vi "test_CRC-32 - Check Protection.vi"(8 "error in (no error)":errorcluster) -> (0 "error out":errorcluster)   [LabVIEW 2023, in "Instrument Addon Protections Unit Tests.lvclass"]
uses:
  Instrument Addon Protections Unit Tests.lvclass
  <vilib>/addons/_JKI Toolkits/VI Tester/TestCase.llb/TestCase.lvclass
  CRC-32/CRC-32.lvclass
panel:
  out "CRC-32 out":refnum<class "CRC-32.lvclass">
  in  "CRC-32 in":refnum<class "CRC-32.lvclass">
  out "TestCase out":refnum<class "Instrument Addon Protections Unit Tests.lvclass">
  in  "TestCase in":refnum<class "Instrument Addon Protections Unit Tests.lvclass">
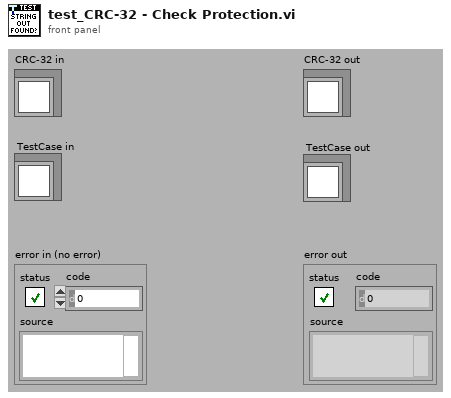
[diagram p1: front panel]
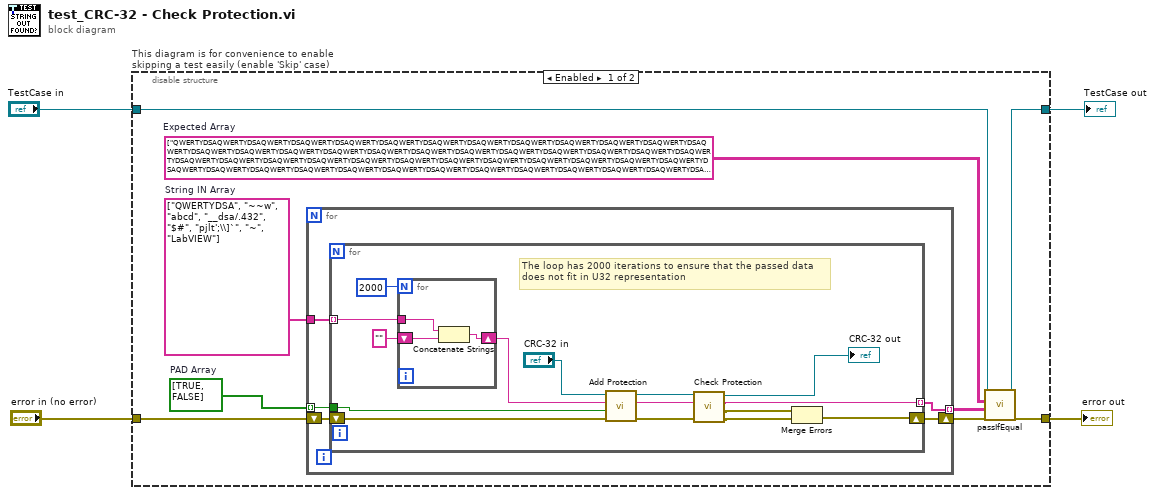
[diagram p0: block diagram]
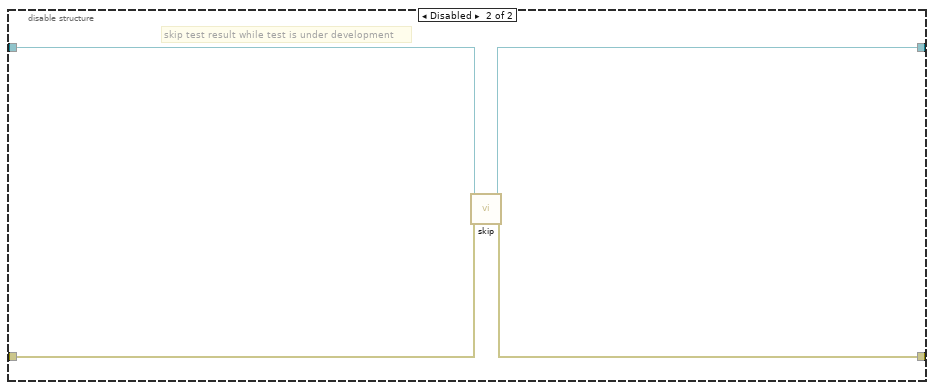
[diagram p2: hidden frame]
diagram:
  n1 = disable-structure "This diagram is for convenience to enable skipping a test easily (enable 'Skip' case)" shown="Enabled" {
    disable-tunnel: "TestCase in" -> [w11 w40]
    disable-tunnel: [w12 w38] -> w1
    disable-tunnel: [w13 w39] -> w3
    disable-tunnel: "error in (no error)" -> [w10 w37]
    frame Enabled {
      w5 = string[][] [["QWERTYDSAQWERTYDSAQWERTYDSAQWERTYDSAQWERTYDSAQWERTYDSAQWERTYDSAQWERTYDSAQWERTYDSAQWERTYDSAQWERTYDSAQWERTYDSAQWERTYDSAQWERTYDSAQWERTYDSAQWERTYDSAQWERTYDSAQWERTYDSAQWERTYDSAQWERTYDSAQWERTYDSAQWERTYDSAQWERTYDSAQWERTYDSAQWERTYDSAQWERTYDSAQWERTYDSAQWERTYDSAQWERTYDSAQWERTYDSAQWERTYDSAQWERTYDSAQWERTYDSAQWERTYDSAQWERTYDSAQWERTYDSAQWERTYDSAQWERTYDSAQWERTYDSAQWERTYDSAQWERTYDSAQWERTYDSAQWERTYDSAQWERTYDSAQWERTYDSAQWERTYDSAQWERTYDSAQWERTYDSAQWERTYDSAQWERTYDSAQWERTYDSAQWERTYDSAQWERTYDSAQWERTYDSAQWERTYDSAQWERTYDSAQWERTYDSAQWERTYDSAQWERTYDSAQWERTYDSAQWERTYDSAQWERTYDSAQWERTYDSAQWERTYDSAQWERTYDSAQWERTYDSAQWERTY...", "~~w~~w~~w~~w~~w~~w~~w~~w~~w~~w~~w~~w~~w~~w~~w~~w~~w~~w~~w~~w~~w~~w~~w~~w~~w~~w~~w~~w~~w~~w~~w~~w~~w~~w~~w~~w~~w~~w~~w~~w~~w~~w~~w~~w~~w~~w~~w~~w~~w~~w~~w~~w~~w~~w~~w~~w~~w~~w~~w~~w~~w~~w~~w~~w~~w~~w~~w~~w~~w~~w~~w~~w~~w~~w~~w~~w~~w~~w~~w~~w~~w~~w~~w~~w~~w~~w~~w~~w~~w~~w~~w~~w~~w~~w~~w~~w~~w~~w~~w~~w~~w~~w~~w~~w~~w~~w~~w~~w~~w~~w~~w~~w~~w~~w~~w~~w~~w~~w~~w~~w~~w~~w~~w~~w~~w~~w~~w~~w~~w~~w~~w~~w~~w~~w~~w~~w~~w~~w~~w~~w~~w~~w~~w~~w~~w~~w~~w~~w~~w~~w~~w~~w~~w~~w~~w~~w~~w~~w~~w~~w~~w~~w~~w~~w~~w~~w~~w~~w~~w~~w~~w~~w~~w~~w~~w~~w~~w~~w~~w~~w~~w~~w~~w~~w~~w~~w~~w~~w~~w~~w~~w~~w~~w~~w~~w~~w~~w~~w~~w~~w~~w~~w~~w~~w~~w~~w~~w~~w~~w~~w~~w~~w~~w~~w~~w~~w~~w~~w~~w~~w~~w~~w~~w~~w~~w~~w~~w~~w~~w~~w~~w~~w~~w~~w~~w~~w~~w~~w~~w~~w~~w~~w~~w~~w~~w~~w~~w~~w~~w~~w~~w~~w~~w~~w~~w~~w~~w~~w~~w~~w~~w~~w~~w~~w~~w~~w~~w~~w~~w~~w~~w~~w~~w~~w~~w~~w~~w~~w~~w~~w~~w~~w~~w~~w~~w~~w~~w~~w~~w~~w~~w~~w~~w~~w~~w~~w~~w~~w~~w~~w~~w~~w~~w~~w~~w~~w~~w~~w~~w~~w~~w~~w~~w~~w~~w~~w~~w~~w~~w~~w~~w~~w~~w~~w~~w~~w~~w~~w~~w~~w~~w~~w~~w~~w~~w~~w~~w~~w~~w~~w~~w~~w~~w~~w~~w~~w~~w~~w~~w~~w~~w~~w~~w~~w~~w~~w~~w~~w~~w~~w~~w~~w~~w~~w~~w~~w~~w~~w~~w~~w~~w~~w~~w~~w~~w~~w~~w~~w~~w~~w~~w~~w~~w~~w~~w~~w~~w~~w~~w~~w~~w~~w~~w~~w~~w~~w~~w~~w~~w~~w~~w~~w~~w~~w~~w~~w~~w~~w~~w~~w~~w~~w~~w~~w~~w~~w~~w~~w~~w~~w~~w~~w~~w~~w~~w~~w~~w~~w~~w~~w~~w~~w~~w~~w~~w~~w~~w~~w~~w~~w~~w~~w~~w~~w~~w~~w~~w~~w~~w~~w~~w~~w~~w~~w~~w~~w~~w~~w~~w~~w~~w~~w~~w~~w~~w~~w~~w~~w~~w~~w~~w~~w~~w~~w~~w~~w~~w~~w~~w~~w~~w~~w~~w~~w~~w~~w~~w~~w~~w~~w~~w~~w~~w~~w~~w~~w~~w~~w~~w~~w~~w~~w~~w~~w~~w~~w~~w~~w~~w~~w~~w~~w~~w~~w~~w~~w~~w~~w~~w~~w~~w~~w~~w~~w~~w~~w~~w~~w~~w~~w~~w~~w~~w~~w~~w~~w~~w~~w~~w~~w~~w~~w~~w~~w~~w~~w~~w~~w~~w~~w~~w~~w~~w~~w~~w~~w~~w~~w~~w~~w~~w~~w~~w~~w~~w~~w~~w~~w~~w~~w~~w~~w~~w~~w~~w~~w~~w~~w~~w~~w~~w~~w~~w~~w~~w~~w~~w~~w~~w~~w~~w~~w~~w~~w~~w~~w~~w~~w~~w~~w~~w~~w~~w~~w~~w~~w~~w~~w~~w~~w~~w~~w~~w~~w~~w~~w~~w~~w~~w~~w~~w~~w~~w~~w~~w~~w~~w~~w~~w~~w~~w~~w~~w~~w~~w~~w~~w~~w~~w~~w~~w~~w~~w~~w~~w~~w~~w~~w~~w~~w~~w~~w~~w~~w~~w~~w~~w~~w~~w~~w~~w~~w~~w~~w~~w~~w~~w~~w~~w~~w~~w~~w~~w~~w~~w~~w~~w~~w~~w~~w~~w~~w~~w~~w~~w~~w~~w~~w~~w~~w~~w~~w~~w~~w~~w~~w~~w~~w~~w~~w~~w~~w~~w~~w~~w~~w~~w~~w~~w~~w~~w~~w~~w~~w~~w~~w~~w~~w~~w~~w~~w~~w~~w~~w~~w~~w~~w~~w~~w~~w~~w~~w~~w~~w~~w~~w~~w~~w~~w~~w~~w~~w~~w~~w~~w~~w~~w~~w~~w~~w~~w~~w~~w~~w~~w~~w~~w~~w~~w~~w~~w~~w~~w~~w~~w~~w~~w~~w~~w~~w~~w~~w~~w~~w~~w~~w~~w~~w~~w~~w~~w~~w~~w~~w~~w~~w~~w~~w~~w~~w~~w~~w~~w~~w~~w~~w~~w~~w~~w~~w~~w~~w~~w~~w~~w~~w~~w~~w~~w~~w~~w~~w~~w~~w~~w~~w~~w~~w~~w~~w~~w~~w~~w~~w~~w~~w~~w~~w~~w~~w~~w~~w~~w~~w~~w~~w~~w~~w~~w~~w~~w~~w~~w~~w~~w~~w~~w~~w~~w~~w~~w~~w~~w~~w~~w~~w~~w~~w~~w~~w~~w~~w~~w~~w~~w~~w~~w~~w~~w~~w~~w~~w~~w~~w~~w~~w~~w~~w~~w~~w~~w~~w~~w~~w~~w~~w~~w~~w~~w~~w~~w~~w~~w~~w~~w~~w~~w~~w~~w~~w~~w~~w~~w~~w~~w~~w~~w~~w~~w~~w~~w~~w~~w~~w~~w~~w~~w~~w~~w~~w~~w~~w~~w~~w~~w~~w~~w~~w~~w~~w~~w~~w~~w~~w~~w~~w~~w~~w~~w~~w~~w~~w~~w~~w~~w~~w~~w~~w~~w~~w~~w~~w~~w~~w~~w~~w~~w~~w~~w~~w~~w~~w~~w~~w~~w~~w~~w~~w~~w~~w~~w~~w~~w~~w~~w~~w~~w~~w~~w~~w~~w~~w~~w~~w~~w~~w~~w~~w~~w~~w~~w~~w~~w~~w~~w~~w~~w~~w~~w~~w~~w~~w~~w~~w~~w~~w~~w~~w~~w~~w~~w~~w~~w~~w~~w~~w~~w~~w~~w~~w~~w~~w~~w~~w~~w~~w~~w~~w~~w~~w~~w~~w~~w~~w~~w~~w~~w~~w~~w~~w~~w~~w~~w~~w~~w~~w~~w~~w~~w~~w~~w~~w~~w~~w~~w~~w~~w~~w~~w~~w~~w~~w~~w~~w~~w~~w~~w~~w~~w~~w~~w~~w~~w~~w~~w~~w~~w~~w~~w~~w~~w~~w~~w~~w~~w~~w~~w~~w~~w~~w~~w~~w~~w~~w~~w~~w~~w~~w~~w~~w~~w~~w~~w~~w~~w~~w~~w~~w~~w~~w~~w~~w~~w~~w~~w~~w~~w~~w~~w~~w~~w~~w~~w~~w~~w~~w~~w~~w~~w~~w~~w~~w~~w~~w~~w~~w~~w~~w~~w~~w~~w~~w~~w~~w~~w~~w~~w~~w~~w~~w~~w~~w~~w~~w~~w~~w~~w~~w~~w~~w~~w~~w~~w~~w~~w~~w~~w~~w~~w~~w~~w~~w~~w~~w~~w~~w~~w~~w~~w~~w~~w~~w~~w~~w~~w~~w~~w~~w~~w~~w~~w~~w~~w~~w~~w~~w~~w~~w~~w~~w~~w~~w~~w~~w~~w~~w~~w~~w~~w~~w~~w~~w~~w~~w~~w~~w~~w~~w~~w~~w~~w~~w~~w~~w~~w~~w~~w~~w~~w~~w~~w~~w~~w~~w~~w~~w~~w~~w~~w~~w~~w~~w~~w~~w~~w~~w~~w~~w~~w~~w~~w~~w~~w~~w~~w~~w~~w~~w~~w~~w~~w~~w~~w~~w~~w~~w~~w~~w~~w~~w~~w~~w~~w~~w~~w~~w~~w~~w~~w~~w~~w~~w~~w~~w~~w~~w~~w~~w~~w~~w~~w~~w~~w~~w~~w~~w~~w~~w~~w~~w~~w~~w~~w~~w~~w~~w~~w~~w~~w~~w~~w~~w~~w~~w~~w~~w~~w~~w~~w~~w~~w~~w~~w~~w~~w~~w~~w~~w~~w~~w~~w~~w~~w~~w~~w~~w~~w~~w~~w~~w~~w~~w~~w~~w~~w~~w~~w~~w~~w~~w~~w~~w~~w~~w~~w~~w~~w~~w~~w~~w~~w~~w~~w~~w~~w~~w~~w~~w~~w~~w~~w~~w~~w~~w~~w~~w~~w~~w~~w~~w~~w~~w~~w~~w~~w~~w~~w~~w~~w~~w~~w~~w~~w~~w~~w~~w~~w~~w~~w~~w~~w~~w~~w~~w~~w~~w~~w~~w~~w~~w~~w~~w~~w~~w~~w~~w~~w~~w~~w~~w~~w~~w~~w~~w~~w~~w~~w~~w~~w~~w~~w~~w~~w~~w~~w~~w~~w~~w~~w~~w~~w~~w~~w~~w~~w~~w~~w~~w~~w~~w~~w~~w~~w~~w~~w~~w~~w~~w~~w~~w~~w~~w~~w~~w~~w~~w~~w~~w~~w~~w~~w~~w~~w~~w~~w~~w~~w~~w~~w~~w~~w~~w~~w~~w~~w~~w~~w~~w~~w~~w~~w~~w~~w~~w~~w~~w~~w~~w~~w~~w~~w~~w~~w~~w~~w~~w~~w~~w~~w~~w~~w~~w~~w~~w~~w~~w~~w~~w~~w~~w~~w~~w~~w~~w~~w~~w~~w~~w~~w~~w~~w~~w~~w~~w~~w~~w~~w~~w~~w~~w~~w~~w~~w~~w~~w~~w~~w~~w~~w~~w~~w~~w~~w~~w~~w~~w~~w~~w~~w~~w~~w~~w~~w~~w~~w~~w~~w~~w~~w~~w~~w~~w~~w~~w~~w~~w~~w~~w~~w~~w~~w~~w~~w~~w~~w~~w~~w~~w~~w~~w~~w~~w~~w~~w~~w~~w~~w~~w~~w~~w~~w~~w~~w~~w~~w~~w~~w~~w~~w~~w~~w~~w~~w~~w~~w~~w~~w~~w~~w~~w~~w~~w~~w~~w~~w~~w~~w~~w~~w~~w~~w~~w~~w~~w~~w~~w~~w~~w~~w~~w~~w~~w~~w~~w~~w~~w~~w~~w~~w~~w~~w~~w~~w~~w~~w~~w~~w~~w~~w~~w~~w~~w~~w~~w~~w~~w~~w~~w~~w~~w~~w~~w~~w~~w~~w~~w~~w~~w~~w~~w~~w~~w~~w~~w~~w~~w~~w~~w~~w~~w~~w~~w~~w~~w~~w~~w~~w~~w~~w~~w~~w~~w~~w~~w~~w~~w~~w~~w~~w~~w~~w~~w~~w~~w~~w~~w~~w~~w~~w~~w~~w~~w~~w~~w~~w~~w~~w~~w~~w~~w~~w~~w~~w~~w~~w~~w~~w~~w~~w~~w~~w~~w~~w~~w~~w~~w~~w~~w~~w~~w~~w~~w~~w~~w~~w~~w~~w~~w~~w~~w~~w~~w~~w~~w~~w~~w~~w~~w~~w~~w~~w~~w~~w~~w~~w~~w~~w~~w~~w~~w~~w~~w~~w~~w~~w~~w~~w~~w~~w~~w~~w~~w~~w~~w~~w~~w~~w~~w~~w~~w~~w~~w~~w~~w~~w~~w~~w~~w~~w~~w~~w~~w~~w~~w~~w~~w~~w~~w~~w~~w~~w~~w~~w~~w~~w~~w~~w~~w~~w~~w~~w~~w~~w~~w~~w~~w~~w~~w~~w~~w~~w~~w~~w~~w~~w~~w~~w~~w~~w~~w~~w~~w~~w~~w~~w~~w~~w~~w~~w~~w~~w~~w~~w~~w~~w~~w~~w~~w~~w~~w~~w~~w~~w~~w~~w~~w~~w~~w~~w~~w~~w~~w~~w~~w~~w~~w~~w~~w~~w~~w~~w~~w~~w~~w~~w~~w~~w~~w~~w~~w~~w~~w~~w~~w~~w~~w~~w~~w~~w~~w~~w~~w~~w~~w~~w~~w~~w~~w~~w~~w~~w~~w~~w~~w~~w~~w~~w~~w~~w~~w~~w~~w~~w~~w~~w~~w~~w~~w~~w~~w~~w~~w~~w~~w~~w~~w~~w~~w~~w~~w~~w~~w~~w~~w~~w~~w~~w~~w~~w~~w~~w~~w~~w~~w~~w~~w~~w~~w~~w~~w~~w~~w~~w~~w~~w~~w~~w~~w~~w~~w~~w~~w~~w~~w~~w~~w~~w~~w~~w~~w~~w~~w~~w~~w~~w~~w~~w~~w~~", "abcdabcdabcdabcdabcdabcdabcdabcdabcdabcdabcdabcdabcdabcdabcdabcdabcdabcdabcdabcdabcdabcdabcdabcdabcdabcdabcdabcdabcdabcdabcdabcdabcdabcdabcdabcdabcdabcdabcdabcdabcdabcdabcdabcdabcdabcdabcdabcdabcdabcdabcdabcdabcdabcdabcdabcdabcdabcdabcdabcdabcdabcdabcdabcdabcdabcdabcdabcdabcdabcdabcdabcdabcdabcdabcdabcdabcdabcdabcdabcdabcdabcdabcdabcdabcdabcdabcdabcdabcdabcdabcdabcdabcdabcdabcdabcdabcdabcdabcdabcdabcdabcdabcdabcdabcdabcdabcdabcdabcdabcdabcdabcdabcdabcdabcdabcdabcdabcdabcdabcdabcdabcdabcdabcdabcdabcdabcdabcdabcdabcdabcdabcdabcdabcdabcdabcdabcdabcdabcdabcdabcdabcdabcdabcdabcdabcdabcdabcdabcdabcd...", "__dsa/.432__dsa/.432__dsa/.432__dsa/.432__dsa/.432__dsa/.432__dsa/.432__dsa/.432__dsa/.432__dsa/.432__dsa/.432__dsa/.432__dsa/.432__dsa/.432__dsa/.432__dsa/.432__dsa/.432__dsa/.432__dsa/.432__dsa/.432__dsa/.432__dsa/.432__dsa/.432__dsa/.432__dsa/.432__dsa/.432__dsa/.432__dsa/.432__dsa/.432__dsa/.432__dsa/.432__dsa/.432__dsa/.432__dsa/.432__dsa/.432__dsa/.432__dsa/.432__dsa/.432__dsa/.432__dsa/.432__dsa/.432__dsa/.432__dsa/.432__dsa/.432__dsa/.432__dsa/.432__dsa/.432__dsa/.432__dsa/.432__dsa/.432__dsa/.432__dsa/.432__dsa/.432__dsa/.432__dsa/.432__dsa/.432__dsa/.432__dsa/.432__dsa/.432__dsa/.432__dsa/.432__dsa/.432__dsa/.432__dsa/.432__dsa/.432__dsa/.432__dsa/.432__dsa/.432__dsa/.432__dsa/.432__dsa/.432__dsa/.432__dsa/.432__dsa/.432__dsa/.432__dsa/.432__dsa/.432__dsa/.432__dsa/.432__dsa/.432__dsa/.432__dsa/.432__dsa/.432__dsa/.432__dsa/.432__dsa/.432__dsa/.432__dsa/.432__dsa/.432__dsa/.432__dsa/.432__dsa/.432__dsa/.432__dsa/.432__dsa/.432__dsa/.432__dsa/.432__dsa/.432__dsa/.432__dsa/.432__dsa/.432__dsa/.432__dsa/.432__dsa/.432__dsa/.432__dsa/.432__dsa/.432__dsa/.432__dsa/.432__dsa/.432__dsa/.432__dsa/.432__dsa/.432__dsa/.432__dsa/.432__dsa/.432__dsa/.432__dsa/.432__dsa/.432__dsa/.432__dsa/.432__dsa/.432__dsa/.432__dsa/.432__dsa/.432__dsa/.432__dsa/.432__dsa/.432__dsa/.432__dsa/.432__dsa/.432__dsa/.432__dsa/.432__dsa/.432__dsa/.432__dsa/.432__dsa/.432__dsa/.432__dsa/.432__dsa/.432__dsa/.432__dsa/.432__dsa/.432__dsa/.432__dsa/.432__dsa/.432__dsa/.432__dsa/.432__dsa/.432__dsa/.432__dsa/.432__dsa/.432__dsa/.432__dsa/.432__dsa/.432__dsa/.432__dsa/.432__dsa/.432__dsa/.432__dsa/.432__dsa/.432__dsa/.432__dsa/.432__dsa/.432__dsa/.432__dsa/.432__dsa/.432__dsa/.432__dsa/.432__dsa/.432__dsa/.432__dsa/.432__dsa/.432__dsa/.432__dsa/.432__dsa/.432__dsa/.432__dsa/.432__dsa/.432__dsa/.432__dsa/.432__dsa/.432__dsa/.432__dsa/.432__dsa/.432__dsa/.432__dsa/.432__dsa/.432__dsa/.432__dsa/.432__dsa/.432__dsa/.432__dsa/.432__dsa/.432__dsa/.432__dsa/.432__dsa/.432__dsa/.432__dsa/.432__dsa/.432__dsa/.432__dsa/.432__dsa/.432__dsa/.432__dsa/.432__dsa/.432__dsa/.432__dsa/.432__dsa/.432__dsa/.432__dsa/.432__dsa/.432__dsa/.432__dsa/.432__dsa/.432__dsa/.432__dsa/.432__dsa/.432__dsa/.432__dsa/.432__dsa/.432__dsa/.432__dsa/.432__dsa/.432__dsa/.432__dsa/.432__dsa/.432__dsa/.432__dsa/.432__dsa/.432__dsa/.432__dsa/.432__dsa/.432__dsa/.432__dsa/.432__dsa/.432__dsa/.432__dsa/.432__dsa/.432__dsa/.432__dsa/.432__dsa/.432__dsa/.432__dsa/.432__dsa/.432__dsa/.432__dsa/.432__dsa/.432__dsa/.432__dsa/.432__dsa/.432__dsa/.432__dsa/.432__dsa/.432__dsa/.432__dsa/.432__dsa/.432__dsa/.432__dsa/.432__dsa/.432__dsa/.432__dsa/.432__dsa/.432__dsa/.432__dsa/.432__dsa/.432__dsa/.432__dsa/.432__dsa/.432__dsa/.432__dsa/.432__dsa/.432__dsa/.432__dsa/.432__dsa/.432__dsa/.432__dsa/.432__dsa/.432__dsa/.432__dsa/.432__dsa/.432__dsa/.432__dsa/.432__dsa/.432__dsa/.432__dsa/.432__dsa/.432__dsa/.432__dsa/.432__dsa/.432__dsa/.432__dsa/.432__dsa/.432__dsa/.432__dsa/.432__dsa/.432__dsa/.432__dsa/.432__dsa/.432__dsa/.432__dsa/.432__dsa/.432__dsa/.432__dsa/.432__dsa/.432__dsa/.432__dsa/.432__dsa/.432__dsa/.432__dsa/.432__dsa/.432__dsa/.432__dsa/.432__dsa/.432__dsa/.432__dsa/.432__dsa/.432__dsa/.432__dsa/.432__dsa/.432__dsa/.432__dsa/.432__dsa/.432__dsa/.432__dsa/.432__dsa/.432__dsa/.432__dsa/.432__dsa/.432__dsa/.432__dsa/.432__dsa/.432__dsa/.432__dsa/.432__dsa/.432__dsa/.432__dsa/.432__dsa/.432__dsa/.432__dsa/.432__dsa/.432__dsa/.432__dsa/.432__dsa/.432__dsa/.432__dsa/.432__dsa/.432__dsa/.432__dsa/.432__dsa/.432__dsa/.432__dsa/.432__dsa/.432__dsa/.432__dsa/.432__dsa/.432__dsa/.432__dsa/.432__dsa/.432__dsa/.432__dsa/.432__dsa/.432__dsa/.432__dsa/.432__dsa/.432__dsa/.432__dsa/.432__dsa/.432__dsa/.432__dsa/.432__dsa/.432__dsa/.432__dsa/.432__dsa/.432__dsa/.432__dsa/.432__dsa/.432__dsa/.432__dsa/.432__dsa/.432__dsa/.432__dsa/.432__dsa/.432__dsa/.432__dsa/.432__dsa/.432__dsa/.432__dsa/.432__dsa/.432__dsa/.432__dsa/.432__dsa/.432__dsa/.432__dsa/.432__dsa/.432__dsa/.432__dsa/.432__dsa/.432__dsa/.432__dsa/.432__dsa/.432__dsa/.432__dsa/.432__dsa/.432__dsa/.432__dsa/.432__dsa/.432__dsa/.432__dsa/.432__dsa/.432__dsa/.432__dsa/.432__dsa/.432__dsa/.432__dsa/.432__dsa/.432__dsa/.432__dsa/.432__dsa/.432__dsa/.432__dsa/.432__dsa/.432__dsa/.432__dsa/.432__dsa/.432__dsa/.432__dsa/.432__dsa/.432__dsa/.432__dsa/.432__dsa/.432__dsa/.432__dsa/.432__dsa/.432__dsa/.432__dsa/.432__dsa/.432__dsa/.432__dsa/.432__dsa/.432__dsa/.432__dsa/.432__dsa/.432__dsa/.432__dsa/.432__dsa/.432__dsa/.432__dsa/.432__dsa/.432__dsa/.432__dsa/.432__dsa/.432__dsa/.432__dsa/.432__dsa/.432__dsa/.432__dsa/.432__dsa/.432__dsa/.432__dsa/.432__dsa/.432__dsa/.432__dsa/.432__dsa/.432__dsa/.432__dsa/.432__dsa/.432__dsa/.432__dsa/.432__dsa/.432__dsa/.432__dsa/.432__dsa/.432__dsa/.432__dsa/.432__dsa/.432__dsa/.432__dsa/.432__dsa/.432__dsa/.432__dsa/.432__dsa/.432__dsa/.432__dsa/.432__dsa/.432__dsa/.432__dsa/.432__dsa/.432__dsa/.432__dsa/.432__dsa/.432__dsa/.432__dsa/.432__dsa/.432__dsa/.432__dsa/.432__dsa/.432__dsa/.432__dsa/.432__dsa/.432__dsa/.432__dsa/.432__dsa/.432__dsa/.432__dsa/.432__dsa/.432__dsa/.432__dsa/.432__dsa/.432__dsa/.432__dsa/.432__dsa/.432__dsa/.432__dsa/.432__dsa/.432__dsa/.432__dsa/.432__dsa/.432__dsa/.432__dsa/.432__dsa/.432__dsa/.432__dsa/.432__dsa/.432__dsa/.432__dsa/.432__dsa/.432__dsa/.432__dsa/.432__dsa/.432__dsa/.432__dsa/.432__dsa/.432__dsa/.432__dsa/.432__dsa/.432__dsa/.432__dsa/.432__dsa/.432__dsa/.432__dsa/.432__dsa/.432__dsa/.432__dsa/.432__dsa/.432__dsa/.432__dsa/.432__dsa/.432__dsa/.432__dsa/.432__dsa/.432__dsa/.432__dsa/.432__dsa/.432__dsa/.432__dsa/.432__dsa/.432__dsa/.432__dsa/.432__dsa/.432__dsa/.432__dsa/.432__dsa/.432__dsa/.432__dsa/.432__dsa/.432__dsa/.432__dsa/.432__dsa/.432__dsa/.432__dsa/.432__dsa/.432__dsa/.432__dsa/.432__dsa/.432__dsa/.432__dsa/.432__dsa/.432__dsa/.432__dsa/.432__dsa/.432__dsa/.432__dsa/.432__dsa/.432__dsa/.432__dsa/.432__dsa/.432__dsa/.432__dsa/.432__dsa/.432__dsa/.432__dsa/.432__dsa/.432__dsa/.432__dsa/.432__dsa/.432__dsa/.432__dsa/.432__dsa/.432__dsa/.432__dsa/.432__dsa/.432__dsa/.432__dsa/.432__dsa/.432__dsa/.432__dsa/.432__dsa/.432__dsa/.432__dsa/.432__dsa/.432__dsa/.432__dsa/.432__dsa/.432__dsa/.432__dsa/.432__dsa/.432__dsa/.432__dsa/.432__dsa/.432__dsa/.432__dsa/.432__dsa/.432__dsa/.432__dsa/.432__dsa/.432__dsa/.432__dsa/.432__dsa/.432__dsa/.432__dsa/.432__dsa/.432__dsa/.432__dsa/.432__dsa/.432__dsa/.432__dsa/.432__dsa/.432__dsa/.432__dsa/.432__dsa/.432__dsa/.432__dsa/.432__dsa/.432__dsa/.432__dsa/.432__dsa/.432__dsa/.432__dsa/.432__dsa/.432__dsa/.432__dsa/.432__dsa/.432__dsa/.432__dsa/.432__dsa/.432__dsa/.432__dsa/.432__dsa/.432__dsa/.432__dsa/.432__dsa/.432__dsa/.432__dsa/.432__dsa/.432__dsa/.432__dsa/.432__dsa/.432__dsa/.432__dsa/.432__dsa/.432__dsa/.432__dsa/.432__dsa/.432__dsa/.432__dsa/.432__dsa/.432__dsa/.432__dsa/.432__dsa/.432__dsa/.432__dsa/.432__dsa/.432__dsa/.432__dsa/.432__dsa/.432__dsa/.432__dsa/.432__dsa/.432__dsa/.432__dsa/.432__dsa/.432__dsa/.432__dsa/.432__dsa/.432__dsa/.432__dsa/.432__dsa/.432__dsa/.432__dsa/.432__dsa/.432__dsa/.432__dsa/.432__dsa/.432__dsa/.432__dsa/.432__dsa/.432__dsa/.432__dsa/.432__dsa/.432__dsa/.432__dsa/.432__dsa/.432__dsa/.432__dsa/.432__dsa/.432__dsa/.432__dsa/.432__dsa/.432__dsa/.432__dsa/.432__dsa/.432__dsa/.432__dsa/.432__dsa/.432__dsa/.432__dsa/.432__dsa/.432__dsa/.432__dsa/.432__dsa/.432__dsa/.432__dsa/.432__dsa/.432__dsa/.432__dsa/.432__dsa/.432__dsa/.432__dsa/.432__dsa/.432__dsa/.432__dsa/.432__dsa/.432__dsa/.432__dsa/.432__dsa/.432__dsa/.432__dsa/.432__dsa/.432__dsa/.432__dsa/.432__dsa/.432__dsa/.432__dsa/.432__dsa/.432__dsa/.432__dsa/.432__dsa/.432__dsa/.432__dsa/.432__dsa/.432__dsa/.432__dsa/.432__dsa/.432__dsa/.432__dsa/.432__dsa/.432__dsa/.432__dsa/.432__dsa/.432__dsa/.432__dsa/.432__dsa/.432__dsa/.432__dsa/.432__dsa/.432__dsa/.432__dsa/.432__dsa/.432__dsa/.432__dsa/.432__dsa/.432__dsa/.432__dsa/.432__dsa/.432__dsa/.432__dsa/.432__dsa/.432__dsa/.432__dsa/.432__dsa/.432__dsa/.432__dsa/.432__dsa/.432__dsa/.432__dsa/.432__dsa/.432__dsa/.432__dsa/.432__dsa/.432__dsa/.432__dsa/.432__dsa/.432__dsa/.432__dsa/.432__dsa/.432__dsa/.432__dsa/.432__dsa/.432__dsa/.432__dsa/.432__dsa/.432__dsa/.432__dsa/.432__dsa/.432__dsa/.432__dsa/.432__dsa/.432__dsa/.432__dsa/.432__dsa/.432__dsa/.432__dsa/.432__dsa/.432__dsa/.432__dsa/.432__dsa/.432__dsa/.432__dsa/.432__dsa/.432__dsa/.432__dsa/.432__dsa/.432__dsa/.432__dsa/.432__dsa/.432__dsa/.432__dsa/.432__dsa/.432__dsa/.432__dsa/.432__dsa/.432__dsa/.432__dsa/.432__dsa/.432__dsa/.432__dsa/.432__dsa/.432__dsa/.432__dsa/.432__dsa/.432__dsa/.432__dsa/.432__dsa/.432__dsa/.432__dsa/.432__dsa/.432__dsa/.432__dsa/.432__dsa/.432__dsa/.432__dsa/.432__dsa/.432__dsa/.432__dsa/.432__dsa/.432__dsa/.432__dsa/.432__dsa/.432__dsa/.432__dsa/.432__dsa/.432__dsa/.432__dsa/.432__dsa/.432__dsa/.432__dsa/.432__dsa/.432__dsa/.432__dsa/.432__dsa/.432__dsa/.432__dsa/.432__dsa/.432__dsa/.432__dsa/.432__dsa/.432__dsa/.432__dsa/.432__dsa/.432__dsa/.432__dsa/.432__dsa/.432__dsa/.432__dsa/.432__dsa/.432__dsa/.432__dsa/.432__dsa/.432__dsa/.432__dsa/.432__dsa/.432__dsa/.432__dsa/.432__dsa/.432__dsa/.432__dsa/.432__dsa/.432__dsa/.432__dsa/.432__dsa/.432__dsa/.432__dsa/.432__dsa/.432__dsa/.432__dsa/.432__dsa/.432__dsa/.432__dsa/.432__dsa/.432__dsa/.432__dsa/.432__dsa/.432__dsa/.432__dsa/.432__dsa/.432__dsa/.432__dsa/.432__dsa/.432__dsa/.432__dsa/.432__dsa/.432__dsa/.432__dsa/.432__dsa/.432__dsa/.432__dsa/.432__dsa/.432__dsa/.432__dsa/.432__dsa/.432__dsa/.432__dsa/.432__dsa/.432__dsa/.432__dsa/.432__dsa/.432__dsa/.432__dsa/.432__dsa/.432__dsa/.432__dsa/.432__dsa/.432__dsa/.432__dsa/.432__dsa/.432__dsa/.432__dsa/.432__dsa/.432__dsa/.432__dsa/.432__dsa/.432__dsa/.432__dsa/.432__dsa/.432__dsa/.432__dsa/.432__dsa/.432__dsa/.432__dsa/.432__dsa/.432__dsa/.432__dsa/.432__dsa/.432__dsa/.432__dsa/.432__dsa/.432__dsa/.432__dsa/.432__dsa/.432__dsa/.432__dsa/.432__dsa/.432__dsa/.432__dsa/.432__dsa/.432__dsa/.432__dsa/.432__dsa/.432__dsa/.432__dsa/.432__dsa/.432__dsa/.432__dsa/.432__dsa/.432__dsa/.432__dsa/.432__dsa/.432__dsa/.432__dsa/.432__dsa/.432__dsa/.432__dsa/.432__dsa/.432__dsa/.432__dsa/.432__dsa/.432__dsa/.432__dsa/.432__dsa/.432__dsa/.432__dsa/.432__dsa/.432__dsa/.432__dsa/.432__dsa/.432__dsa/.432__dsa/.432__dsa/.432__dsa/.432__dsa/.432__dsa/.432__dsa/.432__dsa/.432__dsa/.432__dsa/.432__dsa/.432__dsa/.432__dsa/.432__dsa/.432__dsa/.432__dsa/.432__dsa/.432__dsa/.432__dsa/.432__dsa/.432__dsa/.432__dsa/.432__dsa/.432__dsa/.432__dsa/.432__dsa/.432__dsa/.432__dsa/.432__dsa/.432__dsa/.432__dsa/.432__dsa/.432__dsa/.432__dsa/.432__dsa/.432__dsa/.432__dsa/.432__dsa/.432__dsa/.432__dsa/.432__dsa/.432__dsa/.432__dsa/.432__dsa/.432__dsa/.432__dsa/.432__dsa/.432__dsa/.432__dsa/.432__dsa/.432__dsa/.432__dsa/.432__dsa/.432__dsa/.432__dsa/.432__dsa/.432__dsa/.432__dsa/.432__dsa/.432__dsa/.432__dsa/.432__dsa/.432__dsa/.432__dsa/.432__dsa/.432__dsa/.432__dsa/.432__dsa/.432__dsa/.432__dsa/.432__dsa/.432__dsa/.432__dsa/.432__dsa/.432__dsa/.432__dsa/.432__dsa/.432__dsa/.432__dsa/.432__dsa/.432__dsa/.432__dsa/.432__dsa/.432__dsa/.432__dsa/.432__dsa/.432__dsa/.432__dsa/.432__dsa/.432__dsa/.432__dsa/.432__dsa/.432__dsa/.432__dsa/.432__dsa/.432__dsa/.432__dsa/.432__dsa/.432__dsa/.432__dsa/.432__dsa/.432__dsa/.432__dsa/.432__dsa/.432__dsa/.432__dsa/.432__dsa/.432__dsa/.432__dsa/.432__dsa/.432__dsa/.432__dsa/.432__dsa/.432__dsa/.432__dsa/.432__dsa/.432__dsa/.432__dsa/.432__dsa/.432__dsa/.432__dsa/.432__dsa/.432__dsa/.432__dsa/.432__dsa/.432__dsa/.432__dsa/.432__dsa/.432__dsa/.432__dsa/.432__dsa/.432__dsa/.432__dsa/.432__dsa/.432__dsa/.432__dsa/.432__dsa/.432__dsa/.432__dsa/.432__dsa/.432__dsa/.432__dsa/.432__dsa/.432__dsa/.432__dsa/.432__dsa/.432__dsa/.432__dsa/.432__dsa/.432__dsa/.432__dsa/.432__dsa/.432__dsa/.432__dsa/.432__dsa/.432__dsa/.432__dsa/.432__dsa/.432__dsa/.432__dsa/.432__dsa/.432__dsa/.432__dsa/.432__dsa/.432__dsa/.432__dsa/.432__dsa/.432__dsa/.432__dsa/.432__dsa/.432__dsa/.432__dsa/.432__dsa/.432__dsa/.432__dsa/.432__dsa/.432__dsa/.432__dsa/.432__dsa/.432__dsa/.432__dsa/.432__dsa/.432__dsa/.432__dsa/.432__dsa/.432__dsa/.432__dsa/.432__dsa/.432__dsa/.432__dsa/.432__dsa/.432__dsa/.432__dsa/.432__dsa/.432__dsa/.432__dsa/.432__dsa/.432__dsa/.432__dsa/.432__dsa/.432__dsa/.432__dsa/.432__dsa/.432__dsa/.432__dsa/.432__dsa/.432__dsa/.432__dsa/.432__dsa/.432__dsa/.432__dsa/.432__dsa/.432__dsa/.432__dsa/.432__dsa/.432__dsa/.432__dsa/.432__dsa/.432__dsa/.432__dsa/.432__dsa/.432__dsa/.432__dsa/.432__dsa/.432__dsa/.432__dsa/.432__dsa/.432__dsa/.432__dsa/.432__dsa/.432__dsa/.432__dsa/.432__dsa/.432__dsa/.432__dsa/.432__dsa/.432__dsa/.432__dsa/.432__dsa/.432__dsa/.432__dsa/.432__dsa/.432__dsa/.432__dsa/.432__dsa/.432__dsa/.432__dsa/.432__dsa/.432__dsa/.432__dsa/.432__dsa/.432__dsa/.432__dsa/.432__dsa/.432__dsa/.432__dsa/.432__dsa/.432__dsa/.432__dsa/.432__dsa/.432__dsa/.432__dsa/.432__dsa/.432__dsa/.432__dsa/.432__dsa/.432__dsa/.432__dsa/.432__dsa/.432__dsa/.432__dsa/.432__dsa/.432__dsa/.432__dsa/.432__dsa/.432__dsa/.432__dsa/.432__dsa/.432__dsa/.432__dsa/.432__dsa/.432__dsa/.432__dsa/.432__dsa/.432__dsa/.432__dsa/.432__dsa/.432__dsa/.432__dsa/.432__dsa/.432__dsa/.432__dsa/.432__dsa/.432__dsa/.432__dsa/.432__dsa/.432__dsa/.432__dsa/.432__dsa/.432__dsa/.432__dsa/.432__dsa/.432__dsa/.432__dsa/.432__dsa/.432__dsa/.432__dsa/.432__dsa/.432__dsa/.432__dsa/.432__dsa/.432__dsa/.432__dsa/.432__dsa/.432__dsa/.432__dsa/.432__dsa/.432__dsa/.432__dsa/.432__dsa/.432__dsa/.432__dsa/.432__dsa/.432__dsa/.432__dsa/.432__dsa/.432__dsa/.432__dsa/.432__dsa/.432__dsa/.432__dsa/.432__dsa/.432__dsa/.432__dsa/.432__dsa/.432__dsa/.432__dsa/.432__dsa/.432__dsa/.432__dsa/.432__dsa/.432__dsa/.432__dsa/.432__dsa/.432__dsa/.432__dsa/.432__dsa/.432__dsa/.432__dsa/.432__dsa/.432__dsa/.432__dsa/.432__dsa/.432__dsa/.432__dsa/.432__dsa/.432__dsa/.432__dsa/.432__dsa/.432__dsa/.432__dsa/.432__dsa/.432__dsa/.432__dsa/.432__dsa/.432__dsa/.432__dsa/.432__dsa/.432__dsa/.432__dsa/.432__dsa/.432__dsa/.432__dsa/.432__dsa/.432__dsa/.432__dsa/.432__dsa/.432__dsa/.432__dsa/.432__dsa/.432__dsa/.432__dsa/.432__dsa/.432__dsa/.432__dsa/.432__dsa/.432__dsa/.432__dsa/.432__dsa/.432__dsa/.432__dsa/.432__dsa/.432__dsa/.432__dsa/.432__dsa/.432__dsa/.432__dsa/.432__dsa/.432__dsa/.432__dsa/.432__dsa/.432__dsa/.432__dsa/.432__dsa/.432__dsa/.432__dsa/.432__dsa/.432__dsa/.432__dsa/.432__dsa/.432__dsa/.432__dsa/.432__dsa/.432__dsa/.432__dsa/.432__dsa/.432__dsa/.432__dsa/.432__dsa/.432__dsa/.432__dsa/.432__dsa/.432__dsa/.432__dsa/.432__dsa/.432__dsa/.432__dsa/.432__dsa/.432__dsa/.432__dsa/.432__dsa/.432__dsa/.432__dsa/.432__dsa/.432__dsa/.432__dsa/.432__dsa/.432__dsa/.432__dsa/.432__dsa/.432__dsa/.432__dsa/.432__dsa/.432__dsa/.432__dsa/.432__dsa/.432__dsa/.432__dsa/.432__dsa/.432__dsa/.432__dsa/.432__dsa/.432__dsa/.432__dsa/.432__dsa/.432__dsa/.432__dsa/.432__dsa/.432__dsa/.432__dsa/.432__dsa/.432__dsa/.432__dsa/.432__dsa/.432__dsa/.432__dsa/.432__dsa/.432__dsa/.432__dsa/.432__dsa/.432__dsa/.432__dsa/.432__dsa/.432__dsa/.432__dsa/.432__dsa/.432__dsa/.432__dsa/.432__dsa/.432__dsa/.432__dsa/.432__dsa/.432__dsa/.432__dsa/.432__dsa/.432__dsa/.432__dsa/.432__dsa/.432__dsa/.432__dsa/.432__dsa/.432__dsa/.432__dsa/.432__dsa/.432__dsa/.432__dsa/.432__dsa/.432__dsa/.432__dsa/.432__dsa/.432__dsa/.432__dsa/.432__dsa/.432__dsa/.432__dsa/.432__dsa/.432__dsa/.432__dsa/.432__dsa/.432__dsa/.432__dsa/.432__dsa/.432__dsa/.432__dsa/.432__dsa/.432__dsa/.432__dsa/.432__dsa/.432__dsa/.432__dsa/.432__dsa/.432__dsa/.432__dsa/.432__dsa/.432__dsa/.432__dsa/.432__dsa/.432__dsa/.432__dsa/.432__dsa/.432__dsa/.432__dsa/.432__dsa/.432__dsa/.432__dsa/.432__dsa/.432__dsa/.432__dsa/.432__dsa/.432__dsa/.432__dsa/.432__dsa/.432__dsa/.432__dsa/.432__dsa/.432__dsa/.432__dsa/.432__dsa/.432__dsa/.432__dsa/.432__dsa/.432__dsa/.432__dsa/.432__dsa/.432__dsa/.432__dsa/.432__dsa/.432__dsa/.432__dsa/.432__dsa/.432__dsa/.432__dsa/.432__dsa/.432__dsa/.432__dsa/.432__dsa/.432__dsa/.432__dsa/.432__dsa/.432__dsa/.432__dsa/.432__dsa/.432__dsa/.432__dsa/.432__dsa/.432__dsa/.432__dsa/.432__dsa/.432__dsa/.432__dsa/.432__dsa/.432__dsa/.432__dsa/.432__dsa/.432__dsa/.432__dsa/.432__dsa/.432__dsa/.432__dsa/.432__dsa/.432__dsa/.432__dsa/.432__dsa/.432__dsa/.432__dsa/.432__dsa/.432__dsa/.432__dsa/.432__dsa/.432__dsa/.432__dsa/.432__dsa/.432__dsa/.432__dsa/.432__dsa/.432__dsa/.432__dsa/.432__dsa/.432__dsa/.432__dsa/.432__dsa/.432__dsa/.432__dsa/.432__dsa/.432__dsa/.432__dsa/.432__dsa/.432__dsa/.432__dsa/.432__dsa/.432__dsa/.432__dsa/.432__dsa/.432__dsa/.432__dsa/.432__dsa/.432__dsa/.432__dsa/.432__dsa/.432__dsa/.432__dsa/.432__dsa/.432__dsa/.432__dsa/.432__dsa/.432__dsa/.432__dsa/.432__dsa/.432__dsa/.432__dsa/.432__dsa/.432__dsa/.432__dsa/.432__dsa/.432__dsa/.432__dsa/.432__dsa/.432__dsa/.432__dsa/.432__dsa/.432__dsa/.432__dsa/.432__dsa/.432__dsa/.432__dsa/.432__dsa/.432__dsa/.432__dsa/.432__dsa/.432__dsa/.432__dsa/.432__dsa/.432__dsa/.432__dsa/.432__dsa/.432__dsa/.432__dsa/.432__dsa/.432__dsa/.432__dsa/.432__dsa/.432__dsa/.432__dsa/.432__dsa/.432__dsa/.432__dsa/.432__dsa/.432__dsa/.432__dsa/.432__dsa/.432__dsa/.432__dsa/.432__dsa/.432__dsa/.432__dsa/.432__dsa/.432__dsa/.432__dsa/.432__dsa/.432__dsa/.432__dsa/.432__dsa/.432__dsa/.432__dsa/.432__dsa/.432__dsa/.432__dsa/.432__dsa/.432__dsa/.432__dsa/.432__dsa/.432__dsa/.432__dsa/.432__dsa/.432__dsa/.432__dsa/.432__dsa/.432__dsa/.432__dsa/.432__dsa/.432__dsa/.432__dsa/.432__dsa/.432__dsa/.432__dsa/.432__dsa/.432__dsa/.432__dsa/.432__dsa/.432__dsa/.432__dsa/.432__dsa/.432__dsa/.432__dsa/.432__dsa/.432__dsa/.432__dsa/.432__dsa/.432__dsa/.432__dsa/.432__dsa/.432__dsa/.432__dsa/.432__dsa/.432__dsa/.432__dsa/.432__dsa/.432__dsa/.432__dsa/.432__dsa/.432__dsa/.432__dsa/.432__dsa/.432__dsa/.432__dsa/.432__dsa/.432__dsa/.432__dsa/.432__dsa/.432__dsa/.432__dsa/.432__dsa/.432__dsa/.432__dsa/.432__dsa/.432__dsa/.432__dsa/.432__dsa/.432__dsa/.432__dsa/.432__dsa/.432__dsa/.432__dsa/.432__dsa/.432__dsa/.432__dsa/.432__dsa/.432__dsa/.432__dsa/.432__dsa/.432__dsa/.432__dsa/.432__dsa/.432__dsa/.432__dsa/.432__dsa/.432__dsa/.432__dsa/.432__dsa/.432__dsa/.432__dsa/.432__dsa/.432__dsa/.432__dsa/.432__dsa/.432__dsa/.432__dsa/.432__dsa/.432__dsa/.432__dsa/.432__dsa/.432__dsa/.432__dsa/.432__dsa/.432__dsa/.432__dsa/.432__dsa/.432__dsa/.432__dsa/.432__dsa/.432__dsa/.432__dsa/.432__dsa/.432__dsa/.432__dsa/.432__dsa/.432__dsa/.432__dsa/.432__dsa/.432__dsa/.432__dsa/.432__dsa/.432__dsa/.432__dsa/.432__dsa/.432__dsa/.432__dsa/.432__dsa/.432__dsa/.432__dsa/.432__dsa/.432__dsa/.432__dsa/.432__dsa/.432__dsa/.432__dsa/.432__dsa/.432__dsa/.432__dsa/.432__dsa/.432__dsa/.432__dsa/.432__dsa/.432__dsa/.432__dsa/.432__dsa/.432__dsa/.432__dsa/.432__dsa/.432__dsa/.432__dsa/.432__dsa/.432__dsa/.432__dsa/.432__dsa/.432__dsa/.432__dsa/.432__dsa/.432__dsa/.432__dsa/.432__dsa/.432__dsa/.432__dsa/.432__dsa/.432__dsa/.432__dsa/.432__dsa/.432__dsa/.432__dsa/.432__dsa/.432__dsa/.432__dsa/.432__dsa/.432__dsa/.432__dsa/.432__dsa/.432__dsa/.432__dsa/.432__dsa/.432__dsa/.432__dsa/.432__dsa/.432__dsa/.432__dsa/.432__dsa/.432__dsa/.432__dsa/.432__dsa/.432__dsa/.432__dsa/.432__dsa/.432__dsa/.432__dsa/.432__dsa/.432__dsa/.432__dsa/.432__dsa/.432__dsa/.432__dsa/.432__dsa/.432__dsa/.432__dsa/.432__dsa/.432__dsa/.432__dsa/.432__dsa/.432__dsa/.432__dsa/.432__dsa/.432__dsa/.432__dsa/.432__dsa/.432__dsa/.432__dsa/.432__dsa/.432__dsa/.432__dsa/.432__dsa/.432__dsa/.432__dsa/.432__dsa/.432__dsa/.432__dsa/.432__dsa/.432__dsa/.432__dsa/.432__dsa/.432__dsa/.432__dsa/.432__dsa/.432__dsa/.432__dsa/.432__dsa/.432__dsa/.432__dsa/.432__dsa/.432__dsa/.432__dsa/.432__dsa/.432__dsa/.432__dsa/.432__dsa/.432__dsa/.432__dsa/.432__dsa/.432__dsa/.432__dsa/.432__dsa/.432__dsa/.432__dsa/.432__dsa/.432__dsa/.432__dsa/.432__dsa/.432__dsa/.432__dsa/.432__dsa/.432__dsa/.432__dsa/.432__dsa/.432__dsa/.432__dsa/.432__dsa/.432__dsa/.432__dsa/.432__dsa/.432__dsa/.432__dsa/.432__dsa/.432__dsa/.432__dsa/.432__dsa/.432__dsa/.432__dsa/.432__dsa/.432__dsa/.432__dsa/.432__dsa/.432__dsa/.432__dsa/.432__dsa/.432__dsa/.432__dsa/.432__dsa/.432__dsa/.432__dsa/.432__dsa/.432__dsa/.432__dsa/.432__dsa/.432__dsa/.432__dsa/.432__dsa/.432__dsa/", "$#$#$#$#$#$#$#$#$#$#$#$#$#$#$#$#$#$#$#$#$#$#$#$#$#$#$#$#$#$#$#$#$#$#$#$#$#$#$#$#$#$#$#$#$#$#$#$#$#$#$#$#$#$#$#$#$#$#$#$#$#$#$#$#$#$#$#$#$#$#$#$#$#$#$#$#$#$#$#$#$#$#$#$#$#$#$#$#$#$#$#$#$#$#$#$#$#$#$#$#$#$#$#$#$#$#$#$#$#$#$#$#$#$#$#$#$#$#$#$#$#$#$#$#$#$#$#$#$#$#$#$#$#$#$#$#$#$#$#$#$#$#$#$#$#$#$#$#$#$#$#$#$#$#$#$#$#$#$#$#$#$#$#$#$#$#$#$#$#$#$#$#$#$#$#$#$#$#$#$#$#$#$#$#$#$#$#$#$#$#$#$#$#$#$#$#$#$#$#$#$#$#$#$#$#$#$#$#$#$#$#$#$#$#$#$#$#$#$#$#$#$#$#$#$#$#$#$#$#$#$#$#$#$#$#$#$#$#$#$#$#$#$#$#$#$#$#$#$#$#$#$#$#$#$#$#$#$#$#$#$#$#$#$#$#$#$#$#$#$#$#$#$#$#$#$#$#$#$#$#$#$#$#$#$#$#$#$#$#$#$#$#$#$#$#$#$#$#$#$#$#$#$#$#$#$#$#$#$#$#$#$#$#$#$#$#$#$#$#$#$#$#$#$#$#$#$#$#$#$#$#$#$#$#$#$#$#$#$#$#$#$#$#$#$#$#$#$#$#$#$#$#$#$#$#$#$#$#$#$#$#$#$#$#$#$#$#$#$#$#$#$#$#$#$#$#$#$#$#$#$#$#$#$#$#$#$#$#$#$#$#$#$#$#$#$#$#$#$#$#$#$#$#$#$#$#$#$#$#$#$#$#$#$#$#$#$#$#$#$#$#$#$#$#$#$#$#$#$#$#$#$#$#$#$#$#$#$#$#$#$#$#$#$#$#$#$#$#$#$#$#$#$#$#$#$#$#$#$#$#$#$#$#$#$#$#$#$#$#$#$#$#$#$#$#$#$#$#$#$#$#$#$#$#$#$#$#$#$#$#$#$#$#$#$#$#$#$#$#$#$#$#$#$#$#$#$#$#$#$#$#$#$#$#$#$#$#$#$#$#$#$#$#$#$#$#$#$#$#$#$#$#$#$#$#$#$#$#$#$#$#$#$#$#$#$#$#$#$#$#$#$#$#$#$#$#$#$#$#$#$#$#$#$#$#$#$#$#$#$#$#$#$#$#$#$#$#$#$#$#$#$#$#$#$#$#$#$#$#$#$#$#$#$#$#$#$#$#$#$#$#$#$#$#$#$#$#$#$#$#$#$#$#$#$#$#$#$#$#$#$#$#$#$#$#$#$#$#$#$#$#$#$#$#$#$#$#$#$#$#$#$#$#$#$#$#$#$#$#$#$#$#$#$#$#$#$#$#$#$#$#$#$#$#$#$#$#$#$#$#$#$#$#$#$#$#$#$#$#$#$#$#$#$#$#$#$#$#$#$#$#$#$#$#$#$#$#$#$#$#$#$#$#$#$#$#$#$#$#$#$#$#$#$#$#$#$#$#$#$#$#$#$#$#$#$#$#$#$#$#$#$#$#$#$#$#$#$#$#$#$#$#$#$#$#$#$#$#$#$#$#$#$#$#$#$#$#$#$#$#$#$#$#$#$#$#$#$#$#$#$#$#$#$#$#$#$#$#$#$#$#$#$#$#$#$#$#$#$#$#$#$#$#$#$#$#$#$#$#$#$#$#$#$#$#$#$#$#$#$#$#$#$#$#$#$#$#$#$#$#$#$#$#$#$#$#$#$#$#$#$#$#$#$#$#$#$#$#$#$#$#$#$#$#$#$#$#$#$#$#$#$#$#$#$#$#$#$#$#$#$#$#$#$#$#$#$#$#$#$#$#$#$#$#$#$#$#$#$#$#$#$#$#$#$#$#$#$#$#$#$#$#$#$#$#$#$#$#$#$#$#$#$#$#$#$#$#$#$#$#$#$#$#$#$#$#$#$#$#$#$#$#$#$#$#$#$#$#$#$#$#$#$#$#$#$#$#$#$#$#$#$#$#$#$#$#$#$#$#$#$#$#$#$#$#$#$#$#$#$#$#$#$#$#$#$#$#$#$#$#$#$#$#$#$#$#$#$#$#$#$#$#$#$#$#$#$#$#$#$#$#$#$#$#$#$#$#$#$#$#$#$#$#$#$#$#$#$#$#$#$#$#$#$#$#$#$#$#$#$#$#$#$#$#$#$#$#$#$#$#$#$#$#$#$#$#$#$#$#$#$#$#$#$#$#$#$#$#$#$#$#$#$#$#$#$#$#$#$#$#$#$#$#$#$#$#$#$#$#$#$#$#$#$#$#$#$#$#$#$#$#$#$#$#$#$#$#$#$#$#$#$#$#$#$#$#$#$#$#$#$#$#$#$#$#$#$#$#$#$#$#$#$#$#$#$#$#$#$#$#$#$#$#$#$#$#$#$#$#$#$#$#$#$#$#$#$#$#$#$#$#$#$#$#$#$#$#$#$#$#$#$#$#$#$#$#$#$#$#$#$#$#$#$#$#$#$#$#$#$#$#$#$#$#$#$#$#$#$#$#$#$#$#$#$#$#$#$#$#$#$#$#$#$#$#$#$#$#$#$#$#$#$#$#$#$#$#$#$#$#$#$#$#$#$#$#$#$#$#$#$#$#$#$#$#$#$#$#$#$#$#$#$#$#$#$#$#$#$#$#$#$#$#$#$#$#$#$#$#$#$#$#$#$#$#$#$#$#$#$#$#$#$#$#$#$#$#$#$#$#$#$#$#$#$#$#$#$#$#$#$#$#$#$#$#$#$#$#$#$#$#$#$#$#$#$#$#$#$#$#$#$#$#$#$#$#$#$#$#$#$#$#$#$#$#$#$#$#$#$#$#$#$#$#$#$#$#$#$#$#$#$#$#$#$#$#$#$#$#$#$#$#$#$#$#$#$#$#$#$#$#$#$#$#$#$#$#$#$#$#$#$#$#$#$#$#$#$#$#$#$#$#$#$#$#$#$#$#$#$#$#$#$#$#$#$#$#$#$#$#$#$#$#$#$#$#$#$#$#$#$#$#$#$#$#$#$#$#$#$#$#$#$#$#$#$#$#$#$#$#$#$#$#$#$#$#$#$#$#$#$#$#$#$#$#$#$#$#$#$#$#$#$#$#$#$#$#$#$#$#$#$#$#$#$#$#$#$#$#$#$#$#$#$#$#$#$#$#$#$#$#$#$#$#$#$#$#$#$#$#$#$#$#$#$#$#$#$#$#$#$#$#$#$#$#$#$#$#$#$#$#$#$#$#$#$#$#$#$#$#$#$#$#$#$#$#$#$#$#$#$#$#$#$#$#$#$#$#$#$#$#$#$#$#$#$#$#$#$#$#$#$#$#$#$#$#$#$#$#$#$#$#$#$#$#$#$#$#$#$#$#$#$#$#$#$#$#$#$#$#$#$#$#$#$#$#$#$#$#$#$#$#$#$#$#$#$#$#$#$#$#$#$#$#$#$#$#$#$#$#$#$#$#$#$#$#$#$#$#$#$#$#$#$#$#$#$#$#$#$#$#$#$#$#$#$#$#$#$#$#$#$#$#$#$#$#$#$#$#$#$#$#$#$#$#$#$#$#$#$#$#$#$#$#$#$#$#$#$#$#$#$#$#$#$#$#$#$#$#$#$#$#$#$#$#$#$#$#$#$#$#$#$#$#$#$#$#$#$#$#$#$#$#$#$#$#$#$#$#$#$#$#$#$#$#$#$#$#$#$#$#$#$#$#$#$#$#$#$#$#$#$#$#$#$#$#$#$#$#$#$#$#$#$#$#$#$#$#$#$#$#$#$#$#$#$#$#$#$#$#$#$#$#$#$#$#$#$#$#$#$#$#$#$#$#$#$#$#$#$#$#$#$#$#$#$#$#$#$#$#$#$#$#$#$#$#$#$#$#$#$#$#$#$#$#$#$#$#$#$#$#$#$#$#$#$#$#$#$#$#$#$#$#$#$#$#$#$#$#$#$#$#$#$#$#$#$#$#$#$#$#$#$#$#$#$#$#$#$#$#$#$#$#$#$#$#$#$#$#$#$#$#$#$#$#$#$#$#$#$#$#$#$#$#$#$#$#$#$#$#$#$#$#$#$#$#$#$#$#$#$#$#$#$#$#$#$#$#$#$#$#$#$#$#$#$#$#$#$#$#$#$#$#$#$#$#$#$#$#$#$#$#$#$#$#$#$#$#$#$#$#$#$#$#$#$#$#$#$#$#$#$#$#$#$#$#$#$#$#$#$#$#$#$#$#$#$#$#$#$#$#$#$#$#$#$#$#$#$#$#$#$#$#$#$#$#$#$#$#$#$#$#$#$#$#$#$#$#$#$#$#$#$#$#$#$#$#$#$#$#$#$#$#$#$#$#$#$#", "pjlt';\\]`pjlt';\\]`pjlt';\\]`pjlt';\\]`pjlt';\\]`pjlt';\\]`pjlt';\\]`pjlt';\\]`pjlt';\\]`pjlt';\\]`pjlt';\\]`pjlt';\\]`pjlt';\\]`pjlt';\\]`pjlt';\\]`pjlt';\\]`pjlt';\\]`pjlt';\\]`pjlt';\\]`pjlt';\\]`pjlt';\\]`pjlt';\\]`pjlt';\\]`pjlt';\\]`pjlt';\\]`pjlt';\\]`pjlt';\\]`pjlt';\\]`pjlt';\\]`pjlt';\\]`pjlt';\\]`pjlt';\\]`pjlt';\\]`pjlt';\\]`pjlt';\\]`pjlt';\\]`pjlt';\\]`pjlt';\\]`pjlt';\\]`pjlt';\\]`pjlt';\\]`pjlt';\\]`pjlt';\\]`pjlt';\\]`pjlt';\\]`pjlt';\\]`pjlt';\\]`pjlt';\\]`pjlt';\\]`pjlt';\\]`pjlt';\\]`pjlt';\\]`pjlt';\\]`pjlt';\\]`pjlt';\\]`pjlt';\\]`pjlt';\\]`pjlt';\\]`pjlt';\\]`pjlt';\\]`pjlt';\\]`pjlt';\\]`pjlt';\\]`pjlt';\\]`pjlt';\\]`pjlt';\\]`pjlt';\\]`pjlt';\\]`pjlt';\\]`pjlt';\\]`pjlt';\\]`pjlt';\\]`pjlt';\\]`pjlt';\\]`pjlt';\\]`pjlt';\\]`pjlt';\\]`pjlt';\\]`pjlt';\\]`pjlt';\\]`pjlt';\\]`pjlt';\\]`pjlt';\\]`pjlt';\\]`pjlt';\\]`pjlt';\\]`pjlt';\\]`pjlt';\\]`pjlt';\\]`pjlt';\\]`pjlt';\\]`pjlt';\\]`pjlt';\\]`pjlt';\\]`pjlt';\\]`pjlt';\\]`pjlt';\\]`pjlt';\\]`pjlt';\\]`pjlt';\\]`pjlt';\\]`pjlt';\\]`pjlt';\\]`pjlt';\\]`pjlt';\\]`pjlt';\\]`pjlt';\\]`pjlt';\\]`pjlt';\\]`pjlt';\\]`pjlt';\\]`pjlt';\\]`pjlt';\\]`pjlt';\\]`pjlt';\\]`pjlt';\\]`pjlt';\\]`pjlt';\\]`pjlt';\\]`pjlt';\\]`pjlt';\\]`pjlt';\\]`pjlt';\\]`pjlt';\\]`pjlt';\\]`pjlt';\\]`pjlt';\\]`pjlt';\\]`pjlt';\\]`pjlt';\\]`pjlt';\\]`pjlt';\\]`pjlt';\\]`pjlt';\\]`pjlt';\\]`pjlt';\\]`pjlt';\\]`pjlt';\\]`pjlt';\\]`pjlt';\\]`pjlt';\\]`pjlt';\\]`pjlt';\\]`pjlt';\\]`pjlt';\\]`pjlt';\\]`pjlt';\\]`pjlt';\\]`pjlt';\\]`pjlt';\\]`pjlt';\\]`pjlt';\\]`pjlt';\\]`pjlt';\\]`pjlt';\\]`pjlt';\\]`pjlt';\\]`pjlt';\\]`pjlt';\\]`pjlt';\\]`pjlt';\\]`pjlt';\\]`pjlt';\\]`pjlt';\\]`pjlt';\\]`pjlt';\\]`pjlt';\\]`pjlt';\\]`pjlt';\\]`pjlt';\\]`pjlt';\\]`pjlt';\\]`pjlt';\\]`pjlt';\\]`pjlt';\\]`pjlt';\\]`pjlt';\\]`pjlt';\\]`pjlt';\\]`pjlt';\\]`pjlt';\\]`pjlt';\\]`pjlt';\\]`pjlt';\\]`pjlt';\\]`pjlt';\\]`pjlt';\\]`pjlt';\\]`pjlt';\\]`pjlt';\\]`pjlt';\\]`pjlt';\\]`pjlt';\\]`pjlt';\\]`pjlt';\\]`pjlt';\\]`pjlt';\\]`pjlt';\\]`pjlt';\\]`pjlt';\\]`pjlt';\\]`pjlt';\\]`pjlt';\\]`pjlt';\\]`pjlt';\\]`pjlt';\\]`pjlt';\\]`pjlt';\\]`pjlt';\\]`pjlt';\\]`pjlt';\\]`pjlt';\\]`pjlt';\\]`pjlt';\\]`pjlt';\\]`pjlt';\\]`pjlt';\\]`pjlt';\\]`pjlt';\\]`pjlt';\\]`pjlt';\\]`pjlt';\\]`pjlt';\\]`pjlt';\\]`pjlt';\\]`pjlt';\\]`pjlt';\\]`pjlt';\\]`pjlt';\\]`pjlt';\\]`pjlt';\\]`pjlt';\\]`pjlt';\\]`pjlt';\\]`pjlt';\\]`pjlt';\\]`pjlt';\\]`pjlt';\\]`pjlt';\\]`pjlt';\\]`pjlt';\\]`pjlt';\\]`pjlt';\\]`pjlt';\\]`pjlt';\\]`pjlt';\\]`pjlt';\\]`pjlt';\\]`pjlt';\\]`pjlt';\\]`pjlt';\\]`pjlt';\\]`pjlt';\\]`pjlt';\\]`pjlt';\\]`pjlt';\\]`pjlt';\\]`pjlt';\\]`pjlt';\\]`pjlt';\\]`pjlt';\\]`pjlt';\\]`pjlt';\\]`pjlt';\\]`pjlt';\\]`pjlt';\\]`pjlt';\\]`pjlt';\\]`pjlt';\\]`pjlt';\\]`pjlt';\\]`pjlt';\\]`pjlt';\\]`pjlt';\\]`pjlt';\\]`pjlt';\\]`pjlt';\\]`pjlt';\\]`pjlt';\\]`pjlt';\\]`pjlt';\\]`pjlt';\\]`pjlt';\\]`pjlt';\\]`pjlt';\\]`pjlt';\\]`pjlt';\\]`pjlt';\\]`pjlt';\\]`pjlt';\\]`pjlt';\\]`pjlt';\\]`pjlt';\\]`pjlt';\\]`pjlt';\\]`pjlt';\\]`pjlt';\\]`pjlt';\\]`pjlt';\\]`pjlt';\\]`pjlt';\\]`pjlt';\\]`pjlt';\\]`pjlt';\\]`pjlt';\\]`pjlt';\\]`pjlt';\\]`pjlt';\\]`pjlt';\\]`pjlt';\\]`pjlt';\\]`pjlt';\\]`pjlt';\\]`pjlt';\\]`pjlt';\\]`pjlt';\\]`pjlt';\\]`pjlt';\\]`pjlt';\\]`pjlt';\\]`pjlt';\\]`pjlt';\\]`pjlt';\\]`pjlt';\\]`pjlt';\\]`pjlt';\\]`pjlt';\\]`pjlt';\\]`pjlt';\\]`pjlt';\\]`pjlt';\\]`pjlt';\\]`pjlt';\\]`pjlt';\\]`pjlt';\\]`pjlt';\\]`pjlt';\\]`pjlt';\\]`pjlt';\\]`pjlt';\\]`pjlt';\\]`pjlt';\\]`pjlt';\\]`pjlt';\\]`pjlt';\\]`pjlt';\\]`pjlt';\\]`pjlt';\\]`pjlt';\\]`pjlt';\\]`pjlt';\\]`pjlt';\\]`pjlt';\\]`pjlt';\\]`pjlt';\\]`pjlt';\\]`pjlt';\\]`pjlt';\\]`pjlt';\\]`pjlt';\\]`pjlt';\\]`pjlt';\\]`pjlt';\\]`pjlt';\\]`pjlt';\\]`pjlt';\\]`pjlt';\\]`pjlt';\\]`pjlt';\\]`pjlt';\\]`pjlt';\\]`pjlt';\\]`pjlt';\\]`pjlt';\\]`pjlt';\\]`pjlt';\\]`pjlt';\\]`pjlt';\\]`pjlt';\\]`pjlt';\\]`pjlt';\\]`pjlt';\\]`pjlt';\\]`pjlt';\\]`pjlt';\\]`pjlt';\\]`pjlt';\\]`pjlt';\\]`pjlt';\\]`pjlt';\\]`pjlt';\\]`pjlt';\\]`pjlt';\\]`pjlt';\\]`pjlt';\\]`pjlt';\\]`pjlt';\\]`pjlt';\\]`pjlt';\\]`pjlt';\\]`pjlt';\\]`pjlt';\\]`pjlt';\\]`pjlt';\\]`pjlt';\\]`pjlt';\\]`pjlt';\\]`pjlt';\\]`pjlt';\\]`pjlt';\\]`pjlt';\\]`pjlt';\\]`pjlt';\\]`pjlt';\\]`pjlt';\\]`pjlt';\\]`pjlt';\\]`pjlt';\\]`pjlt';\\]`pjlt';\\]`pjlt';\\]`pjlt';\\]`pjlt';\\]`pjlt';\\]`pjlt';\\]`pjlt';\\]`pjlt';\\]`pjlt';\\]`pjlt';\\]`pjlt';\\]`pjlt';\\]`pjlt';\\]`pjlt';\\]`pjlt';\\]`pjlt';\\]`pjlt';\\]`pjlt';\\]`pjlt';\\]`pjlt';\\]`pjlt';\\]`pjlt';\\]`pjlt';\\]`pjlt';\\]`pjlt';\\]`pjlt';\\]`pjlt';\\]`pjlt';\\]`pjlt';\\]`pjlt';\\]`pjlt';\\]`pjlt';\\]`pjlt';\\]`pjlt';\\]`pjlt';\\]`pjlt';\\]`pjlt';\\]`pjlt';\\]`pjlt';\\]`pjlt';\\]`pjlt';\\]`pjlt';\\]`pjlt';\\]`pjlt';\\]`pjlt';\\]`pjlt';\\]`pjlt';\\]`pjlt';\\]`pjlt';\\]`pjlt';\\]`pjlt';\\]`pjlt';\\]`pjlt';\\]`pjlt';\\]`pjlt';\\]`pjlt';\\]`pjlt';\\]`pjlt';\\]`pjlt';\\]`pjlt';\\]`pjlt';\\]`pjlt';\\]`pjlt';\\]`pjlt';\\]`pjlt';\\]`pjlt';\\]`pjlt';\\]`pjlt';\\]`pjlt';\\]`pjlt';\\]`pjlt';\\]`pjlt';\\]`pjlt';\\]`pjlt';\\]`pjlt';\\]`pjlt';\\]`pjlt';\\]`pjlt';\\]`pjlt';\\]`pjlt';\\]`pjlt';\\]`pjlt';\\]`pjlt';\\]`pjlt';\\]`pjlt';\\]`pjlt';\\]`pjlt';\\]`pjlt';\\]`pjlt';\\]`pjlt';\\]`pjlt';\\]`pjlt';\\]`pjlt';\\]`pjlt';\\]`pjlt';\\]`pjlt';\\]`pjlt';\\]`pjlt';\\]`pjlt';\\]`pjlt';\\]`pjlt';\\]`pjlt';\\]`pjlt';\\]`pjlt';\\]`pjlt';\\]`pjlt';\\]`pjlt';\\]`pjlt';\\]`pjlt';\\]`pjlt';\\]`pjlt';\\]`pjlt';\\]`pjlt';\\]`pjlt';\\]`pjlt';\\]`pjlt';\\]`pjlt';\\]`pjlt';\\]`pjlt';\\]`pjlt';\\]`pjlt';\\]`pjlt';\\]`pjlt';\\]`pjlt';\\]`pjlt';\\]`pjlt';\\]`pjlt';\\]`pjlt';\\]`pjlt';\\]`pjlt';\\]`pjlt';\\]`pjlt';\\]`pjlt';\\]`pjlt';\\]`pjlt';\\]`pjlt';\\]`pjlt';\\]`pjlt';\\]`pjlt';\\]`pjlt';\\]`pjlt';\\]`pjlt';\\]`pjlt';\\]`pjlt';\\]`pjlt';\\]`pjlt';\\]`pjlt';\\]`pjlt';\\]`pjlt';\\]`pjlt';\\]`pjlt';\\]`pjlt';\\]`pjlt';\\]`pjlt';\\]`pjlt';\\]`pjlt';\\]`pjlt';\\]`pjlt';\\]`pjlt';\\]`pjlt';\\]`pjlt';\\]`pjlt';\\]`pjlt';\\]`pjlt';\\]`pjlt';\\]`pjlt';\\]`pjlt';\\]`pjlt';\\]`pjlt';\\]`pjlt';\\]`pjlt';\\]`pjlt';\\]`pjlt';\\]`pjlt';\\]`pjlt';\\]`pjlt';\\]`pjlt';\\]`pjlt';\\]`pjlt';\\]`pjlt';\\]`pjlt';\\]`pjlt';\\]`pjlt';\\]`pjlt';\\]`pjlt';\\]`pjlt';\\]`pjlt';\\]`pjlt';\\]`pjlt';\\]`pjlt';\\]`pjlt';\\]`pjlt';\\]`pjlt';\\]`pjlt';\\]`pjlt';\\]`pjlt';\\]`pjlt';\\]`pjlt';\\]`pjlt';\\]`pjlt';\\]`pjlt';\\]`pjlt';\\]`pjlt';\\]`pjlt';\\]`pjlt';\\]`pjlt';\\]`pjlt';\\]`pjlt';\\]`pjlt';\\]`pjlt';\\]`pjlt';\\]`pjlt';\\]`pjlt';\\]`pjlt';\\]`pjlt';\\]`pjlt';\\]`pjlt';\\]`pjlt';\\]`pjlt';\\]`pjlt';\\]`pjlt';\\]`pjlt';\\]`pjlt';\\]`pjlt';\\]`pjlt';\\]`pjlt';\\]`pjlt';\\]`pjlt';\\]`pjlt';\\]`pjlt';\\]`pjlt';\\]`pjlt';\\]`pjlt';\\]`pjlt';\\]`pjlt';\\]`pjlt';\\]`pjlt';\\]`pjlt';\\]`pjlt';\\]`pjlt';\\]`pjlt';\\]`pjlt';\\]`pjlt';\\]`pjlt';\\]`pjlt';\\]`pjlt';\\]`pjlt';\\]`pjlt';\\]`pjlt';\\]`pjlt';\\]`pjlt';\\]`pjlt';\\]`pjlt';\\]`pjlt';\\]`pjlt';\\]`pjlt';\\]`pjlt';\\]`pjlt';\\]`pjlt';\\]`pjlt';\\]`pjlt';\\]`pjlt';\\]`pjlt';\\]`pjlt';\\]`pjlt';\\]`pjlt';\\]`pjlt';\\]`pjlt';\\]`pjlt';\\]`pjlt';\\]`pjlt';\\]`pjlt';\\]`pjlt';\\]`pjlt';\\]`pjlt';\\]`pjlt';\\]`pjlt';\\]`pjlt';\\]`pjlt';\\]`pjlt';\\]`pjlt';\\]`pjlt';\\]`pjlt';\\]`pjlt';\\]`pjlt';\\]`pjlt';\\]`pjlt';\\]`pjlt';\\]`pjlt';\\]`pjlt';\\]`pjlt';\\]`pjlt';\\]`pjlt';\\]`pjlt';\\]`pjlt';\\]`pjlt';\\]`pjlt';\\]`pjlt';\\]`pjlt';\\]`pjlt';\\]`pjlt';\\]`pjlt';\\]`pjlt';\\]`pjlt';\\]`pjlt';\\]`pjlt';\\]`pjlt';\\]`pjlt';\\]`pjlt';\\]`pjlt';\\]`pjlt';\\]`pjlt';\\]`pjlt';\\]`pjlt';\\]`pjlt';\\]`pjlt';\\]`pjlt';\\]`pjlt';\\]`pjlt';\\]`pjlt';\\]`pjlt';\\]`pjlt';\\]`pjlt';\\]`pjlt';\\]`pjlt';\\]`pjlt';\\]`pjlt';\\]`pjlt';\\]`pjlt';\\]`pjlt';\\]`pjlt';\\]`pjlt';\\]`pjlt';\\]`pjlt';\\]`pjlt';\\]`pjlt';\\]`pjlt';\\]`pjlt';\\]`pjlt';\\]`pjlt';\\]`pjlt';\\]`pjlt';\\]`pjlt';\\]`pjlt';\\]`pjlt';\\]`pjlt';\\]`pjlt';\\]`pjlt';\\]`pjlt';\\]`pjlt';\\]`pjlt';\\]`pjlt';\\]`pjlt';\\]`pjlt';\\]`pjlt';\\]`pjlt';\\]`pjlt';\\]`pjlt';\\]`pjlt';\\]`pjlt';\\]`pjlt';\\]`pjlt';\\]`pjlt';\\]`pjlt';\\]`pjlt';\\]`pjlt';\\]`pjlt';\\]`pjlt';\\]`pjlt';\\]`pjlt';\\]`pjlt';\\]`pjlt';\\]`pjlt';\\]`pjlt';\\]`pjlt';\\]`pjlt';\\]`pjlt';\\]`pjlt';\\]`pjlt';\\]`pjlt';\\]`pjlt';\\]`pjlt';\\]`pjlt';\\]`pjlt';\\]`pjlt';\\]`pjlt';\\]`pjlt';\\]`pjlt';\\]`pjlt';\\]`pjlt';\\]`pjlt';\\]`pjlt';\\]`pjlt';\\]`pjlt';\\]`pjlt';\\]`pjlt';\\]`pjlt';\\]`pjlt';\\]`pjlt';\\]`pjlt';\\]`pjlt';\\]`pjlt';\\]`pjlt';\\]`pjlt';\\]`pjlt';\\]`pjlt';\\]`pjlt';\\]`pjlt';\\]`pjlt';\\]`pjlt';\\]`pjlt';\\]`pjlt';\\]`pjlt';\\]`pjlt';\\]`pjlt';\\]`pjlt';\\]`pjlt';\\]`pjlt';\\]`pjlt';\\]`pjlt';\\]`pjlt';\\]`pjlt';\\]`pjlt';\\]`pjlt';\\]`pjlt';\\]`pjlt';\\]`pjlt';\\]`pjlt';\\]`pjlt';\\]`pjlt';\\]`pjlt';\\]`pjlt';\\]`pjlt';\\]`pjlt';\\]`pjlt';\\]`pjlt';\\]`pjlt';\\]`pjlt';\\]`pjlt';\\]`pjlt';\\]`pjlt';\\]`pjlt';\\]`pjlt';\\]`pjlt';\\]`pjlt';\\]`pjlt';\\]`pjlt';\\]`pjlt';\\]`pjlt';\\]`pjlt';\\]`pjlt';\\]`pjlt';\\]`pjlt';\\]`pjlt';\\]`pjlt';\\]`pjlt';\\]`pjlt';\\]`pjlt';\\]`pjlt';\\]`pjlt';\\]`pjlt';\\]`pjlt';\\]`pjlt';\\]`pjlt';\\]`pjlt';\\]`pjlt';\\]`pjlt';\\]`pjlt';\\]`pjlt';\\]`pjlt';\\]`pjlt';\\]`pjlt';\\]`pjlt';\\]`pjlt';\\]`pjlt';\\]`pjlt';\\]`pjlt';\\]`pjlt';\\]`pjlt';\\]`pjlt';\\]`pjlt';\\]`pjlt';\\]`pjlt';\\]`pjlt';\\]`pjlt';\\]`pjlt';\\]`pjlt';\\]`pjlt';\\]`pjlt';\\]`pjlt';\\]`pjlt';\\]`pjlt';\\]`pjlt';\\]`pjlt';\\]`pjlt';\\]`pjlt';\\]`pjlt';\\]`pjlt';\\]`pjlt';\\]`pjlt';\\]`pjlt';\\]`pjlt';\\]`pjlt';\\]`pjlt';\\]`pjlt';\\]`pjlt';\\]`pjlt';\\]`pjlt';\\]`pjlt';\\]`pjlt';\\]`pjlt';\\]`pjlt';\\]`pjlt';\\]`pjlt';\\]`pjlt';\\]`pjlt';\\]`pjlt';\\]`pjlt';\\]`pjlt';\\]`pjlt';\\]`pjlt';\\]`pjlt';\\]`pjlt';\\]`pjlt';\\]`pjlt';\\]`pjlt';\\]`pjlt';\\]`pjlt';\\]`pjlt';\\]`pjlt';\\]`pjlt';\\]`pjlt';\\]`pjlt';\\]`pjlt';\\]`pjlt';\\]`pjlt';\\]`pjlt';\\]`pjlt';\\]`pjlt';\\]`pjlt';\\]`pjlt';\\]`pjlt';\\]`pjlt';\\]`pjlt';\\]`pjlt';\\]`pjlt';\\]`pjlt';\\]`pjlt';\\]`pjlt';\\]`pjlt';\\]`pjlt';\\]`pjlt';\\]`pjlt';\\]`pjlt';\\]`pjlt';\\]`pjlt';\\]`pjlt';\\]`pjlt';\\]`pjlt';\\]`pjlt';\\]`pjlt';\\]`pjlt';\\]`pjlt';\\]`pjlt';\\]`pjlt';\\]`pjlt';\\]`pjlt';\\]`pjlt';\\]`pjlt';\\]`pjlt';\\]`pjlt';\\]`pjlt';\\]`pjlt';\\]`pjlt';\\]`pjlt';\\]`pjlt';\\]`pjlt';\\]`pjlt';\\]`pjlt';\\]`pjlt';\\]`pjlt';\\]`pjlt';\\]`pjlt';\\]`pjlt';\\]`pjlt';\\]`pjlt';\\]`pjlt';\\]`pjlt';\\]`pjlt';\\]`pjlt';\\]`pjlt';\\]`pjlt';\\]`pjlt';\\]`pjlt';\\]`pjlt';\\]`pjlt';\\]`pjlt';\\]`pjlt';\\]`pjlt';\\]`pjlt';\\]`pjlt';\\]`pjlt';\\]`pjlt';\\]`pjlt';\\]`pjlt';\\]`pjlt';\\]`pjlt';\\]`pjlt';\\]`pjlt';\\]`pjlt';\\]`pjlt';\\]`pjlt';\\]`pjlt';\\]`pjlt';\\]`pjlt';\\]`pjlt';\\]`pjlt';\\]`pjlt';\\]`pjlt';\\]`pjlt';\\]`pjlt';\\]`pjlt';\\]`pjlt';\\]`pjlt';\\]`pjlt';\\]`pjlt';\\]`pjlt';\\]`pjlt';\\]`pjlt';\\]`pjlt';\\]`pjlt';\\]`pjlt';\\]`pjlt';\\]`pjlt';\\]`pjlt';\\]`pjlt';\\]`pjlt';\\]`pjlt';\\]`pjlt';\\]`pjlt';\\]`pjlt';\\]`pjlt';\\]`pjlt';\\]`pjlt';\\]`pjlt';\\]`pjlt';\\]`pjlt';\\]`pjlt';\\]`pjlt';\\]`pjlt';\\]`pjlt';\\]`pjlt';\\]`pjlt';\\]`pjlt';\\]`pjlt';\\]`pjlt';\\]`pjlt';\\]`pjlt';\\]`pjlt';\\]`pjlt';\\]`pjlt';\\]`pjlt';\\]`pjlt';\\]`pjlt';\\]`pjlt';\\]`pjlt';\\]`pjlt';\\]`pjlt';\\]`pjlt';\\]`pjlt';\\]`pjlt';\\]`pjlt';\\]`pjlt';\\]`pjlt';\\]`pjlt';\\]`pjlt';\\]`pjlt';\\]`pjlt';\\]`pjlt';\\]`pjlt';\\]`pjlt';\\]`pjlt';\\]`pjlt';\\]`pjlt';\\]`pjlt';\\]`pjlt';\\]`pjlt';\\]`pjlt';\\]`pjlt';\\]`pjlt';\\]`pjlt';\\]`pjlt';\\]`pjlt';\\]`pjlt';\\]`pjlt';\\]`pjlt';\\]`pjlt';\\]`pjlt';\\]`pjlt';\\]`pjlt';\\]`pjlt';\\]`pjlt';\\]`pjlt';\\]`pjlt';\\]`pjlt';\\]`pjlt';\\]`pjlt';\\]`pjlt';\\]`pjlt';\\]`pjlt';\\]`pjlt';\\]`pjlt';\\]`pjlt';\\]`pjlt';\\]`pjlt';\\]`pjlt';\\]`pjlt';\\]`pjlt';\\]`pjlt';\\]`pjlt';\\]`pjlt';\\]`pjlt';\\]`pjlt';\\]`pjlt';\\]`pjlt';\\]`pjlt';\\]`pjlt';\\]`pjlt';\\]`pjlt';\\]`pjlt';\\]`pjlt';\\]`pjlt';\\]`pjlt';\\]`pjlt';\\]`pjlt';\\]`pjlt';\\]`pjlt';\\]`pjlt';\\]`pjlt';\\]`pjlt';\\]`pjlt';\\]`pjlt';\\]`pjlt';\\]`pjlt';\\]`pjlt';\\]`pjlt';\\]`pjlt';\\]`pjlt';\\]`pjlt';\\]`pjlt';\\]`pjlt';\\]`pjlt';\\]`pjlt';\\]`pjlt';\\]`pjlt';\\]`pjlt';\\]`pjlt';\\]`pjlt';\\]`pjlt';\\]`pjlt';\\]`pjlt';\\]`pjlt';\\]`pjlt';\\]`pjlt';\\]`pjlt';\\]`pjlt';\\]`pjlt';\\]`pjlt';\\]`pjlt';\\]`pjlt';\\]`pjlt';\\]`pjlt';\\]`pjlt';\\]`pjlt';\\]`pjlt';\\]`pjlt';\\]`pjlt';\\]`pjlt';\\]`pjlt';\\]`pjlt';\\]`pjlt';\\]`pjlt';\\]`pjlt';\\]`pjlt';\\]`pjlt';\\]`pjlt';\\]`pjlt';\\]`pjlt';\\]`pjlt';\\]`pjlt';\\]`pjlt';\\]`pjlt';\\]`pjlt';\\]`pjlt';\\]`pjlt';\\]`pjlt';\\]`pjlt';\\]`pjlt';\\]`pjlt';\\]`pjlt';\\]`pjlt';\\]`pjlt';\\]`pjlt';\\]`pjlt';\\]`pjlt';\\]`pjlt';\\]`pjlt';\\]`pjlt';\\]`pjlt';\\]`pjlt';\\]`pjlt';\\]`pjlt';\\]`pjlt';\\]`pjlt';\\]`pjlt';\\]`pjlt';\\]`pjlt';\\]`pjlt';\\]`pjlt';\\]`pjlt';\\]`pjlt';\\]`pjlt';\\]`pjlt';\\]`pjlt';\\]`pjlt';\\]`pjlt';\\]`pjlt';\\]`pjlt';\\]`pjlt';\\]`pjlt';\\]`pjlt';\\]`pjlt';\\]`pjlt';\\]`pjlt';\\]`pjlt';\\]`pjlt';\\]`pjlt';\\]`pjlt';\\]`pjlt';\\]`pjlt';\\]`pjlt';\\]`pjlt';\\]`pjlt';\\]`pjlt';\\]`pjlt';\\]`pjlt';\\]`pjlt';\\]`pjlt';\\]`pjlt';\\]`pjlt';\\]`pjlt';\\]`pjlt';\\]`pjlt';\\]`pjlt';\\]`pjlt';\\]`pjlt';\\]`pjlt';\\]`pjlt';\\]`pjlt';\\]`pjlt';\\]`pjlt';\\]`pjlt';\\]`pjlt';\\]`pjlt';\\]`pjlt';\\]`pjlt';\\]`pjlt';\\]`pjlt';\\]`pjlt';\\]`pjlt';\\]`pjlt';\\]`pjlt';\\]`pjlt';\\]`pjlt';\\]`pjlt';\\]`pjlt';\\]`pjlt';\\]`pjlt';\\]`pjlt';\\]`pjlt';\\]`pjlt';\\]`pjlt';\\]`pjlt';\\]`pjlt';\\]`pjlt';\\]`pjlt';\\]`pjlt';\\]`pjlt';\\]`pjlt';\\]`pjlt';\\]`pjlt';\\]`pjlt';\\]`pjlt';\\]`pjlt';\\]`pjlt';\\]`pjlt';\\]`pjlt';\\]`pjlt';\\]`pjlt';\\]`pjlt';\\]`pjlt';\\]`pjlt';\\]`pjlt';\\]`pjlt';\\]`pjlt';\\]`pjlt';\\]`pjlt';\\]`pjlt';\\]`pjlt';\\]`pjlt';\\]`pjlt';\\]`pjlt';\\]`pjlt';\\]`pjlt';\\]`pjlt';\\]`pjlt';\\]`pjlt';\\]`pjlt';\\]`pjlt';\\]`pjlt';\\]`pjlt';\\]`pjlt';\\]`pjlt';\\]`pjlt';\\]`pjlt';\\]`pjlt';\\]`pjlt';\\]`pjlt';\\]`pjlt';\\]`pjlt';\\]`pjlt';\\]`pjlt';\\]`pjlt';\\]`pjlt';\\]`pjlt';\\]`pjlt';\\]`pjlt';\\]`pjlt';\\]`pjlt';\\]`pjlt';\\]`pjlt';\\]`pjlt';\\]`pjlt';\\]`pjlt';\\]`pjlt';\\]`pjlt';\\]`pjlt';\\]`pjlt';\\]`pjlt';\\]`pjlt';\\]`pjlt';\\]`pjlt';\\]`pjlt';\\]`pjlt';\\]`pjlt';\\]`pjlt';\\]`pjlt';\\]`pjlt';\\]`pjlt';\\]`pjlt';\\]`pjlt';\\]`pjlt';\\]`pjlt';\\]`pjlt';\\]`pjlt';\\]`pjlt';\\]`pjlt';\\]`pjlt';\\]`pjlt';\\]`pjlt';\\]`pjlt';\\]`pjlt';\\]`pjlt';\\]`pjlt';\\]`pjlt';\\]`pjlt';\\]`pjlt';\\]`pjlt';\\]`pjlt';\\]`pjlt';\\]`pjlt';\\]`pjlt';\\]`pjlt';\\]`pjlt';\\]`pjlt';\\]`pjlt';\\]`pjlt';\\]`pjlt';\\]`pjlt';\\]`pjlt';\\]`pjlt';\\]`pjlt';\\]`pjlt';\\]`pjlt';\\]`pjlt';\\]`pjlt';\\]`pjlt';\\]`pjlt';\\]`pjlt';\\]`pjlt';\\]`pjlt';\\]`pjlt';\\]`pjlt';\\]`pjlt';\\]`pjlt';\\]`pjlt';\\]`pjlt';\\]`pjlt';\\]`pjlt';\\]`pjlt';\\]`pjlt';\\]`pjlt';\\]`pjlt';\\]`pjlt';\\]`pjlt';\\]`pjlt';\\]`pjlt';\\]`pjlt';\\]`pjlt';\\]`pjlt';\\]`pjlt';\\]`pjlt';\\]`pjlt';\\]`pjlt';\\]`pjlt';\\]`pjlt';\\]`pjlt';\\]`pjlt';\\]`pjlt';\\]`pjlt';\\]`pjlt';\\]`pjlt';\\]`pjlt';\\]`pjlt';\\]`pjlt';\\]`pjlt';\\]`pjlt';\\]`pjlt';\\]`pjlt';\\]`pjlt';\\]`pjlt';\\]`pjlt';\\]`pjlt';\\]`pjlt';\\]`pjlt';\\]`pjlt';\\]`pjlt';\\]`pjlt';\\]`pjlt';\\]`pjlt';\\]`pjlt';\\]`pjlt';\\]`pjlt';\\]`pjlt';\\]`pjlt';\\]`pjlt';\\]`pjlt';\\]`pjlt';\\]`pjlt';\\]`pjlt';\\]`pjlt';\\]`pjlt';\\]`pjlt';\\]`pjlt';\\]`pjlt';\\]`pjlt';\\]`pjlt';\\]`pjlt';\\]`pjlt';\\]`pjlt';\\]`pjlt';\\]`pjlt';\\]`pjlt';\\]`pjlt';\\]`pjlt';\\]`pjlt';\\]`pjlt';\\]`pjlt';\\]`pjlt';\\]`pjlt';\\]`pjlt';\\]`pjlt';\\]`pjlt';\\]`pjlt';\\]`pjlt';\\]`pjlt';\\]`pjlt';\\]`pjlt';\\]`pjlt';\\]`pjlt';\\]`pjlt';\\]`pjlt';\\]`pjlt';\\]`pjlt';\\]`pjlt';\\]`pjlt';\\]`pjlt';\\]`pjlt';\\]`pjlt';\\]`pjlt';\\]`pjlt';\\]`pjlt';\\]`pjlt';\\]`pjlt';\\]`pjlt';\\]`pjlt';\\]`pjlt';\\]`pjlt';\\]`pjlt';\\]`pjlt';\\]`pjlt';\\]`pjlt';\\]`pjlt';\\]`pjlt';\\]`pjlt';\\]`pjlt';\\]`pjlt';\\]`pjlt';\\]`pjlt';\\]`pjlt';\\]`pjlt';\\]`pjlt';\\]`pjlt';\\]`pjlt';\\]`pjlt';\\]`pjlt';\\]`pjlt';\\]`pjlt';\\]`pjlt';\\]`pjlt';\\]`pjlt';\\]`pjlt';\\]`pjlt';\\]`pjlt';\\]`pjlt';\\]`pjlt';\\]`pjlt';\\]`pjlt';\\]`pjlt';\\]`pjlt';\\]`pjlt';\\]`pjlt';\\]`pjlt';\\]`pjlt';\\]`pjlt';\\]`pjlt';\\]`pjlt';\\]`pjlt';\\]`pjlt';\\]`pjlt';\\]`pjlt';\\]`pjlt';\\]`pjlt';\\]`pjlt';\\]`pjlt';\\]`pjlt';\\]`pjlt';\\]`pjlt';\\]`pjlt';\\]`pjlt';\\]`pjlt';\\]`pjlt';\\]`pjlt';\\]`pjlt';\\]`pjlt';\\]`pjlt';\\]`pjlt';\\]`pjlt';\\]`pjlt';\\]`pjlt';\\]`pjlt';\\]`pjlt';\\]`pjlt';\\]`pjlt';\\]`pjlt';\\]`pjlt';\\]`pjlt';\\]`pjlt';\\]`pjlt';\\]`pjlt';\\]`pjlt';\\]`pjlt';\\]`pjlt';\\]`pjlt';\\]`pjlt';\\]`pjlt';\\]`pjlt';\\]`pjlt';\\]`pjlt';\\]`pjlt';\\]`pjlt';\\]`pjlt';\\]`pjlt';\\]`pjlt';\\]`pjlt';\\]`pjlt';\\]`pjlt';\\]`pjlt';\\]`pjlt';\\]`pjlt';\\]`pjlt';\\]`pjlt';\\]`pjlt';\\]`pjlt';\\]`pjlt';\\]`pjlt';\\]`pjlt';\\]`pjlt';\\]`pjlt';\\]`pjlt';\\]`pjlt';\\]`pjlt';\\]`pjlt';\\]`pjlt';\\]`pjlt';\\]`pjlt';\\]`pjlt';\\]`pjlt';\\]`pjlt';\\]`pjlt';\\]`pjlt';\\]`pjlt';\\]`pjlt';\\]`pjlt';\\]`pjlt';\\]`pjlt';\\]`pjlt';\\]`pjlt';\\]`pjlt';\\]`pjlt';\\]`pjlt';\\]`pjlt';\\]`pjlt';\\]`pjlt';\\]`pjlt';\\]`pjlt';\\]`pjlt';\\]`pjlt';\\]`pjlt';\\]`pjlt';\\]`pjlt';\\]`pjlt';\\]`pjlt';\\]`pjlt';\\]`pjlt';\\]`pjlt';\\]`pjlt';\\]`pjlt';\\]`pjlt';\\]`pjlt';\\]`pjlt';\\]`pjlt';\\]`pjlt';\\]`pjlt';\\]`pjlt';\\]`pjlt';\\]`pjlt';\\]`pjlt';\\]`pjlt';\\]`pjlt';\\]`pjlt';\\]`pjlt';\\]`pjlt';\\]`pjlt';\\]`pjlt';\\]`pjlt';\\]`pjlt';\\]`pjlt';\\]`pjlt';\\]`pjlt';\\]`pjlt';\\]`pjlt';\\]`pjlt';\\]`pjlt';\\]`pjlt';\\]`pjlt';\\]`pjlt';\\]`pjlt';\\]`pjlt';\\]`pjlt';\\]`pjlt';\\]`pjlt';\\]`pjlt';\\]`pjlt';\\]`pjlt';\\]`pjlt';\\]`pjlt';\\]`pjlt';\\]`pjlt';\\]`pjlt';\\]`pjlt';\\]`pjlt';\\]`pjlt';\\]`pjlt';\\]`pjlt';\\]`pjlt';\\]`pjlt';\\]`pjlt';\\]`pjlt';\\]`pjlt';\\]`pjlt';\\]`pjlt';\\]`pjlt';\\]`pjlt';\\]`pjlt';\\]`pjlt';\\]`pjlt';\\]`pjlt';\\]`pjlt';\\]`pjlt';\\]`pjlt';\\]`pjlt';\\]`pjlt';\\]`pjlt';\\]`pjlt';\\]`pjlt';\\]`pjlt';\\]`pjlt';\\]`pjlt';\\]`pjlt';\\]`pjlt';\\]`pjlt';\\]`pjlt';\\]`pjlt';\\]`pjlt';\\]`pjlt';\\]`pjlt';\\]`pjlt';\\]`pjlt';\\]`pjlt';\\]`pjlt';\\]`pjlt';\\]`pjlt';\\]`pjlt';\\]`pjlt';\\]`pjlt';\\]`pjlt';\\]`pjlt';\\]`pjlt';\\]`pjlt';\\]`pjlt';\\]`pjlt';\\]`pjlt';\\]`pjlt';\\]`pjlt';\\]`pjlt';\\]`pjlt';\\]`pjlt';\\]`pjlt';\\]`pjlt';\\]`pjlt';\\]`pjlt';\\]`pjlt';\\]`pjlt';\\]`pjlt';\\]`pjlt';\\]`pjlt';\\]`pjlt';\\]`pjlt';\\]`pjlt';\\]`pjlt';\\]`pjlt';\\]`pjlt';\\]`pjlt';\\]`pjlt';\\]`pjlt';\\]`pjlt';\\]`pjlt';\\]`pjlt';\\]`pjlt';\\]`pjlt';\\]`pjlt';\\]`pjlt';\\]`pjlt';\\]`pjlt';\\]`pjlt';\\]`pjlt';\\]`pjlt';\\]`pjlt';\\]`pjlt';\\]`pjlt';\\]`pjlt';\\]`pjlt';\\]`pjlt';\\]`pjlt';\\]`pjlt';\\]`pjlt';\\]`pjlt';\\]`pjlt';\\]`pjlt';\\]`pjlt';\\]`pjlt';\\]`pjlt';\\]`pjlt';\\]`pjlt';\\]`pjlt';\\]`pjlt';\\]`pjlt';\\]`pjlt';\\]`pjlt';\\]`pjlt';\\]`pjlt';\\]`pjlt';\\]`pjlt';\\]`pjlt';\\]`pjlt';\\]`pjlt';\\]`pjlt';\\]`pjlt';\\]`pjlt';\\]`pjlt';\\]`pjlt';\\]`pjlt';\\]`pjlt';\\]`pjlt';\\]`pjlt';\\]`pjlt';\\]`pjlt';\\]`pjlt';\\]`pjlt';\\]`pjlt';\\]`pjlt';\\]`pjlt';\\]`pjlt';\\]`pjlt';\\]`pjlt';\\]`pjlt';\\]`pjlt';\\]`pjlt';\\]`pjlt';\\]`pjlt';\\]`pjlt';\\]`pjlt';\\]`pjlt';\\]`pjlt';\\]`pjlt';\\]`pjlt';\\]`pjlt';\\]`pjlt';\\]`pjlt';\\]`pjlt';\\]`pjlt';\\]`pjlt';\\]`pjlt';\\]`pjlt';\\]`pjlt';\\]`pjlt';\\]`pjlt';\\]`pjlt';\\]`pjlt';\\]`pjlt';\\]`pjlt';\\]`pjlt';\\]`pjlt';\\]`pjlt';\\]`pjlt';\\]`pjlt';\\]`pjlt';\\]`pjlt';\\]`pjlt';\\]`pjlt';\\]`pjlt';\\]`pjlt';\\]`pjlt';\\]`pjlt';\\]`pjlt';\\]`pjlt';\\]`pjlt';\\]`pjlt';\\]`pjlt';\\]`pjlt';\\]`pjlt';\\]`pjlt';\\]`pjlt';\\]`pjlt';\\]`pjlt';\\]`pjlt';\\]`pjlt';\\]`pjlt';\\]`pjlt';\\]`pjlt';\\]`pjlt';\\]`pjlt';\\]`pjlt';\\]`pjlt';\\]`pjlt';\\]`pjlt';\\]`pjlt';\\]`pjlt';\\]`pjlt';\\]`pjlt';\\]`pjlt';\\]`pjlt';\\]`pjlt';\\]`pjlt';\\]`pjlt';\\]`pjlt';\\]`pjlt';\\]`pjlt';\\]`pjlt';\\]`pjlt';\\]`pjlt';\\]`pjlt';\\]`pjlt';\\]`pjlt';\\]`pjlt';\\]`pjlt';\\]`pjlt';\\]`pjlt';\\]`pjlt';\\]`pjlt';\\]`pjlt';\\]`pjlt';\\]`pjlt';\\]`pjlt';\\]`pjlt';\\]`pjlt';\\]`pjlt';\\]`pjlt';\\]`pjlt';\\]`pjlt';\\]`pjlt';\\]`pjlt';\\]`pjlt';\\]`pjlt';\\]`pjlt';\\]`pjlt';\\]`pjlt';\\]`pjlt';\\]`pjlt';\\]`pjlt';\\]`pjlt';\\]`pjlt';\\]`pjlt';\\]`pjlt';\\]`pjlt';\\]`pjlt';\\]`pjlt';\\]`pjlt';\\]`pjlt';\\]`pjlt';\\]`pjlt';\\]`pjlt';\\]`pjlt';\\]`pjlt';\\]`pjlt';\\]`pjlt';\\]`pjlt';\\]`pjlt';\\]`pjlt';\\]`pjlt';\\]`pjlt';\\]`pjlt';\\]`pjlt';\\]`pjlt';\\]`pjlt';\\]`pjlt';\\]`pjlt';\\]`pjlt';\\]`pjlt';\\]`pjlt';\\]`pjlt';\\]`pjlt';\\]`pjlt';\\]`pjlt';\\]`pjlt';\\]`pjlt';\\]`pjlt';\\]`pjlt';\\]`pjlt';\\]`pjlt';\\]`pjlt';\\]`pjlt';\\]`pjlt';\\]`pjlt';\\]`pjlt';\\]`pjlt';\\]`pjlt';\\]`pjlt';\\]`pjlt';\\]`pjlt'", "~~~~~~~~~~~~~~~~~~~~~~~~~~~~~~~~~~~~~~~~~~~~~~~~~~~~~~~~~~~~~~~~~~~~~~~~~~~~~~~~~~~~~~~~~~~~~~~~~~~~~~~~~~~~~~~~~~~~~~~~~~~~~~~~~~~~~~~~~~~~~~~~~~~~~~~~~~~~~~~~~~~~~~~~~~~~~~~~~~~~~~~~~~~~~~~~~~~~~~~~~~~~~~~~~~~~~~~~~~~~~~~~~~~~~~~~~~~~~~~~~~~~~~~~~~~~~~~~~~~~~~~~~~~~~~~~~~~~~~~~~~~~~~~~~~~~~~~~~~~~~~~~~~~~~~~~~~~~~~~~~~~~~~~~~~~~~~~~~~~~~~~~~~~~~~~~~~~~~~~~~~~~~~~~~~~~~~~~~~~~~~~~~~~~~~~~~~~~~~~~~~~~~~~~~~~~~~~~~~~~~~~~~~~~~~~~~~~~~~~~~~~~~~~~~~~~~~~~~~~~~~~~~~~~~~~~~~~~~~~~~~~~~~~~~~~~~~~~~~~~~~~~~~~~~~~~~~~~~~~~~~~~~~~~~~~~~~~~~~~~~~~~~~~~~~~~~~~~~~~~~~~~~~~~~~~~~~~~~~~~~~~~~~~~~~~~~~~~~~~~~~~~~~~~~~~~~~~~~~~~~~~~~~~~~~~~~~~~~~~~~~~~~~~~~~~~~~~~~~~~~~~~~~~~~~~~~~~~~~~~~~~~~~~~~~~~~~~~~~~~~~~~~~~~~~~~~~~~~~~~~~~~~~~~~~~~~~~~~~~~~~~~~~~~~~~~~~~~~~~~~~~~~~~~~~~~~~~~~~~~~~~~~~~~~~~~~~~~~~~~~~~~~~~~~~~~~~~~~~~~~~~~~~~~~~~~~~~~~~~~~~~~~~~~~~~~~~~~~~~~~~~~~~~~~~~~~~~~~~~~~~~~~~~~~~~~~~~~~~~~~~~~~~~~~~~~~~~~~~~~~~~~~~~~~~~~~~~~~~~~~~~~~~~~~~~~~~~~~~~~~~~~~~~~~~~~~~~~~~~~~~~~~~~~~~~~~~~~~~~~~~~~~~~~~~~~~~~~~~~~~~~~~~~~~~~~~~~~~~~~~~~~~~~~~~~~~~~~~~~~~~~~~~~~~~~~~~~~~~~~~~~~~~~~~~~~~~~~~~~~~~~~~~~~~~~~~~~~~~~~~~~~~~~~~~~~~~~~~~~~~~~~~~~~~~~~~~~~~~~~~~~~~~~~~~~~~~~~~~~~~~~~~~~~~~~~~~~~~~~~~~~~~~~~~~~~~~~~~~~~~~~~~~~~~~~~~~~~~~~~~~~~~~~~~~~~~~~~~~~~~~~~~~~~~~~~~~~~~~~~~~~~~~~~~~~~~~~~~~~~~~~~~~~~~~~~~~~~~~~~~~~~~~~~~~~~~~~~~~~~~~~~~~~~~~~~~~~~~~~~~~~~~~~~~~~~~~~~~~~~~~~~~~~~~~~~~~~~~~~~~~~~~~~~~~~~~~~~~~~~~~~~~~~~~~~~~~~~~~~~~~~~~~~~~~~~~~~~~~~~~~~~~~~~~~~~~~~~~~~~~~~~~~~~~~~~~~~~~~~~~~~~~~~~~~~~~~~~~~~~~~~~~~~~~~~~~~~~~~~~~~~~~~~~~~~~~~~~~~~~~~~~~~~~~~~~~~~~~~~~~~~~~~~~~~~~~~~~~~~~~~~~~~~~~~~~~~~~~~~~~~~~~~~~~~~~~~~~~~~~~~~~~~~~~~~~~~~~~~~~~~~~~~~~~~~~~~~~~~~~~~~~~~~~~~~~~~~~~~~~~~~~~~~~~~~~~~~~~~~~~~~~~~~~~~~~~~~~~~~~~~~~~~~~~~~~~~~~~~~~~~~~~~~~~~~~~~~~~~~~~~~~~~~~~~~~~~~~~~~~~~~~~~~~~~~~~~~~~~~~~~~~~~~~~~~~~~~~~~~~~~~~~~~~~~~~~~~~~~~~~~~~~~~~~~~~~~~~~~~~~~~~~~~~~~~~~~~~~~~~~~~~~~~~~~~~~~~~~~~~~~~~~~~~~~~~~~~~~~~~~~~~~~~~~~~~~~~~~~~~~~~~~~~~~~~~~~~~~~~~~~~~~~~~~~~~~~~~", "LabVIEWLabVIEWLabVIEWLabVIEWLabVIEWLabVIEWLabVIEWLabVIEWLabVIEWLabVIEWLabVIEWLabVIEWLabVIEWLabVIEWLabVIEWLabVIEWLabVIEWLabVIEWLabVIEWLabVIEWLabVIEWLabVIEWLabVIEWLabVIEWLabVIEWLabVIEWLabVIEWLabVIEWLabVIEWLabVIEWLabVIEWLabVIEWLabVIEWLabVIEWLabVIEWLabVIEWLabVIEWLabVIEWLabVIEWLabVIEWLabVIEWLabVIEWLabVIEWLabVIEWLabVIEWLabVIEWLabVIEWLabVIEWLabVIEWLabVIEWLabVIEWLabVIEWLabVIEWLabVIEWLabVIEWLabVIEWLabVIEWLabVIEWLabVIEWLabVIEWLabVIEWLabVIEWLabVIEWLabVIEWLabVIEWLabVIEWLabVIEWLabVIEWLabVIEWLabVIEWLabVIEWLabVIEWLabVIEWLabVIEWLabVIEWLabVIEWLabVIEWLabVIEWLabVIEWLabVIEWLabVIEWLabVIEWLabVIEWLabVIEWLabVIEWLabVI..."], ["QWERTYDSAQWERTYDSAQWERTYDSAQWERTYDSAQWERTYDSAQWERTYDSAQWERTYDSAQWERTYDSAQWERTYDSAQWERTYDSAQWERTYDSAQWERTYDSAQWERTYDSAQWERTYDSAQWERTYDSAQWERTYDSAQWERTYDSAQWERTYDSAQWERTYDSAQWERTYDSAQWERTYDSAQWERTYDSAQWERTYDSAQWERTYDSAQWERTYDSAQWERTYDSAQWERTYDSAQWERTYDSAQWERTYDSAQWERTYDSAQWERTYDSAQWERTYDSAQWERTYDSAQWERTYDSAQWERTYDSAQWERTYDSAQWERTYDSAQWERTYDSAQWERTYDSAQWERTYDSAQWERTYDSAQWERTYDSAQWERTYDSAQWERTYDSAQWERTYDSAQWERTYDSAQWERTYDSAQWERTYDSAQWERTYDSAQWERTYDSAQWERTYDSAQWERTYDSAQWERTYDSAQWERTYDSAQWERTYDSAQWERTYDSAQWERTYDSAQWERTYDSAQWERTYDSAQWERTYDSAQWERTYDSAQWERTYDSAQWERTYDSAQWERTYDSAQWERTYDSAQWERTYDSAQWERTY...", "~~w~~w~~w~~w~~w~~w~~w~~w~~w~~w~~w~~w~~w~~w~~w~~w~~w~~w~~w~~w~~w~~w~~w~~w~~w~~w~~w~~w~~w~~w~~w~~w~~w~~w~~w~~w~~w~~w~~w~~w~~w~~w~~w~~w~~w~~w~~w~~w~~w~~w~~w~~w~~w~~w~~w~~w~~w~~w~~w~~w~~w~~w~~w~~w~~w~~w~~w~~w~~w~~w~~w~~w~~w~~w~~w~~w~~w~~w~~w~~w~~w~~w~~w~~w~~w~~w~~w~~w~~w~~w~~w~~w~~w~~w~~w~~w~~w~~w~~w~~w~~w~~w~~w~~w~~w~~w~~w~~w~~w~~w~~w~~w~~w~~w~~w~~w~~w~~w~~w~~w~~w~~w~~w~~w~~w~~w~~w~~w~~w~~w~~w~~w~~w~~w~~w~~w~~w~~w~~w~~w~~w~~w~~w~~w~~w~~w~~w~~w~~w~~w~~w~~w~~w~~w~~w~~w~~w~~w~~w~~w~~w~~w~~w~~w~~w~~w~~w~~w~~w~~w~~w~~w~~w~~w~~w~~w~~w~~w~~w~~w~~w~~w~~w~~w~~w~~w~~w~~w~~w~~w~~w~~w~~w~~w~~w~~w~~w~~w~~w~~w~~w~~w~~w~~w~~w~~w~~w~~w~~w~~w~~w~~w~~w~~w~~w~~w~~w~~w~~w~~w~~w~~w~~w~~w~~w~~w~~w~~w~~w~~w~~w~~w~~w~~w~~w~~w~~w~~w~~w~~w~~w~~w~~w~~w~~w~~w~~w~~w~~w~~w~~w~~w~~w~~w~~w~~w~~w~~w~~w~~w~~w~~w~~w~~w~~w~~w~~w~~w~~w~~w~~w~~w~~w~~w~~w~~w~~w~~w~~w~~w~~w~~w~~w~~w~~w~~w~~w~~w~~w~~w~~w~~w~~w~~w~~w~~w~~w~~w~~w~~w~~w~~w~~w~~w~~w~~w~~w~~w~~w~~w~~w~~w~~w~~w~~w~~w~~w~~w~~w~~w~~w~~w~~w~~w~~w~~w~~w~~w~~w~~w~~w~~w~~w~~w~~w~~w~~w~~w~~w~~w~~w~~w~~w~~w~~w~~w~~w~~w~~w~~w~~w~~w~~w~~w~~w~~w~~w~~w~~w~~w~~w~~w~~w~~w~~w~~w~~w~~w~~w~~w~~w~~w~~w~~w~~w~~w~~w~~w~~w~~w~~w~~w~~w~~w~~w~~w~~w~~w~~w~~w~~w~~w~~w~~w~~w~~w~~w~~w~~w~~w~~w~~w~~w~~w~~w~~w~~w~~w~~w~~w~~w~~w~~w~~w~~w~~w~~w~~w~~w~~w~~w~~w~~w~~w~~w~~w~~w~~w~~w~~w~~w~~w~~w~~w~~w~~w~~w~~w~~w~~w~~w~~w~~w~~w~~w~~w~~w~~w~~w~~w~~w~~w~~w~~w~~w~~w~~w~~w~~w~~w~~w~~w~~w~~w~~w~~w~~w~~w~~w~~w~~w~~w~~w~~w~~w~~w~~w~~w~~w~~w~~w~~w~~w~~w~~w~~w~~w~~w~~w~~w~~w~~w~~w~~w~~w~~w~~w~~w~~w~~w~~w~~w~~w~~w~~w~~w~~w~~w~~w~~w~~w~~w~~w~~w~~w~~w~~w~~w~~w~~w~~w~~w~~w~~w~~w~~w~~w~~w~~w~~w~~w~~w~~w~~w~~w~~w~~w~~w~~w~~w~~w~~w~~w~~w~~w~~w~~w~~w~~w~~w~~w~~w~~w~~w~~w~~w~~w~~w~~w~~w~~w~~w~~w~~w~~w~~w~~w~~w~~w~~w~~w~~w~~w~~w~~w~~w~~w~~w~~w~~w~~w~~w~~w~~w~~w~~w~~w~~w~~w~~w~~w~~w~~w~~w~~w~~w~~w~~w~~w~~w~~w~~w~~w~~w~~w~~w~~w~~w~~w~~w~~w~~w~~w~~w~~w~~w~~w~~w~~w~~w~~w~~w~~w~~w~~w~~w~~w~~w~~w~~w~~w~~w~~w~~w~~w~~w~~w~~w~~w~~w~~w~~w~~w~~w~~w~~w~~w~~w~~w~~w~~w~~w~~w~~w~~w~~w~~w~~w~~w~~w~~w~~w~~w~~w~~w~~w~~w~~w~~w~~w~~w~~w~~w~~w~~w~~w~~w~~w~~w~~w~~w~~w~~w~~w~~w~~w~~w~~w~~w~~w~~w~~w~~w~~w~~w~~w~~w~~w~~w~~w~~w~~w~~w~~w~~w~~w~~w~~w~~w~~w~~w~~w~~w~~w~~w~~w~~w~~w~~w~~w~~w~~w~~w~~w~~w~~w~~w~~w~~w~~w~~w~~w~~w~~w~~w~~w~~w~~w~~w~~w~~w~~w~~w~~w~~w~~w~~w~~w~~w~~w~~w~~w~~w~~w~~w~~w~~w~~w~~w~~w~~w~~w~~w~~w~~w~~w~~w~~w~~w~~w~~w~~w~~w~~w~~w~~w~~w~~w~~w~~w~~w~~w~~w~~w~~w~~w~~w~~w~~w~~w~~w~~w~~w~~w~~w~~w~~w~~w~~w~~w~~w~~w~~w~~w~~w~~w~~w~~w~~w~~w~~w~~w~~w~~w~~w~~w~~w~~w~~w~~w~~w~~w~~w~~w~~w~~w~~w~~w~~w~~w~~w~~w~~w~~w~~w~~w~~w~~w~~w~~w~~w~~w~~w~~w~~w~~w~~w~~w~~w~~w~~w~~w~~w~~w~~w~~w~~w~~w~~w~~w~~w~~w~~w~~w~~w~~w~~w~~w~~w~~w~~w~~w~~w~~w~~w~~w~~w~~w~~w~~w~~w~~w~~w~~w~~w~~w~~w~~w~~w~~w~~w~~w~~w~~w~~w~~w~~w~~w~~w~~w~~w~~w~~w~~w~~w~~w~~w~~w~~w~~w~~w~~w~~w~~w~~w~~w~~w~~w~~w~~w~~w~~w~~w~~w~~w~~w~~w~~w~~w~~w~~w~~w~~w~~w~~w~~w~~w~~w~~w~~w~~w~~w~~w~~w~~w~~w~~w~~w~~w~~w~~w~~w~~w~~w~~w~~w~~w~~w~~w~~w~~w~~w~~w~~w~~w~~w~~w~~w~~w~~w~~w~~w~~w~~w~~w~~w~~w~~w~~w~~w~~w~~w~~w~~w~~w~~w~~w~~w~~w~~w~~w~~w~~w~~w~~w~~w~~w~~w~~w~~w~~w~~w~~w~~w~~w~~w~~w~~w~~w~~w~~w~~w~~w~~w~~w~~w~~w~~w~~w~~w~~w~~w~~w~~w~~w~~w~~w~~w~~w~~w~~w~~w~~w~~w~~w~~w~~w~~w~~w~~w~~w~~w~~w~~w~~w~~w~~w~~w~~w~~w~~w~~w~~w~~w~~w~~w~~w~~w~~w~~w~~w~~w~~w~~w~~w~~w~~w~~w~~w~~w~~w~~w~~w~~w~~w~~w~~w~~w~~w~~w~~w~~w~~w~~w~~w~~w~~w~~w~~w~~w~~w~~w~~w~~w~~w~~w~~w~~w~~w~~w~~w~~w~~w~~w~~w~~w~~w~~w~~w~~w~~w~~w~~w~~w~~w~~w~~w~~w~~w~~w~~w~~w~~w~~w~~w~~w~~w~~w~~w~~w~~w~~w~~w~~w~~w~~w~~w~~w~~w~~w~~w~~w~~w~~w~~w~~w~~w~~w~~w~~w~~w~~w~~w~~w~~w~~w~~w~~w~~w~~w~~w~~w~~w~~w~~w~~w~~w~~w~~w~~w~~w~~w~~w~~w~~w~~w~~w~~w~~w~~w~~w~~w~~w~~w~~w~~w~~w~~w~~w~~w~~w~~w~~w~~w~~w~~w~~w~~w~~w~~w~~w~~w~~w~~w~~w~~w~~w~~w~~w~~w~~w~~w~~w~~w~~w~~w~~w~~w~~w~~w~~w~~w~~w~~w~~w~~w~~w~~w~~w~~w~~w~~w~~w~~w~~w~~w~~w~~w~~w~~w~~w~~w~~w~~w~~w~~w~~w~~w~~w~~w~~w~~w~~w~~w~~w~~w~~w~~w~~w~~w~~w~~w~~w~~w~~w~~w~~w~~w~~w~~w~~w~~w~~w~~w~~w~~w~~w~~w~~w~~w~~w~~w~~w~~w~~w~~w~~w~~w~~w~~w~~w~~w~~w~~w~~w~~w~~w~~w~~w~~w~~w~~w~~w~~w~~w~~w~~w~~w~~w~~w~~w~~w~~w~~w~~w~~w~~w~~w~~w~~w~~w~~w~~w~~w~~w~~w~~w~~w~~w~~w~~w~~w~~w~~w~~w~~w~~w~~w~~w~~w~~w~~w~~w~~w~~w~~w~~w~~w~~w~~w~~w~~w~~w~~w~~w~~w~~w~~w~~w~~w~~w~~w~~w~~w~~w~~w~~w~~w~~w~~w~~w~~w~~w~~w~~w~~w~~w~~w~~w~~w~~w~~w~~w~~w~~w~~w~~w~~w~~w~~w~~w~~w~~w~~w~~w~~w~~w~~w~~w~~w~~w~~w~~w~~w~~w~~w~~w~~w~~w~~w~~w~~w~~w~~w~~w~~w~~w~~w~~w~~w~~w~~w~~w~~w~~w~~w~~w~~w~~w~~w~~w~~w~~w~~w~~w~~w~~w~~w~~w~~w~~w~~w~~w~~w~~w~~w~~w~~w~~w~~w~~w~~w~~w~~w~~w~~w~~w~~w~~w~~w~~w~~w~~w~~w~~w~~w~~w~~w~~w~~w~~w~~w~~w~~w~~w~~w~~w~~w~~w~~w~~w~~w~~w~~w~~w~~w~~w~~w~~w~~w~~w~~w~~w~~w~~w~~w~~w~~w~~w~~w~~w~~w~~w~~w~~w~~w~~w~~w~~w~~w~~w~~w~~w~~w~~w~~w~~w~~w~~w~~w~~w~~w~~w~~w~~w~~w~~w~~w~~w~~w~~w~~w~~w~~w~~w~~w~~w~~w~~w~~w~~w~~w~~w~~w~~w~~w~~w~~w~~w~~w~~w~~w~~w~~w~~w~~w~~w~~w~~w~~w~~w~~w~~w~~w~~w~~w~~w~~w~~w~~w~~w~~w~~w~~w~~w~~w~~w~~w~~w~~w~~w~~w~~w~~w~~w~~w~~w~~w~~w~~w~~w~~w~~w~~w~~w~~w~~w~~w~~w~~w~~w~~w~~w~~w~~w~~w~~w~~w~~w~~w~~w~~w~~w~~w~~w~~w~~w~~w~~w~~w~~w~~w~~w~~w~~w~~w~~w~~w~~w~~w~~w~~w~~w~~w~~w~~w~~w~~w~~w~~w~~w~~w~~w~~w~~w~~w~~w~~w~~w~~w~~w~~w~~w~~w~~w~~w~~w~~w~~w~~w~~w~~w~~w~~w~~w~~w~~w~~w~~w~~w~~w~~w~~w~~w~~w~~w~~w~~w~~w~~w~~w~~w~~w~~w~~w~~w~~w~~w~~w~~w~~w~~w~~w~~w~~w~~w~~w~~w~~w~~w~~w~~w~~w~~w~~w~~w~~w~~w~~w~~w~~w~~w~~w~~w~~w~~w~~w~~w~~w~~w~~w~~w~~w~~w~~w~~w~~w~~w~~w~~w~~w~~w~~w~~w~~w~~w~~w~~w~~w~~w~~w~~w~~w~~w~~w~~w~~w~~w~~w~~w~~w~~w~~w~~w~~w~~w~~w~~w~~w~~w~~w~~w~~w~~w~~w~~w~~w~~w~~w~~w~~w~~w~~w~~w~~w~~w~~w~~w~~w~~w~~w~~w~~w~~w~~w~~w~~w~~w~~w~~w~~w~~w~~w~~w~~w~~w~~w~~w~~w~~w~~w~~w~~w~~w~~w~~w~~w~~w~~w~~w~~w~~w~~w~~w~~w~~w~~w~~w~~w~~w~~w~~w~~w~~w~~w~~w~~w~~w~~w~~w~~w~~w~~w~~w~~w~~w~~w~~w~~w~~w~~w~~w~~w~~w~~w~~w~~w~~w~~w~~w~~w~~w~~w~~w~~w~~w~~w~~w~~w~~w~~w~~w~~w~~w~~w~~w~~w~~w~~w~~w~~w~~w~~w~~w~~w~~w~~w~~w~~w~~w~~w~~w~~w~~w~~w~~w~~w~~w~~w~~w~~w~~w~~w~~w~~w~~w~~w~~w~~w~~w~~w~~w~~w~~w~~w~~w~~w~~w~~w~~w~~w~~w~~w~~w~~w~~w~~w~~w~~w~~w~~w~~w~~w~~w~~w~~w~~w~~w~~w~~w~~w~~w~~w~~w~~w~~w~~w~~w~~w~~w~~w~~w~~w~~w~~w~~w~~w~~w~~w~~w~~w~~w~~w~~w~~w~~w~~w~~w~~w~~w~~w~~w~~w~~w~~w~~w~~w~~w~~w~~w~~w~~w~~w~~w~~w~~w~~w~~w~~w~~w~~w~~w~~w~~w~~w~~w~~w~~w~~w~~w~~w~~w~~w~~w~~w~~w~~w~~w~~w~~w", "abcdabcdabcdabcdabcdabcdabcdabcdabcdabcdabcdabcdabcdabcdabcdabcdabcdabcdabcdabcdabcdabcdabcdabcdabcdabcdabcdabcdabcdabcdabcdabcdabcdabcdabcdabcdabcdabcdabcdabcdabcdabcdabcdabcdabcdabcdabcdabcdabcdabcdabcdabcdabcdabcdabcdabcdabcdabcdabcdabcdabcdabcdabcdabcdabcdabcdabcdabcdabcdabcdabcdabcdabcdabcdabcdabcdabcdabcdabcdabcdabcdabcdabcdabcdabcdabcdabcdabcdabcdabcdabcdabcdabcdabcdabcdabcdabcdabcdabcdabcdabcdabcdabcdabcdabcdabcdabcdabcdabcdabcdabcdabcdabcdabcdabcdabcdabcdabcdabcdabcdabcdabcdabcdabcdabcdabcdabcdabcdabcdabcdabcdabcdabcdabcdabcdabcdabcdabcdabcdabcdabcdabcdabcdabcdabcdabcdabcdabcdabcdabcd...", "__dsa/.432__dsa/.432__dsa/.432__dsa/.432__dsa/.432__dsa/.432__dsa/.432__dsa/.432__dsa/.432__dsa/.432__dsa/.432__dsa/.432__dsa/.432__dsa/.432__dsa/.432__dsa/.432__dsa/.432__dsa/.432__dsa/.432__dsa/.432__dsa/.432__dsa/.432__dsa/.432__dsa/.432__dsa/.432__dsa/.432__dsa/.432__dsa/.432__dsa/.432__dsa/.432__dsa/.432__dsa/.432__dsa/.432__dsa/.432__dsa/.432__dsa/.432__dsa/.432__dsa/.432__dsa/.432__dsa/.432__dsa/.432__dsa/.432__dsa/.432__dsa/.432__dsa/.432__dsa/.432__dsa/.432__dsa/.432__dsa/.432__dsa/.432__dsa/.432__dsa/.432__dsa/.432__dsa/.432__dsa/.432__dsa/.432__dsa/.432__dsa/.432__dsa/.432__dsa/.432__dsa/.432__dsa/.432__dsa/.432__dsa/.432__dsa/.432__dsa/.432__dsa/.432__dsa/.432__dsa/.432__dsa/.432__dsa/.432__dsa/.432__dsa/.432__dsa/.432__dsa/.432__dsa/.432__dsa/.432__dsa/.432__dsa/.432__dsa/.432__dsa/.432__dsa/.432__dsa/.432__dsa/.432__dsa/.432__dsa/.432__dsa/.432__dsa/.432__dsa/.432__dsa/.432__dsa/.432__dsa/.432__dsa/.432__dsa/.432__dsa/.432__dsa/.432__dsa/.432__dsa/.432__dsa/.432__dsa/.432__dsa/.432__dsa/.432__dsa/.432__dsa/.432__dsa/.432__dsa/.432__dsa/.432__dsa/.432__dsa/.432__dsa/.432__dsa/.432__dsa/.432__dsa/.432__dsa/.432__dsa/.432__dsa/.432__dsa/.432__dsa/.432__dsa/.432__dsa/.432__dsa/.432__dsa/.432__dsa/.432__dsa/.432__dsa/.432__dsa/.432__dsa/.432__dsa/.432__dsa/.432__dsa/.432__dsa/.432__dsa/.432__dsa/.432__dsa/.432__dsa/.432__dsa/.432__dsa/.432__dsa/.432__dsa/.432__dsa/.432__dsa/.432__dsa/.432__dsa/.432__dsa/.432__dsa/.432__dsa/.432__dsa/.432__dsa/.432__dsa/.432__dsa/.432__dsa/.432__dsa/.432__dsa/.432__dsa/.432__dsa/.432__dsa/.432__dsa/.432__dsa/.432__dsa/.432__dsa/.432__dsa/.432__dsa/.432__dsa/.432__dsa/.432__dsa/.432__dsa/.432__dsa/.432__dsa/.432__dsa/.432__dsa/.432__dsa/.432__dsa/.432__dsa/.432__dsa/.432__dsa/.432__dsa/.432__dsa/.432__dsa/.432__dsa/.432__dsa/.432__dsa/.432__dsa/.432__dsa/.432__dsa/.432__dsa/.432__dsa/.432__dsa/.432__dsa/.432__dsa/.432__dsa/.432__dsa/.432__dsa/.432__dsa/.432__dsa/.432__dsa/.432__dsa/.432__dsa/.432__dsa/.432__dsa/.432__dsa/.432__dsa/.432__dsa/.432__dsa/.432__dsa/.432__dsa/.432__dsa/.432__dsa/.432__dsa/.432__dsa/.432__dsa/.432__dsa/.432__dsa/.432__dsa/.432__dsa/.432__dsa/.432__dsa/.432__dsa/.432__dsa/.432__dsa/.432__dsa/.432__dsa/.432__dsa/.432__dsa/.432__dsa/.432__dsa/.432__dsa/.432__dsa/.432__dsa/.432__dsa/.432__dsa/.432__dsa/.432__dsa/.432__dsa/.432__dsa/.432__dsa/.432__dsa/.432__dsa/.432__dsa/.432__dsa/.432__dsa/.432__dsa/.432__dsa/.432__dsa/.432__dsa/.432__dsa/.432__dsa/.432__dsa/.432__dsa/.432__dsa/.432__dsa/.432__dsa/.432__dsa/.432__dsa/.432__dsa/.432__dsa/.432__dsa/.432__dsa/.432__dsa/.432__dsa/.432__dsa/.432__dsa/.432__dsa/.432__dsa/.432__dsa/.432__dsa/.432__dsa/.432__dsa/.432__dsa/.432__dsa/.432__dsa/.432__dsa/.432__dsa/.432__dsa/.432__dsa/.432__dsa/.432__dsa/.432__dsa/.432__dsa/.432__dsa/.432__dsa/.432__dsa/.432__dsa/.432__dsa/.432__dsa/.432__dsa/.432__dsa/.432__dsa/.432__dsa/.432__dsa/.432__dsa/.432__dsa/.432__dsa/.432__dsa/.432__dsa/.432__dsa/.432__dsa/.432__dsa/.432__dsa/.432__dsa/.432__dsa/.432__dsa/.432__dsa/.432__dsa/.432__dsa/.432__dsa/.432__dsa/.432__dsa/.432__dsa/.432__dsa/.432__dsa/.432__dsa/.432__dsa/.432__dsa/.432__dsa/.432__dsa/.432__dsa/.432__dsa/.432__dsa/.432__dsa/.432__dsa/.432__dsa/.432__dsa/.432__dsa/.432__dsa/.432__dsa/.432__dsa/.432__dsa/.432__dsa/.432__dsa/.432__dsa/.432__dsa/.432__dsa/.432__dsa/.432__dsa/.432__dsa/.432__dsa/.432__dsa/.432__dsa/.432__dsa/.432__dsa/.432__dsa/.432__dsa/.432__dsa/.432__dsa/.432__dsa/.432__dsa/.432__dsa/.432__dsa/.432__dsa/.432__dsa/.432__dsa/.432__dsa/.432__dsa/.432__dsa/.432__dsa/.432__dsa/.432__dsa/.432__dsa/.432__dsa/.432__dsa/.432__dsa/.432__dsa/.432__dsa/.432__dsa/.432__dsa/.432__dsa/.432__dsa/.432__dsa/.432__dsa/.432__dsa/.432__dsa/.432__dsa/.432__dsa/.432__dsa/.432__dsa/.432__dsa/.432__dsa/.432__dsa/.432__dsa/.432__dsa/.432__dsa/.432__dsa/.432__dsa/.432__dsa/.432__dsa/.432__dsa/.432__dsa/.432__dsa/.432__dsa/.432__dsa/.432__dsa/.432__dsa/.432__dsa/.432__dsa/.432__dsa/.432__dsa/.432__dsa/.432__dsa/.432__dsa/.432__dsa/.432__dsa/.432__dsa/.432__dsa/.432__dsa/.432__dsa/.432__dsa/.432__dsa/.432__dsa/.432__dsa/.432__dsa/.432__dsa/.432__dsa/.432__dsa/.432__dsa/.432__dsa/.432__dsa/.432__dsa/.432__dsa/.432__dsa/.432__dsa/.432__dsa/.432__dsa/.432__dsa/.432__dsa/.432__dsa/.432__dsa/.432__dsa/.432__dsa/.432__dsa/.432__dsa/.432__dsa/.432__dsa/.432__dsa/.432__dsa/.432__dsa/.432__dsa/.432__dsa/.432__dsa/.432__dsa/.432__dsa/.432__dsa/.432__dsa/.432__dsa/.432__dsa/.432__dsa/.432__dsa/.432__dsa/.432__dsa/.432__dsa/.432__dsa/.432__dsa/.432__dsa/.432__dsa/.432__dsa/.432__dsa/.432__dsa/.432__dsa/.432__dsa/.432__dsa/.432__dsa/.432__dsa/.432__dsa/.432__dsa/.432__dsa/.432__dsa/.432__dsa/.432__dsa/.432__dsa/.432__dsa/.432__dsa/.432__dsa/.432__dsa/.432__dsa/.432__dsa/.432__dsa/.432__dsa/.432__dsa/.432__dsa/.432__dsa/.432__dsa/.432__dsa/.432__dsa/.432__dsa/.432__dsa/.432__dsa/.432__dsa/.432__dsa/.432__dsa/.432__dsa/.432__dsa/.432__dsa/.432__dsa/.432__dsa/.432__dsa/.432__dsa/.432__dsa/.432__dsa/.432__dsa/.432__dsa/.432__dsa/.432__dsa/.432__dsa/.432__dsa/.432__dsa/.432__dsa/.432__dsa/.432__dsa/.432__dsa/.432__dsa/.432__dsa/.432__dsa/.432__dsa/.432__dsa/.432__dsa/.432__dsa/.432__dsa/.432__dsa/.432__dsa/.432__dsa/.432__dsa/.432__dsa/.432__dsa/.432__dsa/.432__dsa/.432__dsa/.432__dsa/.432__dsa/.432__dsa/.432__dsa/.432__dsa/.432__dsa/.432__dsa/.432__dsa/.432__dsa/.432__dsa/.432__dsa/.432__dsa/.432__dsa/.432__dsa/.432__dsa/.432__dsa/.432__dsa/.432__dsa/.432__dsa/.432__dsa/.432__dsa/.432__dsa/.432__dsa/.432__dsa/.432__dsa/.432__dsa/.432__dsa/.432__dsa/.432__dsa/.432__dsa/.432__dsa/.432__dsa/.432__dsa/.432__dsa/.432__dsa/.432__dsa/.432__dsa/.432__dsa/.432__dsa/.432__dsa/.432__dsa/.432__dsa/.432__dsa/.432__dsa/.432__dsa/.432__dsa/.432__dsa/.432__dsa/.432__dsa/.432__dsa/.432__dsa/.432__dsa/.432__dsa/.432__dsa/.432__dsa/.432__dsa/.432__dsa/.432__dsa/.432__dsa/.432__dsa/.432__dsa/.432__dsa/.432__dsa/.432__dsa/.432__dsa/.432__dsa/.432__dsa/.432__dsa/.432__dsa/.432__dsa/.432__dsa/.432__dsa/.432__dsa/.432__dsa/.432__dsa/.432__dsa/.432__dsa/.432__dsa/.432__dsa/.432__dsa/.432__dsa/.432__dsa/.432__dsa/.432__dsa/.432__dsa/.432__dsa/.432__dsa/.432__dsa/.432__dsa/.432__dsa/.432__dsa/.432__dsa/.432__dsa/.432__dsa/.432__dsa/.432__dsa/.432__dsa/.432__dsa/.432__dsa/.432__dsa/.432__dsa/.432__dsa/.432__dsa/.432__dsa/.432__dsa/.432__dsa/.432__dsa/.432__dsa/.432__dsa/.432__dsa/.432__dsa/.432__dsa/.432__dsa/.432__dsa/.432__dsa/.432__dsa/.432__dsa/.432__dsa/.432__dsa/.432__dsa/.432__dsa/.432__dsa/.432__dsa/.432__dsa/.432__dsa/.432__dsa/.432__dsa/.432__dsa/.432__dsa/.432__dsa/.432__dsa/.432__dsa/.432__dsa/.432__dsa/.432__dsa/.432__dsa/.432__dsa/.432__dsa/.432__dsa/.432__dsa/.432__dsa/.432__dsa/.432__dsa/.432__dsa/.432__dsa/.432__dsa/.432__dsa/.432__dsa/.432__dsa/.432__dsa/.432__dsa/.432__dsa/.432__dsa/.432__dsa/.432__dsa/.432__dsa/.432__dsa/.432__dsa/.432__dsa/.432__dsa/.432__dsa/.432__dsa/.432__dsa/.432__dsa/.432__dsa/.432__dsa/.432__dsa/.432__dsa/.432__dsa/.432__dsa/.432__dsa/.432__dsa/.432__dsa/.432__dsa/.432__dsa/.432__dsa/.432__dsa/.432__dsa/.432__dsa/.432__dsa/.432__dsa/.432__dsa/.432__dsa/.432__dsa/.432__dsa/.432__dsa/.432__dsa/.432__dsa/.432__dsa/.432__dsa/.432__dsa/.432__dsa/.432__dsa/.432__dsa/.432__dsa/.432__dsa/.432__dsa/.432__dsa/.432__dsa/.432__dsa/.432__dsa/.432__dsa/.432__dsa/.432__dsa/.432__dsa/.432__dsa/.432__dsa/.432__dsa/.432__dsa/.432__dsa/.432__dsa/.432__dsa/.432__dsa/.432__dsa/.432__dsa/.432__dsa/.432__dsa/.432__dsa/.432__dsa/.432__dsa/.432__dsa/.432__dsa/.432__dsa/.432__dsa/.432__dsa/.432__dsa/.432__dsa/.432__dsa/.432__dsa/.432__dsa/.432__dsa/.432__dsa/.432__dsa/.432__dsa/.432__dsa/.432__dsa/.432__dsa/.432__dsa/.432__dsa/.432__dsa/.432__dsa/.432__dsa/.432__dsa/.432__dsa/.432__dsa/.432__dsa/.432__dsa/.432__dsa/.432__dsa/.432__dsa/.432__dsa/.432__dsa/.432__dsa/.432__dsa/.432__dsa/.432__dsa/.432__dsa/.432__dsa/.432__dsa/.432__dsa/.432__dsa/.432__dsa/.432__dsa/.432__dsa/.432__dsa/.432__dsa/.432__dsa/.432__dsa/.432__dsa/.432__dsa/.432__dsa/.432__dsa/.432__dsa/.432__dsa/.432__dsa/.432__dsa/.432__dsa/.432__dsa/.432__dsa/.432__dsa/.432__dsa/.432__dsa/.432__dsa/.432__dsa/.432__dsa/.432__dsa/.432__dsa/.432__dsa/.432__dsa/.432__dsa/.432__dsa/.432__dsa/.432__dsa/.432__dsa/.432__dsa/.432__dsa/.432__dsa/.432__dsa/.432__dsa/.432__dsa/.432__dsa/.432__dsa/.432__dsa/.432__dsa/.432__dsa/.432__dsa/.432__dsa/.432__dsa/.432__dsa/.432__dsa/.432__dsa/.432__dsa/.432__dsa/.432__dsa/.432__dsa/.432__dsa/.432__dsa/.432__dsa/.432__dsa/.432__dsa/.432__dsa/.432__dsa/.432__dsa/.432__dsa/.432__dsa/.432__dsa/.432__dsa/.432__dsa/.432__dsa/.432__dsa/.432__dsa/.432__dsa/.432__dsa/.432__dsa/.432__dsa/.432__dsa/.432__dsa/.432__dsa/.432__dsa/.432__dsa/.432__dsa/.432__dsa/.432__dsa/.432__dsa/.432__dsa/.432__dsa/.432__dsa/.432__dsa/.432__dsa/.432__dsa/.432__dsa/.432__dsa/.432__dsa/.432__dsa/.432__dsa/.432__dsa/.432__dsa/.432__dsa/.432__dsa/.432__dsa/.432__dsa/.432__dsa/.432__dsa/.432__dsa/.432__dsa/.432__dsa/.432__dsa/.432__dsa/.432__dsa/.432__dsa/.432__dsa/.432__dsa/.432__dsa/.432__dsa/.432__dsa/.432__dsa/.432__dsa/.432__dsa/.432__dsa/.432__dsa/.432__dsa/.432__dsa/.432__dsa/.432__dsa/.432__dsa/.432__dsa/.432__dsa/.432__dsa/.432__dsa/.432__dsa/.432__dsa/.432__dsa/.432__dsa/.432__dsa/.432__dsa/.432__dsa/.432__dsa/.432__dsa/.432__dsa/.432__dsa/.432__dsa/.432__dsa/.432__dsa/.432__dsa/.432__dsa/.432__dsa/.432__dsa/.432__dsa/.432__dsa/.432__dsa/.432__dsa/.432__dsa/.432__dsa/.432__dsa/.432__dsa/.432__dsa/.432__dsa/.432__dsa/.432__dsa/.432__dsa/.432__dsa/.432__dsa/.432__dsa/.432__dsa/.432__dsa/.432__dsa/.432__dsa/.432__dsa/.432__dsa/.432__dsa/.432__dsa/.432__dsa/.432__dsa/.432__dsa/.432__dsa/.432__dsa/.432__dsa/.432__dsa/.432__dsa/.432__dsa/.432__dsa/.432__dsa/.432__dsa/.432__dsa/.432__dsa/.432__dsa/.432__dsa/.432__dsa/.432__dsa/.432__dsa/.432__dsa/.432__dsa/.432__dsa/.432__dsa/.432__dsa/.432__dsa/.432__dsa/.432__dsa/.432__dsa/.432__dsa/.432__dsa/.432__dsa/.432__dsa/.432__dsa/.432__dsa/.432__dsa/.432__dsa/.432__dsa/.432__dsa/.432__dsa/.432__dsa/.432__dsa/.432__dsa/.432__dsa/.432__dsa/.432__dsa/.432__dsa/.432__dsa/.432__dsa/.432__dsa/.432__dsa/.432__dsa/.432__dsa/.432__dsa/.432__dsa/.432__dsa/.432__dsa/.432__dsa/.432__dsa/.432__dsa/.432__dsa/.432__dsa/.432__dsa/.432__dsa/.432__dsa/.432__dsa/.432__dsa/.432__dsa/.432__dsa/.432__dsa/.432__dsa/.432__dsa/.432__dsa/.432__dsa/.432__dsa/.432__dsa/.432__dsa/.432__dsa/.432__dsa/.432__dsa/.432__dsa/.432__dsa/.432__dsa/.432__dsa/.432__dsa/.432__dsa/.432__dsa/.432__dsa/.432__dsa/.432__dsa/.432__dsa/.432__dsa/.432__dsa/.432__dsa/.432__dsa/.432__dsa/.432__dsa/.432__dsa/.432__dsa/.432__dsa/.432__dsa/.432__dsa/.432__dsa/.432__dsa/.432__dsa/.432__dsa/.432__dsa/.432__dsa/.432__dsa/.432__dsa/.432__dsa/.432__dsa/.432__dsa/.432__dsa/.432__dsa/.432__dsa/.432__dsa/.432__dsa/.432__dsa/.432__dsa/.432__dsa/.432__dsa/.432__dsa/.432__dsa/.432__dsa/.432__dsa/.432__dsa/.432__dsa/.432__dsa/.432__dsa/.432__dsa/.432__dsa/.432__dsa/.432__dsa/.432__dsa/.432__dsa/.432__dsa/.432__dsa/.432__dsa/.432__dsa/.432__dsa/.432__dsa/.432__dsa/.432__dsa/.432__dsa/.432__dsa/.432__dsa/.432__dsa/.432__dsa/.432__dsa/.432__dsa/.432__dsa/.432__dsa/.432__dsa/.432__dsa/.432__dsa/.432__dsa/.432__dsa/.432__dsa/.432__dsa/.432__dsa/.432__dsa/.432__dsa/.432__dsa/.432__dsa/.432__dsa/.432__dsa/.432__dsa/.432__dsa/.432__dsa/.432__dsa/.432__dsa/.432__dsa/.432__dsa/.432__dsa/.432__dsa/.432__dsa/.432__dsa/.432__dsa/.432__dsa/.432__dsa/.432__dsa/.432__dsa/.432__dsa/.432__dsa/.432__dsa/.432__dsa/.432__dsa/.432__dsa/.432__dsa/.432__dsa/.432__dsa/.432__dsa/.432__dsa/.432__dsa/.432__dsa/.432__dsa/.432__dsa/.432__dsa/.432__dsa/.432__dsa/.432__dsa/.432__dsa/.432__dsa/.432__dsa/.432__dsa/.432__dsa/.432__dsa/.432__dsa/.432__dsa/.432__dsa/.432__dsa/.432__dsa/.432__dsa/.432__dsa/.432__dsa/.432__dsa/.432__dsa/.432__dsa/.432__dsa/.432__dsa/.432__dsa/.432__dsa/.432__dsa/.432__dsa/.432__dsa/.432__dsa/.432__dsa/.432__dsa/.432__dsa/.432__dsa/.432__dsa/.432__dsa/.432__dsa/.432__dsa/.432__dsa/.432__dsa/.432__dsa/.432__dsa/.432__dsa/.432__dsa/.432__dsa/.432__dsa/.432__dsa/.432__dsa/.432__dsa/.432__dsa/.432__dsa/.432__dsa/.432__dsa/.432__dsa/.432__dsa/.432__dsa/.432__dsa/.432__dsa/.432__dsa/.432__dsa/.432__dsa/.432__dsa/.432__dsa/.432__dsa/.432__dsa/.432__dsa/.432__dsa/.432__dsa/.432__dsa/.432__dsa/.432__dsa/.432__dsa/.432__dsa/.432__dsa/.432__dsa/.432__dsa/.432__dsa/.432__dsa/.432__dsa/.432__dsa/.432__dsa/.432__dsa/.432__dsa/.432__dsa/.432__dsa/.432__dsa/.432__dsa/.432__dsa/.432__dsa/.432__dsa/.432__dsa/.432__dsa/.432__dsa/.432__dsa/.432__dsa/.432__dsa/.432__dsa/.432__dsa/.432__dsa/.432__dsa/.432__dsa/.432__dsa/.432__dsa/.432__dsa/.432__dsa/.432__dsa/.432__dsa/.432__dsa/.432__dsa/.432__dsa/.432__dsa/.432__dsa/.432__dsa/.432__dsa/.432__dsa/.432__dsa/.432__dsa/.432__dsa/.432__dsa/.432__dsa/.432__dsa/.432__dsa/.432__dsa/.432__dsa/.432__dsa/.432__dsa/.432__dsa/.432__dsa/.432__dsa/.432__dsa/.432__dsa/.432__dsa/.432__dsa/.432__dsa/.432__dsa/.432__dsa/.432__dsa/.432__dsa/.432__dsa/.432__dsa/.432__dsa/.432__dsa/.432__dsa/.432__dsa/.432__dsa/.432__dsa/.432__dsa/.432__dsa/.432__dsa/.432__dsa/.432__dsa/.432__dsa/.432__dsa/.432__dsa/.432__dsa/.432__dsa/.432__dsa/.432__dsa/.432__dsa/.432__dsa/.432__dsa/.432__dsa/.432__dsa/.432__dsa/.432__dsa/.432__dsa/.432__dsa/.432__dsa/.432__dsa/.432__dsa/.432__dsa/.432__dsa/.432__dsa/.432__dsa/.432__dsa/.432__dsa/.432__dsa/.432__dsa/.432__dsa/.432__dsa/.432__dsa/.432__dsa/.432__dsa/.432__dsa/.432__dsa/.432__dsa/.432__dsa/.432__dsa/.432__dsa/.432__dsa/.432__dsa/.432__dsa/.432__dsa/.432__dsa/.432__dsa/.432__dsa/.432__dsa/.432__dsa/.432__dsa/.432__dsa/.432__dsa/.432__dsa/.432__dsa/.432__dsa/.432__dsa/.432__dsa/.432__dsa/.432__dsa/.432__dsa/.432__dsa/.432__dsa/.432__dsa/.432__dsa/.432__dsa/.432__dsa/.432__dsa/.432__dsa/.432__dsa/.432__dsa/.432__dsa/.432__dsa/.432__dsa/.432__dsa/.432__dsa/.432__dsa/.432__dsa/.432__dsa/.432__dsa/.432__dsa/.432__dsa/.432__dsa/.432__dsa/.432__dsa/.432__dsa/.432__dsa/.432__dsa/.432__dsa/.432__dsa/.432__dsa/.432__dsa/.432__dsa/.432__dsa/.432__dsa/.432__dsa/.432__dsa/.432__dsa/.432__dsa/.432__dsa/.432__dsa/.432__dsa/.432__dsa/.432__dsa/.432__dsa/.432__dsa/.432__dsa/.432__dsa/.432__dsa/.432__dsa/.432__dsa/.432__dsa/.432__dsa/.432__dsa/.432__dsa/.432__dsa/.432__dsa/.432__dsa/.432__dsa/.432__dsa/.432__dsa/.432__dsa/.432__dsa/.432__dsa/.432__dsa/.432__dsa/.432__dsa/.432__dsa/.432__dsa/.432__dsa/.432__dsa/.432__dsa/.432__dsa/.432__dsa/.432__dsa/.432__dsa/.432__dsa/.432__dsa/.432__dsa/.432__dsa/.432__dsa/.432__dsa/.432__dsa/.432__dsa/.432__dsa/.432__dsa/.432__dsa/.432__dsa/.432__dsa/.432__dsa/.432__dsa/.432__dsa/.432__dsa/.432__dsa/.432__dsa/.432__dsa/.432__dsa/.432__dsa/.432__dsa/.432__dsa/.432__dsa/.432__dsa/.432__dsa/.432__dsa/.432__dsa/.432__dsa/.432__dsa/.432__dsa/.432__dsa/.432__dsa/.432__dsa/.432__dsa/.432__dsa/.432__dsa/.432__dsa/.432__dsa/.432__dsa/.432__dsa/.432__dsa/.432__dsa/.432__dsa/.432__dsa/.432__dsa/.432__dsa/.432__dsa/.432__dsa/.432__dsa/.432__dsa/.432__dsa/.432__dsa/.432__dsa/.432__dsa/.432__dsa/.432__dsa/.432__dsa/.432__dsa/.432__dsa/.432__dsa/.432__dsa/.432__dsa/.432__dsa/.432__dsa/.432__dsa/.432__dsa/.432__dsa/.432__dsa/.432__dsa/.432__dsa/.432__dsa/.432__dsa/.432__dsa/.432__dsa/.432__dsa/.432__dsa/.432__dsa/.432__dsa/.432__dsa/.432__dsa/.432__dsa/.432__dsa/.432__dsa/.432__dsa/.432__dsa/.432__dsa/.432__dsa/.432__dsa/.432__dsa/.432__dsa/.432__dsa/.432__dsa/.432__dsa/.432__dsa/.432__dsa/.432__dsa/.432__dsa/.432__dsa/.432__dsa/.432__dsa/.432__dsa/.432__dsa/.432__dsa/.432__dsa/.432__dsa/.432__dsa/.432__dsa/.432__dsa/.432__dsa/.432__dsa/.432__dsa/.432__dsa/.432__dsa/.432__dsa/.432__dsa/.432__dsa/.432__dsa/.432__dsa/.432__dsa/.432__dsa/.432__dsa/.432__dsa/.432__dsa/.432__dsa/.432__dsa/.432__dsa/.432__dsa/.432__dsa/.432__dsa/.432__dsa/.432__dsa/.432__dsa/.432__dsa/.432__dsa/.432__dsa/.432__dsa/.432__dsa/.432__dsa/.432__dsa/.432__dsa/.432__dsa/.432__dsa/.432__dsa/.432__dsa/.432__dsa/.432__dsa/.432__dsa/.432__dsa/.432__dsa/.432__dsa/.432__dsa/.432__dsa/.432__dsa/.432__dsa/.432__dsa/.432__dsa/.432__dsa/.432__dsa/.432__dsa/.432__dsa/.432__dsa/.432__dsa/.432__dsa/.432__dsa/.432__dsa/.432__dsa/.432__dsa/.432__dsa/.432__dsa/.432__dsa/.432__dsa/.432__dsa/.432__dsa/.432__dsa/.432__dsa/.432__dsa/.432__dsa/.432__dsa/.432__dsa/.432__dsa/.432__dsa/.432__dsa/.432__dsa/.432__dsa/.432__dsa/.432__dsa/.432__dsa/.432__dsa/.432__dsa/.432__dsa/.432__dsa/.432__dsa/.432__dsa/.432__dsa/.432__dsa/.432__dsa/.432__dsa/.432__dsa/.432__dsa/.432__dsa/.432__dsa/.432__dsa/.432__dsa/.432__dsa/.432__dsa/.432__dsa/.432__dsa/.432__dsa/.432__dsa/.432__dsa/.432__dsa/.432__dsa/.432__dsa/.432__dsa/.432__dsa/.432__dsa/.432__dsa/.432__dsa/.432__dsa/.432__dsa/.432__dsa/.432__dsa/.432__dsa/.432__dsa/.432__dsa/.432__dsa/.432__dsa/.432__dsa/.432__dsa/.432__dsa/.432__dsa/.432__dsa/.432__dsa/.432__dsa/.432__dsa/.432__dsa/.432__dsa/.432__dsa/.432__dsa/.432__dsa/.432__dsa/.432__dsa/.432__dsa/.432__dsa/.432__dsa/.432__dsa/.432__dsa/.432__dsa/.432__dsa/.432__dsa/.432__dsa/.432__dsa/.432__dsa/.432__dsa/.432__dsa/.432__dsa/.432__dsa/.432__dsa/.432__dsa/.432__dsa/.432__dsa/.432__dsa/.432__dsa/.432__dsa/.432__dsa/.432__dsa/.432__dsa/.432__dsa/.432__dsa/.432__dsa/.432__dsa/.432__dsa/.432__dsa/.432__dsa/.432__dsa/.432__dsa/.432__dsa/.432__dsa/.432__dsa/.432__dsa/.432__dsa/.432__dsa/.432__dsa/.432__dsa/.432__dsa/.432__dsa/.432__dsa/.432__dsa/.432__dsa/.432__dsa/.432__dsa/.432__dsa/.432__dsa/.432__dsa/.432__dsa/.432__dsa/.432__dsa/.432__dsa/.432__dsa/.432__dsa/.432__dsa/.432__dsa/.432__dsa/.432__dsa/.432__dsa/.432__dsa/.432__dsa/.432__dsa/.432__dsa/.432__dsa/.432__dsa/.432__dsa/.432__dsa/.432__dsa/.432__dsa/.432__dsa/.432__dsa/.432__dsa/.432__dsa/.432__dsa/.432__dsa/.432__dsa/.432__dsa/.432__dsa/.432__dsa/.432__dsa/.432__dsa/.432__dsa/.432__dsa/.432__dsa/.432__dsa/.432__dsa/.432__dsa/.432__dsa/.432__dsa/.432__dsa/.432__dsa/.432__dsa/.432__dsa/.432__dsa/.432__dsa/.432__dsa/.432__dsa/.432__dsa/.432__dsa/.432__dsa/.432__dsa/.432__dsa/.432__dsa/.432__dsa/.432__dsa/.432__dsa/.432__dsa/.432__dsa/.432__dsa/.432__dsa/.432__dsa/.432__dsa/.432__dsa/.432__dsa/.432__dsa/.432__dsa/.432__dsa/.432__dsa/.432__dsa/.432__dsa/.432__dsa/.432__dsa/.432__dsa/.432__dsa/.432__dsa/.432__dsa/.432__dsa/.432__dsa/.432__dsa/.432__dsa/.432__dsa/.432__dsa/.432__dsa/.432__dsa/.432__dsa/.432__dsa/.432__dsa/.432__dsa/.432__dsa/.432__dsa/.432__dsa/.432__dsa/.432__dsa/.432__dsa/.432__dsa/.432__dsa/.432__dsa/.432__dsa/.432__dsa/.432__dsa/.432__dsa/.432__dsa/.432__dsa/.432__dsa/.432__dsa/.432__dsa/.432__dsa/.432__dsa/.432__dsa/.432__dsa/.432__dsa/.432__dsa/.432__dsa/.432__dsa/.432__dsa/.432__dsa/.432__dsa/.432__dsa/.432__dsa/.432__dsa/.432__dsa/.432__dsa/.432__dsa/.432__dsa/.432__dsa/.432__dsa/.432__dsa/.432__dsa/.432__dsa/.432__dsa/.432__dsa/.432__dsa/.432__dsa/.432__dsa/.432__dsa/.432__dsa/.432__dsa/.432__dsa/.432__dsa/.432__dsa/.432__dsa/.432__dsa/.432__dsa/.432__dsa/.432__dsa/.432__dsa/.432__dsa/.432__dsa/.432__dsa/.432__dsa/.432__dsa/.432__dsa/.432__dsa/.432__dsa/.432__dsa/.432__dsa/.432__dsa/.432__dsa/.432__dsa/.432__dsa/.432__dsa/.432__dsa/.432__dsa/.432__dsa/.432__dsa/.432__dsa/.432__dsa/.432__dsa/.432__dsa/.432__dsa/.432__dsa/.432__dsa/.432__dsa/.432__dsa/.432__dsa/.432__dsa/.432__dsa/.432__dsa/.432__dsa/.432__dsa/.432__dsa/.432__dsa/.432__dsa/.432__dsa/.432__dsa/.432__dsa/.432__dsa/.432__dsa/.432__dsa/.432__dsa/.432__dsa/.432__dsa/.432__dsa/.432__dsa/.432__dsa/.432__dsa/.432__dsa/.432__dsa/.432__dsa/.432__dsa/.432__dsa/.432__dsa/.432__dsa/.432__dsa/.432__dsa/.432__dsa/.432__dsa/.432__dsa/.432__dsa/.432__dsa/.432__dsa/.432__dsa/.432__dsa/.432__dsa/.432__dsa/.432__dsa/.432__dsa/.432__dsa/.432__dsa/.432__dsa/.432__dsa/.432__dsa/.432__dsa/.432__dsa/.432__dsa/.432__dsa/.432__dsa/.432__dsa/.432__dsa/.432__dsa/.432__dsa/.432__dsa/.432__dsa/.432__dsa/.432__dsa/.432__dsa/.432__dsa/.432__dsa/.432__dsa/.432__dsa/.432__dsa/.432__dsa/.432__dsa/.432__dsa/.432__dsa/.432__dsa/.432__dsa/.432__dsa/.432__dsa/.432__dsa/.432__dsa/.432__dsa/.432__dsa/.432__dsa/.432__dsa/.432__dsa/.432__dsa/.432__dsa/.432__dsa/.432__dsa/.432__dsa/.432__dsa/.432__dsa/.432__dsa/.432__dsa/.432__dsa/.432", "$#$#$#$#$#$#$#$#$#$#$#$#$#$#$#$#$#$#$#$#$#$#$#$#$#$#$#$#$#$#$#$#$#$#$#$#$#$#$#$#$#$#$#$#$#$#$#$#$#$#$#$#$#$#$#$#$#$#$#$#$#$#$#$#$#$#$#$#$#$#$#$#$#$#$#$#$#$#$#$#$#$#$#$#$#$#$#$#$#$#$#$#$#$#$#$#$#$#$#$#$#$#$#$#$#$#$#$#$#$#$#$#$#$#$#$#$#$#$#$#$#$#$#$#$#$#$#$#$#$#$#$#$#$#$#$#$#$#$#$#$#$#$#$#$#$#$#$#$#$#$#$#$#$#$#$#$#$#$#$#$#$#$#$#$#$#$#$#$#$#$#$#$#$#$#$#$#$#$#$#$#$#$#$#$#$#$#$#$#$#$#$#$#$#$#$#$#$#$#$#$#$#$#$#$#$#$#$#$#$#$#$#$#$#$#$#$#$#$#$#$#$#$#$#$#$#$#$#$#$#$#$#$#$#$#$#$#$#$#$#$#$#$#$#$#$#$#$#$#$#$#$#$#$#$#$#$#$#$#$#$#$#$#$#$#$#$#$#$#$#$#$#$#$#$#$#$#$#$#$#$#$#$#$#$#$#$#$#$#$#$#$#$#$#$#$#$#$#$#$#$#$#$#$#$#$#$#$#$#$#$#$#$#$#$#$#$#$#$#$#$#$#$#$#$#$#$#$#$#$#$#$#$#$#$#$#$#$#$#$#$#$#$#$#$#$#$#$#$#$#$#$#$#$#$#$#$#$#$#$#$#$#$#$#$#$#$#$#$#$#$#$#$#$#$#$#$#$#$#$#$#$#$#$#$#$#$#$#$#$#$#$#$#$#$#$#$#$#$#$#$#$#$#$#$#$#$#$#$#$#$#$#$#$#$#$#$#$#$#$#$#$#$#$#$#$#$#$#$#$#$#$#$#$#$#$#$#$#$#$#$#$#$#$#$#$#$#$#$#$#$#$#$#$#$#$#$#$#$#$#$#$#$#$#$#$#$#$#$#$#$#$#$#$#$#$#$#$#$#$#$#$#$#$#$#$#$#$#$#$#$#$#$#$#$#$#$#$#$#$#$#$#$#$#$#$#$#$#$#$#$#$#$#$#$#$#$#$#$#$#$#$#$#$#$#$#$#$#$#$#$#$#$#$#$#$#$#$#$#$#$#$#$#$#$#$#$#$#$#$#$#$#$#$#$#$#$#$#$#$#$#$#$#$#$#$#$#$#$#$#$#$#$#$#$#$#$#$#$#$#$#$#$#$#$#$#$#$#$#$#$#$#$#$#$#$#$#$#$#$#$#$#$#$#$#$#$#$#$#$#$#$#$#$#$#$#$#$#$#$#$#$#$#$#$#$#$#$#$#$#$#$#$#$#$#$#$#$#$#$#$#$#$#$#$#$#$#$#$#$#$#$#$#$#$#$#$#$#$#$#$#$#$#$#$#$#$#$#$#$#$#$#$#$#$#$#$#$#$#$#$#$#$#$#$#$#$#$#$#$#$#$#$#$#$#$#$#$#$#$#$#$#$#$#$#$#$#$#$#$#$#$#$#$#$#$#$#$#$#$#$#$#$#$#$#$#$#$#$#$#$#$#$#$#$#$#$#$#$#$#$#$#$#$#$#$#$#$#$#$#$#$#$#$#$#$#$#$#$#$#$#$#$#$#$#$#$#$#$#$#$#$#$#$#$#$#$#$#$#$#$#$#$#$#$#$#$#$#$#$#$#$#$#$#$#$#$#$#$#$#$#$#$#$#$#$#$#$#$#$#$#$#$#$#$#$#$#$#$#$#$#$#$#$#$#$#$#$#$#$#$#$#$#$#$#$#$#$#$#$#$#$#$#$#$#$#$#$#$#$#$#$#$#$#$#$#$#$#$#$#$#$#$#$#$#$#$#$#$#$#$#$#$#$#$#$#$#$#$#$#$#$#$#$#$#$#$#$#$#$#$#$#$#$#$#$#$#$#$#$#$#$#$#$#$#$#$#$#$#$#$#$#$#$#$#$#$#$#$#$#$#$#$#$#$#$#$#$#$#$#$#$#$#$#$#$#$#$#$#$#$#$#$#$#$#$#$#$#$#$#$#$#$#$#$#$#$#$#$#$#$#$#$#$#$#$#$#$#$#$#$#$#$#$#$#$#$#$#$#$#$#$#$#$#$#$#$#$#$#$#$#$#$#$#$#$#$#$#$#$#$#$#$#$#$#$#$#$#$#$#$#$#$#$#$#$#$#$#$#$#$#$#$#$#$#$#$#$#$#$#$#$#$#$#$#$#$#$#$#$#$#$#$#$#$#$#$#$#$#$#$#$#$#$#$#$#$#$#$#$#$#$#$#$#$#$#$#$#$#$#$#$#$#$#$#$#$#$#$#$#$#$#$#$#$#$#$#$#$#$#$#$#$#$#$#$#$#$#$#$#$#$#$#$#$#$#$#$#$#$#$#$#$#$#$#$#$#$#$#$#$#$#$#$#$#$#$#$#$#$#$#$#$#$#$#$#$#$#$#$#$#$#$#$#$#$#$#$#$#$#$#$#$#$#$#$#$#$#$#$#$#$#$#$#$#$#$#$#$#$#$#$#$#$#$#$#$#$#$#$#$#$#$#$#$#$#$#$#$#$#$#$#$#$#$#$#$#$#$#$#$#$#$#$#$#$#$#$#$#$#$#$#$#$#$#$#$#$#$#$#$#$#$#$#$#$#$#$#$#$#$#$#$#$#$#$#$#$#$#$#$#$#$#$#$#$#$#$#$#$#$#$#$#$#$#$#$#$#$#$#$#$#$#$#$#$#$#$#$#$#$#$#$#$#$#$#$#$#$#$#$#$#$#$#$#$#$#$#$#$#$#$#$#$#$#$#$#$#$#$#$#$#$#$#$#$#$#$#$#$#$#$#$#$#$#$#$#$#$#$#$#$#$#$#$#$#$#$#$#$#$#$#$#$#$#$#$#$#$#$#$#$#$#$#$#$#$#$#$#$#$#$#$#$#$#$#$#$#$#$#$#$#$#$#$#$#$#$#$#$#$#$#$#$#$#$#$#$#$#$#$#$#$#$#$#$#$#$#$#$#$#$#$#$#$#$#$#$#$#$#$#$#$#$#$#$#$#$#$#$#$#$#$#$#$#$#$#$#$#$#$#$#$#$#$#$#$#$#$#$#$#$#$#$#$#$#$#$#$#$#$#$#$#$#$#$#$#$#$#$#$#$#$#$#$#$#$#$#$#$#$#$#$#$#$#$#$#$#$#$#$#$#$#$#$#$#$#$#$#$#$#$#$#$#$#$#$#$#$#$#$#$#$#$#$#$#$#$#$#$#$#$#$#$#$#$#$#$#$#$#$#$#$#$#$#$#$#$#$#$#$#$#$#$#$#$#$#$#$#$#$#$#$#$#$#$#$#$#$#$#$#$#$#$#$#$#$#$#$#$#$#$#$#$#$#$#$#$#$#$#$#$#$#$#$#$#$#$#$#$#$#$#$#$#$#$#$#$#$#$#$#$#$#$#$#$#$#$#$#$#$#$#$#$#$#$#$#$#$#$#$#$#$#$#$#$#$#$#$#$#$#$#$#$#$#$#$#$#$#$#$#$#$#$#$#$#$#$#$#$#$#$#$#$#$#$#$#$#$#$#$#$#$#$#$#$#$#$#$#$#$#$#$#$#$#$#$#$#$#$#$#$#$#$#$#$#$#$#$#$#$#$#$#$#$#$#$#$#$#$#$#$#$#$#$#$#$#$#$#$#$#$#$#$#$#$#$#$#$#$#$#$#$#$#$#$#$#$#$#$#$#$#$#$#$#$#$#$#$#$#$#$#$#$#$#$#$#$#$#$#$#$#$#$#$#$#$#$#$#$#$#$#$#$#$#$#$#$#$#$#$#$#$#$#$#$#$#$#$#$#$#$#$#$#$#$#$#$#$#$#$#$#$#$#$#$#$#$#$#$#$#$#$#$#$#$#$#$#$#$#$#$#$#$#$#$#$#$#$#$#$#$#$#$#$#$#$#$#$#$#$#$#$#$#$#$#$#$#$#$#$#$#$#$#$#$#$#$#$#$#$#$#$#$#$#$#$#$#$#$#$#$#$#$#$#$#$#$#$#$#$#$#$#$#$#$#$#$#$#$#$#$#$#$#$#$#$#$#$#$#$#$#$#$#$#$#$#$#$#$#$#$#$#$#$#$#$#$#$#$#$#$#$#$#$#$#$#$#$#$#$#$#$#$#$#$#$#$#$#$#$#$#$#$#$#$#$#$#$#$#$#$#$#$#$#$#$#$#$#$#$#$#$#$#$#$#$#$#$#$#$#$#$#$#$#$#$#$#$#$#$#$#$#$#$#$#$#$#$#$#$#$#$#$#$#$#$#$#$#$#$#$#$#$#$#$#$#$#$#$#$#$#$#$#$#$#$#$#$#$#$#$#$#$#$#$#$#$#$#$#", "pjlt';\\]`pjlt';\\]`pjlt';\\]`pjlt';\\]`pjlt';\\]`pjlt';\\]`pjlt';\\]`pjlt';\\]`pjlt';\\]`pjlt';\\]`pjlt';\\]`pjlt';\\]`pjlt';\\]`pjlt';\\]`pjlt';\\]`pjlt';\\]`pjlt';\\]`pjlt';\\]`pjlt';\\]`pjlt';\\]`pjlt';\\]`pjlt';\\]`pjlt';\\]`pjlt';\\]`pjlt';\\]`pjlt';\\]`pjlt';\\]`pjlt';\\]`pjlt';\\]`pjlt';\\]`pjlt';\\]`pjlt';\\]`pjlt';\\]`pjlt';\\]`pjlt';\\]`pjlt';\\]`pjlt';\\]`pjlt';\\]`pjlt';\\]`pjlt';\\]`pjlt';\\]`pjlt';\\]`pjlt';\\]`pjlt';\\]`pjlt';\\]`pjlt';\\]`pjlt';\\]`pjlt';\\]`pjlt';\\]`pjlt';\\]`pjlt';\\]`pjlt';\\]`pjlt';\\]`pjlt';\\]`pjlt';\\]`pjlt';\\]`pjlt';\\]`pjlt';\\]`pjlt';\\]`pjlt';\\]`pjlt';\\]`pjlt';\\]`pjlt';\\]`pjlt';\\]`pjlt';\\]`pjlt';\\]`pjlt';\\]`pjlt';\\]`pjlt';\\]`pjlt';\\]`pjlt';\\]`pjlt';\\]`pjlt';\\]`pjlt';\\]`pjlt';\\]`pjlt';\\]`pjlt';\\]`pjlt';\\]`pjlt';\\]`pjlt';\\]`pjlt';\\]`pjlt';\\]`pjlt';\\]`pjlt';\\]`pjlt';\\]`pjlt';\\]`pjlt';\\]`pjlt';\\]`pjlt';\\]`pjlt';\\]`pjlt';\\]`pjlt';\\]`pjlt';\\]`pjlt';\\]`pjlt';\\]`pjlt';\\]`pjlt';\\]`pjlt';\\]`pjlt';\\]`pjlt';\\]`pjlt';\\]`pjlt';\\]`pjlt';\\]`pjlt';\\]`pjlt';\\]`pjlt';\\]`pjlt';\\]`pjlt';\\]`pjlt';\\]`pjlt';\\]`pjlt';\\]`pjlt';\\]`pjlt';\\]`pjlt';\\]`pjlt';\\]`pjlt';\\]`pjlt';\\]`pjlt';\\]`pjlt';\\]`pjlt';\\]`pjlt';\\]`pjlt';\\]`pjlt';\\]`pjlt';\\]`pjlt';\\]`pjlt';\\]`pjlt';\\]`pjlt';\\]`pjlt';\\]`pjlt';\\]`pjlt';\\]`pjlt';\\]`pjlt';\\]`pjlt';\\]`pjlt';\\]`pjlt';\\]`pjlt';\\]`pjlt';\\]`pjlt';\\]`pjlt';\\]`pjlt';\\]`pjlt';\\]`pjlt';\\]`pjlt';\\]`pjlt';\\]`pjlt';\\]`pjlt';\\]`pjlt';\\]`pjlt';\\]`pjlt';\\]`pjlt';\\]`pjlt';\\]`pjlt';\\]`pjlt';\\]`pjlt';\\]`pjlt';\\]`pjlt';\\]`pjlt';\\]`pjlt';\\]`pjlt';\\]`pjlt';\\]`pjlt';\\]`pjlt';\\]`pjlt';\\]`pjlt';\\]`pjlt';\\]`pjlt';\\]`pjlt';\\]`pjlt';\\]`pjlt';\\]`pjlt';\\]`pjlt';\\]`pjlt';\\]`pjlt';\\]`pjlt';\\]`pjlt';\\]`pjlt';\\]`pjlt';\\]`pjlt';\\]`pjlt';\\]`pjlt';\\]`pjlt';\\]`pjlt';\\]`pjlt';\\]`pjlt';\\]`pjlt';\\]`pjlt';\\]`pjlt';\\]`pjlt';\\]`pjlt';\\]`pjlt';\\]`pjlt';\\]`pjlt';\\]`pjlt';\\]`pjlt';\\]`pjlt';\\]`pjlt';\\]`pjlt';\\]`pjlt';\\]`pjlt';\\]`pjlt';\\]`pjlt';\\]`pjlt';\\]`pjlt';\\]`pjlt';\\]`pjlt';\\]`pjlt';\\]`pjlt';\\]`pjlt';\\]`pjlt';\\]`pjlt';\\]`pjlt';\\]`pjlt';\\]`pjlt';\\]`pjlt';\\]`pjlt';\\]`pjlt';\\]`pjlt';\\]`pjlt';\\]`pjlt';\\]`pjlt';\\]`pjlt';\\]`pjlt';\\]`pjlt';\\]`pjlt';\\]`pjlt';\\]`pjlt';\\]`pjlt';\\]`pjlt';\\]`pjlt';\\]`pjlt';\\]`pjlt';\\]`pjlt';\\]`pjlt';\\]`pjlt';\\]`pjlt';\\]`pjlt';\\]`pjlt';\\]`pjlt';\\]`pjlt';\\]`pjlt';\\]`pjlt';\\]`pjlt';\\]`pjlt';\\]`pjlt';\\]`pjlt';\\]`pjlt';\\]`pjlt';\\]`pjlt';\\]`pjlt';\\]`pjlt';\\]`pjlt';\\]`pjlt';\\]`pjlt';\\]`pjlt';\\]`pjlt';\\]`pjlt';\\]`pjlt';\\]`pjlt';\\]`pjlt';\\]`pjlt';\\]`pjlt';\\]`pjlt';\\]`pjlt';\\]`pjlt';\\]`pjlt';\\]`pjlt';\\]`pjlt';\\]`pjlt';\\]`pjlt';\\]`pjlt';\\]`pjlt';\\]`pjlt';\\]`pjlt';\\]`pjlt';\\]`pjlt';\\]`pjlt';\\]`pjlt';\\]`pjlt';\\]`pjlt';\\]`pjlt';\\]`pjlt';\\]`pjlt';\\]`pjlt';\\]`pjlt';\\]`pjlt';\\]`pjlt';\\]`pjlt';\\]`pjlt';\\]`pjlt';\\]`pjlt';\\]`pjlt';\\]`pjlt';\\]`pjlt';\\]`pjlt';\\]`pjlt';\\]`pjlt';\\]`pjlt';\\]`pjlt';\\]`pjlt';\\]`pjlt';\\]`pjlt';\\]`pjlt';\\]`pjlt';\\]`pjlt';\\]`pjlt';\\]`pjlt';\\]`pjlt';\\]`pjlt';\\]`pjlt';\\]`pjlt';\\]`pjlt';\\]`pjlt';\\]`pjlt';\\]`pjlt';\\]`pjlt';\\]`pjlt';\\]`pjlt';\\]`pjlt';\\]`pjlt';\\]`pjlt';\\]`pjlt';\\]`pjlt';\\]`pjlt';\\]`pjlt';\\]`pjlt';\\]`pjlt';\\]`pjlt';\\]`pjlt';\\]`pjlt';\\]`pjlt';\\]`pjlt';\\]`pjlt';\\]`pjlt';\\]`pjlt';\\]`pjlt';\\]`pjlt';\\]`pjlt';\\]`pjlt';\\]`pjlt';\\]`pjlt';\\]`pjlt';\\]`pjlt';\\]`pjlt';\\]`pjlt';\\]`pjlt';\\]`pjlt';\\]`pjlt';\\]`pjlt';\\]`pjlt';\\]`pjlt';\\]`pjlt';\\]`pjlt';\\]`pjlt';\\]`pjlt';\\]`pjlt';\\]`pjlt';\\]`pjlt';\\]`pjlt';\\]`pjlt';\\]`pjlt';\\]`pjlt';\\]`pjlt';\\]`pjlt';\\]`pjlt';\\]`pjlt';\\]`pjlt';\\]`pjlt';\\]`pjlt';\\]`pjlt';\\]`pjlt';\\]`pjlt';\\]`pjlt';\\]`pjlt';\\]`pjlt';\\]`pjlt';\\]`pjlt';\\]`pjlt';\\]`pjlt';\\]`pjlt';\\]`pjlt';\\]`pjlt';\\]`pjlt';\\]`pjlt';\\]`pjlt';\\]`pjlt';\\]`pjlt';\\]`pjlt';\\]`pjlt';\\]`pjlt';\\]`pjlt';\\]`pjlt';\\]`pjlt';\\]`pjlt';\\]`pjlt';\\]`pjlt';\\]`pjlt';\\]`pjlt';\\]`pjlt';\\]`pjlt';\\]`pjlt';\\]`pjlt';\\]`pjlt';\\]`pjlt';\\]`pjlt';\\]`pjlt';\\]`pjlt';\\]`pjlt';\\]`pjlt';\\]`pjlt';\\]`pjlt';\\]`pjlt';\\]`pjlt';\\]`pjlt';\\]`pjlt';\\]`pjlt';\\]`pjlt';\\]`pjlt';\\]`pjlt';\\]`pjlt';\\]`pjlt';\\]`pjlt';\\]`pjlt';\\]`pjlt';\\]`pjlt';\\]`pjlt';\\]`pjlt';\\]`pjlt';\\]`pjlt';\\]`pjlt';\\]`pjlt';\\]`pjlt';\\]`pjlt';\\]`pjlt';\\]`pjlt';\\]`pjlt';\\]`pjlt';\\]`pjlt';\\]`pjlt';\\]`pjlt';\\]`pjlt';\\]`pjlt';\\]`pjlt';\\]`pjlt';\\]`pjlt';\\]`pjlt';\\]`pjlt';\\]`pjlt';\\]`pjlt';\\]`pjlt';\\]`pjlt';\\]`pjlt';\\]`pjlt';\\]`pjlt';\\]`pjlt';\\]`pjlt';\\]`pjlt';\\]`pjlt';\\]`pjlt';\\]`pjlt';\\]`pjlt';\\]`pjlt';\\]`pjlt';\\]`pjlt';\\]`pjlt';\\]`pjlt';\\]`pjlt';\\]`pjlt';\\]`pjlt';\\]`pjlt';\\]`pjlt';\\]`pjlt';\\]`pjlt';\\]`pjlt';\\]`pjlt';\\]`pjlt';\\]`pjlt';\\]`pjlt';\\]`pjlt';\\]`pjlt';\\]`pjlt';\\]`pjlt';\\]`pjlt';\\]`pjlt';\\]`pjlt';\\]`pjlt';\\]`pjlt';\\]`pjlt';\\]`pjlt';\\]`pjlt';\\]`pjlt';\\]`pjlt';\\]`pjlt';\\]`pjlt';\\]`pjlt';\\]`pjlt';\\]`pjlt';\\]`pjlt';\\]`pjlt';\\]`pjlt';\\]`pjlt';\\]`pjlt';\\]`pjlt';\\]`pjlt';\\]`pjlt';\\]`pjlt';\\]`pjlt';\\]`pjlt';\\]`pjlt';\\]`pjlt';\\]`pjlt';\\]`pjlt';\\]`pjlt';\\]`pjlt';\\]`pjlt';\\]`pjlt';\\]`pjlt';\\]`pjlt';\\]`pjlt';\\]`pjlt';\\]`pjlt';\\]`pjlt';\\]`pjlt';\\]`pjlt';\\]`pjlt';\\]`pjlt';\\]`pjlt';\\]`pjlt';\\]`pjlt';\\]`pjlt';\\]`pjlt';\\]`pjlt';\\]`pjlt';\\]`pjlt';\\]`pjlt';\\]`pjlt';\\]`pjlt';\\]`pjlt';\\]`pjlt';\\]`pjlt';\\]`pjlt';\\]`pjlt';\\]`pjlt';\\]`pjlt';\\]`pjlt';\\]`pjlt';\\]`pjlt';\\]`pjlt';\\]`pjlt';\\]`pjlt';\\]`pjlt';\\]`pjlt';\\]`pjlt';\\]`pjlt';\\]`pjlt';\\]`pjlt';\\]`pjlt';\\]`pjlt';\\]`pjlt';\\]`pjlt';\\]`pjlt';\\]`pjlt';\\]`pjlt';\\]`pjlt';\\]`pjlt';\\]`pjlt';\\]`pjlt';\\]`pjlt';\\]`pjlt';\\]`pjlt';\\]`pjlt';\\]`pjlt';\\]`pjlt';\\]`pjlt';\\]`pjlt';\\]`pjlt';\\]`pjlt';\\]`pjlt';\\]`pjlt';\\]`pjlt';\\]`pjlt';\\]`pjlt';\\]`pjlt';\\]`pjlt';\\]`pjlt';\\]`pjlt';\\]`pjlt';\\]`pjlt';\\]`pjlt';\\]`pjlt';\\]`pjlt';\\]`pjlt';\\]`pjlt';\\]`pjlt';\\]`pjlt';\\]`pjlt';\\]`pjlt';\\]`pjlt';\\]`pjlt';\\]`pjlt';\\]`pjlt';\\]`pjlt';\\]`pjlt';\\]`pjlt';\\]`pjlt';\\]`pjlt';\\]`pjlt';\\]`pjlt';\\]`pjlt';\\]`pjlt';\\]`pjlt';\\]`pjlt';\\]`pjlt';\\]`pjlt';\\]`pjlt';\\]`pjlt';\\]`pjlt';\\]`pjlt';\\]`pjlt';\\]`pjlt';\\]`pjlt';\\]`pjlt';\\]`pjlt';\\]`pjlt';\\]`pjlt';\\]`pjlt';\\]`pjlt';\\]`pjlt';\\]`pjlt';\\]`pjlt';\\]`pjlt';\\]`pjlt';\\]`pjlt';\\]`pjlt';\\]`pjlt';\\]`pjlt';\\]`pjlt';\\]`pjlt';\\]`pjlt';\\]`pjlt';\\]`pjlt';\\]`pjlt';\\]`pjlt';\\]`pjlt';\\]`pjlt';\\]`pjlt';\\]`pjlt';\\]`pjlt';\\]`pjlt';\\]`pjlt';\\]`pjlt';\\]`pjlt';\\]`pjlt';\\]`pjlt';\\]`pjlt';\\]`pjlt';\\]`pjlt';\\]`pjlt';\\]`pjlt';\\]`pjlt';\\]`pjlt';\\]`pjlt';\\]`pjlt';\\]`pjlt';\\]`pjlt';\\]`pjlt';\\]`pjlt';\\]`pjlt';\\]`pjlt';\\]`pjlt';\\]`pjlt';\\]`pjlt';\\]`pjlt';\\]`pjlt';\\]`pjlt';\\]`pjlt';\\]`pjlt';\\]`pjlt';\\]`pjlt';\\]`pjlt';\\]`pjlt';\\]`pjlt';\\]`pjlt';\\]`pjlt';\\]`pjlt';\\]`pjlt';\\]`pjlt';\\]`pjlt';\\]`pjlt';\\]`pjlt';\\]`pjlt';\\]`pjlt';\\]`pjlt';\\]`pjlt';\\]`pjlt';\\]`pjlt';\\]`pjlt';\\]`pjlt';\\]`pjlt';\\]`pjlt';\\]`pjlt';\\]`pjlt';\\]`pjlt';\\]`pjlt';\\]`pjlt';\\]`pjlt';\\]`pjlt';\\]`pjlt';\\]`pjlt';\\]`pjlt';\\]`pjlt';\\]`pjlt';\\]`pjlt';\\]`pjlt';\\]`pjlt';\\]`pjlt';\\]`pjlt';\\]`pjlt';\\]`pjlt';\\]`pjlt';\\]`pjlt';\\]`pjlt';\\]`pjlt';\\]`pjlt';\\]`pjlt';\\]`pjlt';\\]`pjlt';\\]`pjlt';\\]`pjlt';\\]`pjlt';\\]`pjlt';\\]`pjlt';\\]`pjlt';\\]`pjlt';\\]`pjlt';\\]`pjlt';\\]`pjlt';\\]`pjlt';\\]`pjlt';\\]`pjlt';\\]`pjlt';\\]`pjlt';\\]`pjlt';\\]`pjlt';\\]`pjlt';\\]`pjlt';\\]`pjlt';\\]`pjlt';\\]`pjlt';\\]`pjlt';\\]`pjlt';\\]`pjlt';\\]`pjlt';\\]`pjlt';\\]`pjlt';\\]`pjlt';\\]`pjlt';\\]`pjlt';\\]`pjlt';\\]`pjlt';\\]`pjlt';\\]`pjlt';\\]`pjlt';\\]`pjlt';\\]`pjlt';\\]`pjlt';\\]`pjlt';\\]`pjlt';\\]`pjlt';\\]`pjlt';\\]`pjlt';\\]`pjlt';\\]`pjlt';\\]`pjlt';\\]`pjlt';\\]`pjlt';\\]`pjlt';\\]`pjlt';\\]`pjlt';\\]`pjlt';\\]`pjlt';\\]`pjlt';\\]`pjlt';\\]`pjlt';\\]`pjlt';\\]`pjlt';\\]`pjlt';\\]`pjlt';\\]`pjlt';\\]`pjlt';\\]`pjlt';\\]`pjlt';\\]`pjlt';\\]`pjlt';\\]`pjlt';\\]`pjlt';\\]`pjlt';\\]`pjlt';\\]`pjlt';\\]`pjlt';\\]`pjlt';\\]`pjlt';\\]`pjlt';\\]`pjlt';\\]`pjlt';\\]`pjlt';\\]`pjlt';\\]`pjlt';\\]`pjlt';\\]`pjlt';\\]`pjlt';\\]`pjlt';\\]`pjlt';\\]`pjlt';\\]`pjlt';\\]`pjlt';\\]`pjlt';\\]`pjlt';\\]`pjlt';\\]`pjlt';\\]`pjlt';\\]`pjlt';\\]`pjlt';\\]`pjlt';\\]`pjlt';\\]`pjlt';\\]`pjlt';\\]`pjlt';\\]`pjlt';\\]`pjlt';\\]`pjlt';\\]`pjlt';\\]`pjlt';\\]`pjlt';\\]`pjlt';\\]`pjlt';\\]`pjlt';\\]`pjlt';\\]`pjlt';\\]`pjlt';\\]`pjlt';\\]`pjlt';\\]`pjlt';\\]`pjlt';\\]`pjlt';\\]`pjlt';\\]`pjlt';\\]`pjlt';\\]`pjlt';\\]`pjlt';\\]`pjlt';\\]`pjlt';\\]`pjlt';\\]`pjlt';\\]`pjlt';\\]`pjlt';\\]`pjlt';\\]`pjlt';\\]`pjlt';\\]`pjlt';\\]`pjlt';\\]`pjlt';\\]`pjlt';\\]`pjlt';\\]`pjlt';\\]`pjlt';\\]`pjlt';\\]`pjlt';\\]`pjlt';\\]`pjlt';\\]`pjlt';\\]`pjlt';\\]`pjlt';\\]`pjlt';\\]`pjlt';\\]`pjlt';\\]`pjlt';\\]`pjlt';\\]`pjlt';\\]`pjlt';\\]`pjlt';\\]`pjlt';\\]`pjlt';\\]`pjlt';\\]`pjlt';\\]`pjlt';\\]`pjlt';\\]`pjlt';\\]`pjlt';\\]`pjlt';\\]`pjlt';\\]`pjlt';\\]`pjlt';\\]`pjlt';\\]`pjlt';\\]`pjlt';\\]`pjlt';\\]`pjlt';\\]`pjlt';\\]`pjlt';\\]`pjlt';\\]`pjlt';\\]`pjlt';\\]`pjlt';\\]`pjlt';\\]`pjlt';\\]`pjlt';\\]`pjlt';\\]`pjlt';\\]`pjlt';\\]`pjlt';\\]`pjlt';\\]`pjlt';\\]`pjlt';\\]`pjlt';\\]`pjlt';\\]`pjlt';\\]`pjlt';\\]`pjlt';\\]`pjlt';\\]`pjlt';\\]`pjlt';\\]`pjlt';\\]`pjlt';\\]`pjlt';\\]`pjlt';\\]`pjlt';\\]`pjlt';\\]`pjlt';\\]`pjlt';\\]`pjlt';\\]`pjlt';\\]`pjlt';\\]`pjlt';\\]`pjlt';\\]`pjlt';\\]`pjlt';\\]`pjlt';\\]`pjlt';\\]`pjlt';\\]`pjlt';\\]`pjlt';\\]`pjlt';\\]`pjlt';\\]`pjlt';\\]`pjlt';\\]`pjlt';\\]`pjlt';\\]`pjlt';\\]`pjlt';\\]`pjlt';\\]`pjlt';\\]`pjlt';\\]`pjlt';\\]`pjlt';\\]`pjlt';\\]`pjlt';\\]`pjlt';\\]`pjlt';\\]`pjlt';\\]`pjlt';\\]`pjlt';\\]`pjlt';\\]`pjlt';\\]`pjlt';\\]`pjlt';\\]`pjlt';\\]`pjlt';\\]`pjlt';\\]`pjlt';\\]`pjlt';\\]`pjlt';\\]`pjlt';\\]`pjlt';\\]`pjlt';\\]`pjlt';\\]`pjlt';\\]`pjlt';\\]`pjlt';\\]`pjlt';\\]`pjlt';\\]`pjlt';\\]`pjlt';\\]`pjlt';\\]`pjlt';\\]`pjlt';\\]`pjlt';\\]`pjlt';\\]`pjlt';\\]`pjlt';\\]`pjlt';\\]`pjlt';\\]`pjlt';\\]`pjlt';\\]`pjlt';\\]`pjlt';\\]`pjlt';\\]`pjlt';\\]`pjlt';\\]`pjlt';\\]`pjlt';\\]`pjlt';\\]`pjlt';\\]`pjlt';\\]`pjlt';\\]`pjlt';\\]`pjlt';\\]`pjlt';\\]`pjlt';\\]`pjlt';\\]`pjlt';\\]`pjlt';\\]`pjlt';\\]`pjlt';\\]`pjlt';\\]`pjlt';\\]`pjlt';\\]`pjlt';\\]`pjlt';\\]`pjlt';\\]`pjlt';\\]`pjlt';\\]`pjlt';\\]`pjlt';\\]`pjlt';\\]`pjlt';\\]`pjlt';\\]`pjlt';\\]`pjlt';\\]`pjlt';\\]`pjlt';\\]`pjlt';\\]`pjlt';\\]`pjlt';\\]`pjlt';\\]`pjlt';\\]`pjlt';\\]`pjlt';\\]`pjlt';\\]`pjlt';\\]`pjlt';\\]`pjlt';\\]`pjlt';\\]`pjlt';\\]`pjlt';\\]`pjlt';\\]`pjlt';\\]`pjlt';\\]`pjlt';\\]`pjlt';\\]`pjlt';\\]`pjlt';\\]`pjlt';\\]`pjlt';\\]`pjlt';\\]`pjlt';\\]`pjlt';\\]`pjlt';\\]`pjlt';\\]`pjlt';\\]`pjlt';\\]`pjlt';\\]`pjlt';\\]`pjlt';\\]`pjlt';\\]`pjlt';\\]`pjlt';\\]`pjlt';\\]`pjlt';\\]`pjlt';\\]`pjlt';\\]`pjlt';\\]`pjlt';\\]`pjlt';\\]`pjlt';\\]`pjlt';\\]`pjlt';\\]`pjlt';\\]`pjlt';\\]`pjlt';\\]`pjlt';\\]`pjlt';\\]`pjlt';\\]`pjlt';\\]`pjlt';\\]`pjlt';\\]`pjlt';\\]`pjlt';\\]`pjlt';\\]`pjlt';\\]`pjlt';\\]`pjlt';\\]`pjlt';\\]`pjlt';\\]`pjlt';\\]`pjlt';\\]`pjlt';\\]`pjlt';\\]`pjlt';\\]`pjlt';\\]`pjlt';\\]`pjlt';\\]`pjlt';\\]`pjlt';\\]`pjlt';\\]`pjlt';\\]`pjlt';\\]`pjlt';\\]`pjlt';\\]`pjlt';\\]`pjlt';\\]`pjlt';\\]`pjlt';\\]`pjlt';\\]`pjlt';\\]`pjlt';\\]`pjlt';\\]`pjlt';\\]`pjlt';\\]`pjlt';\\]`pjlt';\\]`pjlt';\\]`pjlt';\\]`pjlt';\\]`pjlt';\\]`pjlt';\\]`pjlt';\\]`pjlt';\\]`pjlt';\\]`pjlt';\\]`pjlt';\\]`pjlt';\\]`pjlt';\\]`pjlt';\\]`pjlt';\\]`pjlt';\\]`pjlt';\\]`pjlt';\\]`pjlt';\\]`pjlt';\\]`pjlt';\\]`pjlt';\\]`pjlt';\\]`pjlt';\\]`pjlt';\\]`pjlt';\\]`pjlt';\\]`pjlt';\\]`pjlt';\\]`pjlt';\\]`pjlt';\\]`pjlt';\\]`pjlt';\\]`pjlt';\\]`pjlt';\\]`pjlt';\\]`pjlt';\\]`pjlt';\\]`pjlt';\\]`pjlt';\\]`pjlt';\\]`pjlt';\\]`pjlt';\\]`pjlt';\\]`pjlt';\\]`pjlt';\\]`pjlt';\\]`pjlt';\\]`pjlt';\\]`pjlt';\\]`pjlt';\\]`pjlt';\\]`pjlt';\\]`pjlt';\\]`pjlt';\\]`pjlt';\\]`pjlt';\\]`pjlt';\\]`pjlt';\\]`pjlt';\\]`pjlt';\\]`pjlt';\\]`pjlt';\\]`pjlt';\\]`pjlt';\\]`pjlt';\\]`pjlt';\\]`pjlt';\\]`pjlt';\\]`pjlt';\\]`pjlt';\\]`pjlt';\\]`pjlt';\\]`pjlt';\\]`pjlt';\\]`pjlt';\\]`pjlt';\\]`pjlt';\\]`pjlt';\\]`pjlt';\\]`pjlt';\\]`pjlt';\\]`pjlt';\\]`pjlt';\\]`pjlt';\\]`pjlt';\\]`pjlt';\\]`pjlt';\\]`pjlt';\\]`pjlt';\\]`pjlt';\\]`pjlt';\\]`pjlt';\\]`pjlt';\\]`pjlt';\\]`pjlt';\\]`pjlt';\\]`pjlt';\\]`pjlt';\\]`pjlt';\\]`pjlt';\\]`pjlt';\\]`pjlt';\\]`pjlt';\\]`pjlt';\\]`pjlt';\\]`pjlt';\\]`pjlt';\\]`pjlt';\\]`pjlt';\\]`pjlt';\\]`pjlt';\\]`pjlt';\\]`pjlt';\\]`pjlt';\\]`pjlt';\\]`pjlt';\\]`pjlt';\\]`pjlt';\\]`pjlt';\\]`pjlt';\\]`pjlt';\\]`pjlt';\\]`pjlt';\\]`pjlt';\\]`pjlt';\\]`pjlt';\\]`pjlt';\\]`pjlt';\\]`pjlt';\\]`pjlt';\\]`pjlt';\\]`pjlt';\\]`pjlt';\\]`pjlt';\\]`pjlt';\\]`pjlt';\\]`pjlt';\\]`pjlt';\\]`pjlt';\\]`pjlt';\\]`pjlt';\\]`pjlt';\\]`pjlt';\\]`pjlt';\\]`pjlt';\\]`pjlt';\\]`pjlt';\\]`pjlt';\\]`pjlt';\\]`pjlt';\\]`pjlt';\\]`pjlt';\\]`pjlt';\\]`pjlt';\\]`pjlt';\\]`pjlt';\\]`pjlt';\\]`pjlt';\\]`pjlt';\\]`pjlt';\\]`pjlt';\\]`pjlt';\\]`pjlt';\\]`pjlt';\\]`pjlt';\\]`pjlt';\\]`pjlt';\\]`pjlt';\\]`pjlt';\\]`pjlt';\\]`pjlt';\\]`pjlt';\\]`pjlt';\\]`pjlt';\\]`pjlt';\\]`pjlt';\\]`pjlt';\\]`pjlt';\\]`pjlt';\\]`pjlt';\\]`pjlt';\\]`pjlt';\\]`pjlt';\\]`pjlt';\\]`pjlt';\\]`pjlt';\\]`pjlt';\\]`pjlt';\\]`pjlt';\\]`pjlt';\\]`pjlt';\\]`pjlt';\\]`pjlt';\\]`pjlt';\\]`pjlt';\\]`pjlt';\\]`pjlt';\\]`pjlt';\\]`pjlt';\\]`pjlt';\\]`pjlt';\\]`pjlt';\\]`pjlt';\\]`pjlt';\\]`pjlt';\\]`pjlt';\\]`pjlt';\\]`pjlt';\\]`pjlt';\\]`pjlt';\\]`pjlt';\\]`pjlt';\\]`pjlt';\\]`pjlt';\\]`pjlt';\\]`pjlt';\\]`pjlt';\\]`pjlt';\\]`pjlt';\\]`pjlt';\\]`pjlt';\\]`pjlt';\\]`pjlt';\\]`pjlt';\\]`pjlt';\\]`pjlt';\\]`pjlt';\\]`pjlt';\\]`pjlt';\\]`pjlt';\\]`pjlt';\\]`pjlt';\\]`pjlt';\\]`pjlt';\\]`pjlt';\\]`pjlt';\\]`pjlt';\\]`pjlt';\\]`pjlt';\\]`pjlt';\\]`pjlt';\\]`pjlt';\\]`pjlt';\\]`pjlt';\\]`pjlt';\\]`pjlt';\\]`pjlt';\\]`pjlt';\\]`pjlt';\\]`pjlt';\\]`pjlt';\\]`pjlt';\\]`pjlt';\\]`pjlt';\\]`pjlt';\\]`pjlt';\\]`pjlt';\\]`pjlt';\\]`pjlt';\\]`pjlt';\\]`pjlt';\\]`pjlt';\\]`pjlt';\\]`pjlt';\\]`pjlt';\\]`pjlt';\\]`pjlt';\\]`pjlt';\\]`pjlt';\\]`pjlt';\\]`pjlt';\\]`pjlt';\\]`pjlt';\\]`pjlt';\\]`pjlt';\\]`pjlt';\\]`pjlt';\\]`pjlt';\\]`pjlt';\\]`pjlt';\\]`pjlt';\\]`pjlt';\\]`pjlt';\\]`pjlt';\\]`pjlt';\\]`pjlt';\\]`pjlt';\\]`pjlt';\\]`pjlt';\\]`pjlt';\\]`pjlt';\\]`pjlt';\\]`pjlt';\\]`pjlt';\\]`pjlt';\\]`pjlt';\\]`pjlt';\\]`pjlt';\\]`pjlt';\\]`pjlt';\\]`pjlt';\\]`pjlt';\\]`pjlt';\\]`pjlt';\\]`pjlt';\\]`pjlt';\\]`pjlt';\\]`pjlt';\\]`pjlt';\\]`pjlt';\\]`pjlt';\\]`pjlt';\\]`pjlt';\\]`pjlt';\\]`pjlt';\\]`pjlt';\\]`pjlt';\\]`pjlt';\\]`pjlt';\\]`pjlt';\\]`pjlt';\\]`pjlt';\\]`pjlt';\\]`pjlt';\\]`pjlt';\\]`pjlt';\\]`pjlt';\\]`pjlt';\\]`pjlt';\\]`pjlt';\\]`pjlt';\\]`pjlt';\\]`pjlt';\\]`pjlt';\\]`pjlt';\\]`pjlt';\\]`pjlt';\\]`pjlt';\\]`pjlt';\\]`pjlt';\\]`pjlt';\\]`pjlt';\\]`pjlt';\\]`pjlt';\\]`pjlt';\\]`pjlt';\\]`pjlt';\\]`pjlt';\\]`pjlt';\\]`pjlt';\\]`pjlt';\\]`pjlt';\\]`pjlt';\\]`pjlt';\\]`pjlt';\\]`pjlt';\\]`pjlt';\\]`pjlt';\\]`pjlt';\\]`pjlt';\\]`pjlt';\\]`pjlt';\\]`pjlt';\\]`pjlt';\\]`pjlt';\\]`pjlt';\\]`pjlt';\\]`pjlt';\\]`pjlt';\\]`pjlt';\\]`pjlt';\\]`pjlt';\\]`pjlt';\\]`pjlt';\\]`pjlt';\\]`pjlt';\\]`pjlt';\\]`pjlt';\\]`pjlt';\\]`pjlt';\\]`pjlt';\\]`pjlt';\\]`pjlt';\\]`pjlt';\\]`pjlt';\\]`pjlt';\\]`pjlt';\\]`pjlt';\\]`pjlt';\\]`pjlt';\\]`pjlt';\\]`pjlt';\\]`pjlt';\\]`pjlt';\\]`pjlt';\\]`pjlt';\\]`pjlt';\\]`pjlt';\\]`pjlt';\\]`pjlt';\\]`pjlt';\\]`pjlt';\\]`pjlt';\\]`pjlt';\\]`pjlt';\\]`pjlt';\\]`pjlt';\\]`pjlt';\\]`pjlt';\\]`pjlt';\\]`pjlt';\\]`pjlt';\\]`pjlt';\\]`pjlt';\\]`pjlt';\\]`pjlt';\\]`pjlt';\\]`pjlt';\\]`pjlt';\\]`pjlt';\\]`pjlt';\\]`pjlt';\\]`pjlt';\\]`pjlt';\\]`pjlt';\\]`pjlt';\\]`pjlt';\\]`pjlt';\\]`pjlt';\\]`pjlt';\\]`pjlt';\\]`pjlt';\\]`pjlt';\\]`pjlt';\\]`pjlt';\\]`pjlt';\\]`pjlt';\\]`pjlt';\\]`pjlt';\\]`pjlt';\\]`pjlt';\\]`pjlt';\\]`pjlt';\\]`pjlt';\\]`pjlt';\\]`pjlt';\\]`pjlt';\\]`pjlt';\\]`pjlt';\\]`pjlt';\\]`pjlt';\\]`pjlt';\\]`pjlt';\\]`pjlt';\\]`pjlt';\\]`pjlt';\\]`pjlt';\\]`pjlt';\\]`pjlt';\\]`pjlt';\\]`pjlt';\\]`pjlt';\\]`pjlt';\\]`pjlt';\\]`pjlt';\\]`pjlt';\\]`pjlt';\\]`pjlt';\\]`pjlt';\\]`pjlt';\\]`pjlt';\\]`pjlt';\\]`pjlt';\\]`pjlt';\\]`pjlt';\\]`pjlt';\\]`pjlt';\\]`pjlt';\\]`pjlt';\\]`pjlt';\\]`pjlt';\\]`pjlt';\\]`pjlt';\\]`pjlt';\\]`pjlt';\\]`pjlt';\\]`pjlt';\\]`pjlt';\\]`pjlt';\\]`pjlt';\\]`pjlt';\\]`pjlt';\\]`pjlt';\\]`pjlt';\\]`pjlt';\\]`pjlt';\\]`pjlt';\\]`pjlt';\\]`pjlt';\\]`pjlt';\\]`pjlt';\\]`pjlt';\\]`pjlt';\\]`pjlt';\\]`pjlt';\\]`pjlt';\\]`pjlt';\\]`pjlt';\\]`pjlt';\\]`pjlt';\\]`pjlt';\\]`pjlt';\\]`pjlt';\\]`pjlt';\\]`pjlt';\\]`pjlt';\\]`pjlt';\\]`pjlt';\\]`pjlt';\\]`pjlt';\\]`pjlt';\\]`pjlt';\\]`pjlt';\\]`pjlt';\\]`pjlt';\\]`pjlt';\\]`pjlt';\\]`pjlt';\\]`pjlt';\\]`pjlt';\\]`pjlt';\\]`pjlt';\\]`pjlt';\\]`pjlt';\\]`pjlt';\\]`pjlt';\\]`pjlt';\\]`pjlt';\\]`pjlt';\\]`pjlt';\\]`pjlt';\\]`pjlt';\\]`pjlt';\\]`pjlt';\\]`pjlt';\\]`pjlt';\\]`pjlt';\\]`pjlt';\\]`pjlt';\\]`pjlt';\\]`pjlt';\\]`pjlt';\\]`pjlt';\\]`pjlt';\\]`pjlt';\\]`pjlt';\\]`pjlt';\\]`pjlt';\\]`pjlt';\\]`pjlt';\\]`pjlt';\\]`pjlt';\\]`pjlt';\\]`pjlt';\\]`pjlt';\\]`pjlt';\\]`pjlt';\\]`pjlt';\\]`pjlt';\\]`pjlt';\\]`pjlt';\\]`pjlt';\\]`pjlt';\\]`pjlt';\\]`pjlt';\\]`pjlt';\\]`pjlt';\\]`pjlt';\\]`pjlt';\\]`pjlt';\\]`pjlt';\\]`pjlt';\\]`pjlt';\\]`pjlt';\\]`pjlt';\\]`pjlt';\\]`pjlt';\\]`pjlt';\\]`pjlt';\\]`pjlt';\\]`pjlt';\\]`pjlt';\\]`pjlt';\\]`pjlt';\\]`pjlt';\\]`pjlt';\\]`pjlt';\\]`pjlt';\\]`pjlt';\\]`pjlt';\\]`pjlt';\\]`pjlt';\\]`pjlt';\\]`pjlt';\\]`pjlt';\\]`pjlt';\\]`pjlt';\\]`pjlt';\\]`pjlt';\\]`pjlt';\\]`pjlt';\\]`pjlt';\\]`pjlt';\\]`pjlt';\\]`pjlt';\\]`pjlt';\\]`pjlt';\\]`pjlt';\\]`pjlt';\\]`pjlt';\\]`pjlt';\\]`pjlt';\\]`pjlt';\\]`pjlt';\\]`pjlt';\\]`pjlt';\\]`pjlt';\\]`pjlt';\\]`pjlt';\\]`pjlt';\\]`pjlt';\\]`pjlt';\\]`pjlt';\\]`pjlt';\\]`pjlt';\\]`pjlt';\\]`pjlt';\\]`pjlt';\\]`pjlt';\\]`pjlt';\\]`pjlt';\\]`pjlt';\\]`pjlt';\\]`pjlt';\\]`pjlt';\\]`pjlt';\\]`pjlt';\\]`pjlt';\\]`pjlt';\\]`pjlt';\\]`pjlt';\\]`pjlt';\\]`pjlt';\\]`pjlt';\\]`pjlt';\\]`pjlt';\\]`pjlt';\\]`pjlt';\\]`pjlt';\\]`pjlt';\\]`pjlt';\\]`pjlt';\\]`pjlt';\\]`pjlt';\\]`pjlt';\\]`pjlt';\\]`pjlt';\\]`pjlt';\\]`pjlt';\\]`pjlt';\\]`pjlt';\\]`pjlt';\\]`pjlt';\\]`pjlt';\\]`pjlt';\\]`pjlt';\\]`pjlt';\\]`pjlt';\\]`pjlt';\\]`pjlt';\\]`pjlt';\\]`pjlt';\\]`pjlt';\\]`pjlt';\\]`pjlt';\\]`pjlt';\\]`pjlt';\\]`pjlt';\\]`pjlt';\\]`pjlt';\\]`pjlt';\\]`pjlt';\\]`pjlt';\\]`pjlt';\\]`pjlt';\\]`pjlt';\\]`pjlt';\\]`pjlt';\\]`pjlt';\\]`pjlt';\\]`pjlt';\\]`pjlt';\\]`pjlt';\\]`pjlt';\\]`pjlt';\\]`pjlt';\\]`pjlt';\\]`pjlt';\\]`pjlt';\\]`pjlt';\\]`pjlt';\\]`pjlt';\\]`pjlt';\\]`pjlt';\\]`pjlt';\\]`pjlt';\\]`pjlt';\\]`pjlt';\\]`pjlt';\\]`pjlt';\\]`pjlt';\\]`pjlt';\\]`pjlt';\\]`pjlt';\\]`pjlt';\\]`pjlt';\\]`pjlt';\\]`pjlt';\\]`pjlt';\\]`pjlt';\\]`pjlt';\\]`pjlt';\\]`pjlt';\\]`pjlt';\\]`pjlt';\\]`pjlt';\\]`pjlt';\\]`pjlt';\\]`pjlt';\\]`pjlt';\\]`pjlt';\\]`pjlt';\\]`pjlt';\\]`pjlt';\\]`pjlt';\\]`pjlt';\\]`pjlt';\\]`pjlt';\\]`pjlt';\\]`pjlt';\\]`pjlt';\\]`pjlt';\\]`pjlt';\\]`pjlt';\\]`pjlt';\\]`pjlt';\\]`pjlt';\\]`pjlt';\\]`pjlt';\\]`pjlt';\\]`pjlt';\\]`pjlt';\\]`pjlt';\\]`pjlt';\\]`pjlt';\\]`pjlt';\\]`pjlt';\\]`pjlt';\\]`pjlt';\\]`pjlt';\\]`pjlt';\\]`pjlt';\\]`pjlt';\\]`pjlt';\\]`pjlt';\\]`pjlt';\\]`pjlt';\\]`pjlt';\\]`pjlt';\\]`pjlt';\\]`pjlt';\\]`pjlt';\\]`pjlt';\\]`pjlt';\\]`pjlt';\\]`pjlt';\\]`pjlt';\\]`pjlt';\\]`pjlt';\\]`pjlt';\\]`pjlt';\\]`pjlt';\\]`pjlt';\\]`pjlt';\\]`pjlt';\\]`pjlt';\\]`pjlt';\\]`pjlt';\\]`pjlt';\\]`pjlt';\\]`pjlt';\\]`pjlt';\\]`pjlt';\\]`pjlt';\\]`pjlt';\\]`pjlt';\\]`pjlt';\\]`pjlt';\\]`pjlt';\\]`pjlt';\\]`pjlt';\\]`pjlt';\\]`pjlt';\\]`pjlt';\\]`pjlt';\\]`pjlt';\\]`pjlt';\\]`pjlt';\\]`pjlt';\\]`pjlt';\\]`pjlt';\\]`pjlt';\\]`pjlt';\\]`pjlt';\\]`pjlt';\\]`pjlt';\\]`pjlt';\\]`pjlt';\\]`pjlt';\\]`pjlt';\\]`pjlt';\\]`pjlt';\\]`pjlt';\\]`pjlt';\\]`pjlt';\\]`pjlt';\\]`pjlt';\\]`pjlt';\\]`pjlt';\\]`pjlt';\\]`pjlt';\\]`pjlt';\\]`pjlt';\\]`pjlt';\\]`pjlt';\\]`pjlt';\\]`pjlt';\\]`pjlt';\\]`pjlt';\\]`pjlt';\\]`pjlt';\\]`pjlt';\\]`pjlt';\\]`pjlt';\\]`pjlt';\\]`pjlt';\\]`pjlt';\\]`pjlt';\\]`pjlt';\\]`pjlt';\\]`pjlt';\\]`pjlt';\\]`pjlt';\\]`pjlt';\\]`pjlt';\\]`pjlt';\\]`pjlt';\\]`pjlt';\\]`pjlt';\\]`pjlt';\\]`pjlt';\\]`pjlt';\\]`pjlt';\\]`pjlt';\\]`pjlt';\\]`pjlt';\\]`pjlt';\\]`pjlt';\\]`pjlt';\\]`", "~~~~~~~~~~~~~~~~~~~~~~~~~~~~~~~~~~~~~~~~~~~~~~~~~~~~~~~~~~~~~~~~~~~~~~~~~~~~~~~~~~~~~~~~~~~~~~~~~~~~~~~~~~~~~~~~~~~~~~~~~~~~~~~~~~~~~~~~~~~~~~~~~~~~~~~~~~~~~~~~~~~~~~~~~~~~~~~~~~~~~~~~~~~~~~~~~~~~~~~~~~~~~~~~~~~~~~~~~~~~~~~~~~~~~~~~~~~~~~~~~~~~~~~~~~~~~~~~~~~~~~~~~~~~~~~~~~~~~~~~~~~~~~~~~~~~~~~~~~~~~~~~~~~~~~~~~~~~~~~~~~~~~~~~~~~~~~~~~~~~~~~~~~~~~~~~~~~~~~~~~~~~~~~~~~~~~~~~~~~~~~~~~~~~~~~~~~~~~~~~~~~~~~~~~~~~~~~~~~~~~~~~~~~~~~~~~~~~~~~~~~~~~~~~~~~~~~~~~~~~~~~~~~~~~~~~~~~~~~~~~~~~~~~~~~~~~~~~~~~~~~~~~~~~~~~~~~~~~~~~~~~~~~~~~~~~~~~~~~~~~~~~~~~~~~~~~~~~~~~~~~~~~~~~~~~~~~~~~~~~~~~~~~~~~~~~~~~~~~~~~~~~~~~~~~~~~~~~~~~~~~~~~~~~~~~~~~~~~~~~~~~~~~~~~~~~~~~~~~~~~~~~~~~~~~~~~~~~~~~~~~~~~~~~~~~~~~~~~~~~~~~~~~~~~~~~~~~~~~~~~~~~~~~~~~~~~~~~~~~~~~~~~~~~~~~~~~~~~~~~~~~~~~~~~~~~~~~~~~~~~~~~~~~~~~~~~~~~~~~~~~~~~~~~~~~~~~~~~~~~~~~~~~~~~~~~~~~~~~~~~~~~~~~~~~~~~~~~~~~~~~~~~~~~~~~~~~~~~~~~~~~~~~~~~~~~~~~~~~~~~~~~~~~~~~~~~~~~~~~~~~~~~~~~~~~~~~~~~~~~~~~~~~~~~~~~~~~~~~~~~~~~~~~~~~~~~~~~~~~~~~~~~~~~~~~~~~~~~~~~~~~~~~~~~~~~~~~~~~~~~~~~~~~~~~~~~~~~~~~~~~~~~~~~~~~~~~~~~~~~~~~~~~~~~~~~~~~~~~~~~~~~~~~~~~~~~~~~~~~~~~~~~~~~~~~~~~~~~~~~~~~~~~~~~~~~~~~~~~~~~~~~~~~~~~~~~~~~~~~~~~~~~~~~~~~~~~~~~~~~~~~~~~~~~~~~~~~~~~~~~~~~~~~~~~~~~~~~~~~~~~~~~~~~~~~~~~~~~~~~~~~~~~~~~~~~~~~~~~~~~~~~~~~~~~~~~~~~~~~~~~~~~~~~~~~~~~~~~~~~~~~~~~~~~~~~~~~~~~~~~~~~~~~~~~~~~~~~~~~~~~~~~~~~~~~~~~~~~~~~~~~~~~~~~~~~~~~~~~~~~~~~~~~~~~~~~~~~~~~~~~~~~~~~~~~~~~~~~~~~~~~~~~~~~~~~~~~~~~~~~~~~~~~~~~~~~~~~~~~~~~~~~~~~~~~~~~~~~~~~~~~~~~~~~~~~~~~~~~~~~~~~~~~~~~~~~~~~~~~~~~~~~~~~~~~~~~~~~~~~~~~~~~~~~~~~~~~~~~~~~~~~~~~~~~~~~~~~~~~~~~~~~~~~~~~~~~~~~~~~~~~~~~~~~~~~~~~~~~~~~~~~~~~~~~~~~~~~~~~~~~~~~~~~~~~~~~~~~~~~~~~~~~~~~~~~~~~~~~~~~~~~~~~~~~~~~~~~~~~~~~~~~~~~~~~~~~~~~~~~~~~~~~~~~~~~~~~~~~~~~~~~~~~~~~~~~~~~~~~~~~~~~~~~~~~~~~~~~~~~~~~~~~~~~~~~~~~~~~~~~~~~~~~~~~~~~~~~~~~~~~~~~~~~~~~~~~~~~~~~~~~~~~~~~~~~~~~~~~~~~~~~~~~~~~~~~~~~~~~~~~~~~~~~~~~~~~~~~~~~~~~~~~~~~~~~~~~~~~~~~~~~~~~~~~~~~~~~~~~~~~~~~~~~~~~~~~~~~~~~~~~~~~~~~~~~~~~~~~~~~~~~~~~~~~~~~~~~~~~~", "LabVIEWLabVIEWLabVIEWLabVIEWLabVIEWLabVIEWLabVIEWLabVIEWLabVIEWLabVIEWLabVIEWLabVIEWLabVIEWLabVIEWLabVIEWLabVIEWLabVIEWLabVIEWLabVIEWLabVIEWLabVIEWLabVIEWLabVIEWLabVIEWLabVIEWLabVIEWLabVIEWLabVIEWLabVIEWLabVIEWLabVIEWLabVIEWLabVIEWLabVIEWLabVIEWLabVIEWLabVIEWLabVIEWLabVIEWLabVIEWLabVIEWLabVIEWLabVIEWLabVIEWLabVIEWLabVIEWLabVIEWLabVIEWLabVIEWLabVIEWLabVIEWLabVIEWLabVIEWLabVIEWLabVIEWLabVIEWLabVIEWLabVIEWLabVIEWLabVIEWLabVIEWLabVIEWLabVIEWLabVIEWLabVIEWLabVIEWLabVIEWLabVIEWLabVIEWLabVIEWLabVIEWLabVIEWLabVIEWLabVIEWLabVIEWLabVIEWLabVIEWLabVIEWLabVIEWLabVIEWLabVIEWLabVIEWLabVIEWLabVIEWLabVIEWLabVI..."]]  # Expected Array
      w6 = bool[] [TRUE, FALSE]  # PAD Array
      w7 = string[] ["QWERTYDSA", "~~w", "abcd", "__dsa/.432", "$#", "pjlt';\\]`", "~", "LabVIEW"]  # String IN Array
      n2 = for {
        tunnel: [w17] -> w9 mode=indexing
        tunnel: w7 -> [w15]
        shift-right: [w16] -> w8
        shift-left: w10 -> [w18]
        tunnel: w6 -> [w14] mode=indexing
        n3 = for {
          tunnel: w15 -> [w31] mode=indexing
          tunnel: [w21] -> w17 mode=indexing
          shift-right: [w30] -> w16
          shift-left: w18 -> [w29]
          tunnel: w14 -> [w19]
          # "The loop has 2000 iterations to ensure that the passed data\ndoes not fit in U32 representation"
          n4 = for {
            N: 2000 -> [_]
            shift-right: [w36] -> w28
            shift-left: "" -> [w35]
            tunnel: w31 -> [w34]
            n5 = Concatenate Strings(w34, w35) -> (w36:string)
          }
          n6 = call-dynamic "Add Protection.vi"("error in (no error)"=w29, "Pad"=w19, "String in"=w28, "CRC-32 in"="CRC-32 in") -> ("error out"=w26:errorcluster, "String out"=w25:string, "CRC-32 out"=w24:refnum<class "CRC-32.lvclass">)  [unwired: 5 in]
          n7 = call-dynamic "Check Protection.vi"("error in (no error)"=w26, "String in"=w25, "CRC-32 in"=w24) -> ("error out"=w23:errorcluster, "Protection Error"=w22:errorcluster, "String out"=w21:string, "CRC-32 out"=→"CRC-32 out":refnum<class "CRC-32.lvclass">)  [unwired: 5 in]
          n8 = Merge Errors(w22, w23) -> (w30:errorcluster)
        }
      }
      n9 = call-dynamic "passIfEqual.vi"("error in (no error)"=w8, "y"=w9, "x"=w5, "TestCase in"=w11) -> ("error out"=w13:errorcluster, "TestCase out"=w12:refnum<class "Instrument Addon Protections Unit Tests.lvclass">)  [unwired: 6 in]
    }
    frame Disabled {
      # "skip test result while test is under development"
      n10 = call <vilib>:"skip.vi"("error in (no error)"=w37, "TestCase in"=w40) -> ("error out"=w39:errorcluster, "TestCase out"=w38:refnum<class "Instrument Addon Protections Unit Tests.lvclass">)  [unwired: 8 in]
    }
  }
  "error out" <- w3
  "TestCase out" <- w1
